vi "main.vi"() -> ()   [LabVIEW 2024]
doc: "Use this template to build a producer/consumer design pattern with events to produce queue items. Use this design pattern instead of the User Interface Event Handler pattern for user interfaces when you want to execute code asynchronously in response to an event without slowing the user interface responsiveness."
uses:
  controls/type.eng.settings.ctl
  controls/UiStepBuilder.ctl
  controls/type.step-builder.ctl
  controls/UiProcHeader.ctl
  controls/Ui.nrt.flow-panel.ctl
  controls/UiNutritionFlowElement.ctl
  controls/UiScheduleTimestamp.ctl
  controls/typeEnv.ctl
  controls/type.StepFunction.ctl
  controls/typeXyPoint.ctl
  controls/type.address.ctl
  controls/enum.io.type.ctl
  controls/enum.io.mode.ctl
  controls/IONode.ctl
  controls/type-io-map-do.ctl
  controls/type-io-map-di.ctl
  controls/type-io-map-ai.ctl
  controls/type-snapshot.ctl
  controls/enum-io-sort-type.ctl
  controls/wind-dir-view.ctl
  controls/windows-panel.ctl
  controls/irr-panel.ctl
  controls/pbr-func-def.ctl
  controls/eng-serial-log.ctl
  controls/cluster-com-log.ctl
  controls/state-engine.ctl
  controls/state-logger.ctl
  controls/enum.io-interface.ctl
  controls/enum-com-log.ctl
  controls/enum-q-sched.ctl
  controls/enum.report-filter.ctl
  controls/typePathSelector.ctl
  controls/ini-key.ctl
  controls/typeProcVarientName.ctl
  controls/UiNutritionPanel.ctl
  controls/enumVarCtrlIO.ctl
  controls/type.eng-call.proc-insert.ctl
  controls/type.eng.proc.isrunning.ctl
  controls/eng-call-do-by-name.ctl
  controls/cluster-q-sched.ctl
  <vilib>/Utility/error.llb/DialogType.ctl
  <vilib>/Utility/miscctls.llb/LVPointTypeDef.ctl
  <vilib>/Utility/miscctls.llb/LVDateTimeRec.ctl
  controls/rio-rx-enum.ctl
  controls/type.eng.log-cluster.ctl
  controls/typeCmdPostStepFunc.ctl
  controls/typeEngineLogCluster.ctl
  VIs/Polymorphics/variantCtrlString.vi
  VIs/proc.util.validateParamExist.vi
  <vilib>/Utility/error.llb/Trim Whitespace.vi
  <vilib>/Utility/error.llb/Trim Whitespace One-Sided.vi
  globals/globals-engine.vi
  <vilib>/Utility/libraryn.llb/Create Directory Recursive.vi
  <vilib>/Utility/config.llb/Read Key (String).vi
  VIs/util.error.create.vi
  <vilib>/Utility/config.llb/Read Key (Double).vi
  <vilib>/Utility/config.llb/Read Key (I32).vi
  VIs/util-address-builder.vi
  VIs/util.DO.ToString.vi
  VIs/Polymorphics/io.command-builder.vi
  VIs/Polymorphics/io.command-builder.DO.vi
  VIs/Polymorphics/io.command-builder.AI.vi
  VIs/Polymorphics/io.command-builder.DI.vi
  <vilib>/Utility/config.llb/Write Key (String).vi
  <vilib>/Utility/config.llb/Write Key (Double).vi
  <vilib>/Utility/config.llb/Write Key (I32).vi
  controls/typeIniFileSection.ctl
  <vilib>/Utility/file.llb/Read Delimited Spreadsheet (DBL).vi
  <vilib>/Utility/config.llb/NI_LVConfig.lvlib
  <vilib>/Instr/_visa.llb/VISA Find Search Mode.ctl
  <vilib>/Utility/file.llb/Write Delimited Spreadsheet (DBL).vi
panel:
  out "clock 3":string="12:34:56"
  out "COM Size":i64 format="IOs: %d"
  out "COM FIFO":i32 format="QCom: %d"
  out "LOG FIFO 2":i32 format="QLog: %d"
  out "ENG FIFO 2":i32 format="QEng: %d"
  in  "Cluster":cluster{"MAIN":bool, "I/O":bool, "ADMIN":bool}
  out "DayNight":bool
  in  "ENG ms ctrl 28":i32=300 caption="Runtime Interval" format="Runtime:  %d [ms]"
  in  "ENG ms ctrl 15":i32=300 caption="Runtime Interval" format="Runtime:  %d [ms]"
  in  "ENG ms ctrl 14":i32=300 caption="Runtime Interval" format="Runtime:  %d [ms]"
  in  "ENG ms ctrl 13":i32=300 caption="Runtime Interval" format="Runtime:  %d [ms]"
  in  "ENG ms ctrl 12":i32=300 caption="Runtime Interval" format="Runtime:  %d [ms]"
  in  "ENG ms ctrl 11":i32=300 caption="Runtime Interval" format="Runtime:  %d [ms]"
  in  "ENG ms ctrl 10":i32=300 caption="Runtime Interval" format="Runtime:  %d [ms]"
  in  "ENG ms ctrl 9":i32=300 caption="Runtime Interval" format="Runtime:  %d [ms]"
  in  "ENG ms ctrl 8":i32=300 caption="Runtime Interval" format="Runtime:  %d [ms]"
  in  "Admin Panel":bool
  out "Waveform Chart":dbl(graph)
  out "User messages":string
  out "error out":errorcluster
  in  "Timer Reset?":bool
  out "userName":string="USER"
  out "projectName":string="NAME"
  in  "ENV":T1=enum."ENV.TEST.SINGLE-02"
  out "clock":string="12:34:56"
  in  "Enable Report":bool
  in  "Tab Control 2":T2(tab)
  in  "EngLogClear":bool
  out "Collected Reports":string
  out "Collected Reports 2":string
  in  "VISA REPORT":T4={"visa report"=[["Range", "High", "Low", "25", "FULL"], ["", "", "", "", ""], ["", "", "", "", ""], ["", "", "", "", ""], ["", "", "", "", ""], ["", "", "", "", ""], ["", "", "", "", ""], ["", "", "", "", ""], ["", "", "", "", ""]], "RIO Address"=0, "IOtype"=enum."AI", "VISA Report En"=FALSE, "Clear"=FALSE, "Only Errors?"=FALSE} {"RIO Address" min=-1 max=31 step=1 format="RIO: %02d"}
  out "SelectedPath":path
  out "case":T5
  in  "Clk Simulator":timestamp format="%<%x %.1X>T"
  in  "Simulate Clock Reset":bool
  out "Clock Simulation":bool
  in  "Time Addition":dbl
  out "AI":dbl[][](array[numeric]) format="%#.1f"
  in  "Calib?":bool
  out "SCHED":i32 format="%.3p"
  out "Waveform Chart 3":dbl(graph)
  out "GuiLog":i32 format="%#.3p"
  out "Eng":i32 format="%#.3p"
  out "Event":i32 format="%#.3p"
  out "ComLog":i32 format="%.3p"
  out "Schedulers":cluster{"Proc Name":string, "Time":timestamp}[](array[cluster]) {"Time" format="%<%H:%M:%S>T"}
  out "Report General":T7(array[cluster]) {"clk" format="%#.1f"}
  in  "Log Clear":bool
  in  "Proc Name":string(combo)
  in  "DO Set by Addr":T9 {"ADDR" format="%04d"}
  in  "DO Set by Name":T10={"State"=FALSE, "Name"="Name...", "Timeout [s]"=8, "Send"=FALSE}
  in  "SerialPort":refnum<visa-resource-name>="COM12"
  in  "MenuRuntime":T11={"Run"=FALSE, "Step"=FALSE, "Load"=FALSE, "Status"=FALSE, "Unload"=FALSE, "Reload"=FALSE, "Stop"=FALSE, "ProcedureReload"=FALSE, "ProcedureStep"=FALSE, "ProcedureSelect"="set-dout", "ProcedureRun"=FALSE}
  out "Simulated":string[](array[string])
  in  "ProjectSettings":T12={"Project Name"="Yogiland", "Latitude"=0.0, "Longitude"=0.0, "TimeZone"=0, "userName"="Yogiland"} {"Longitude" format="%#.6g"; "Latitude" format="%#.6g"}
  out "RIO Snapshots":T13[](array[typedef]) {"Dports" format="%08x"}
  in  "Tab Main":enum32{"MAIN", "I/O", "ADMIN"}(tab)
  in  "Button":bool
  in  "Section":string(combo)
  in  "Tab NTR":T14(tab)
  in  "NTR Flowchart":T15={"WASH_IN"={"boolean"=FALSE, "Message"="25/150"}, "EC"={"boolean"=TRUE, "Message"="L Alarm"}, "PH"={"boolean"=TRUE, "Message"="Low"}, "ORP"={"boolean"=TRUE, "Message"="Range"}, "W_TEMP"={"boolean"=TRUE, "Message"="25"}, "W_LEVEL"={"boolean"=TRUE, "Message"="FULL"}, "ALFA1"={"boolean"=TRUE, "Message"="60/60"}, "BETA1"={"boolean"=TRUE, "Message"="25/60"}, "ALFA2"={"boolean"=FALSE, "Message"="0/0"}, "BETA2"={"boolean"=FALSE, "Message"="0/0"}, "ACID"={"boolean"=FALSE, "Message"="0/60"}, "BASE"={"boolean"=FALSE, "Message"="0/50"}, "WATER"={"boolean"=FALSE, "Message"="0/150"}, "WASH_OUT"={"boolean"=FALSE, "Message"="ss"}, "UNIT"={"boolean"=FALSE, "Message"="0"}, "ORPMIX"={"boolean"=FALSE, "Message"="0/150"}}
  out "ntr.status-table":string[][](table)=[["Range", "High", "Low", "25", "FULL"], ["", "", "", "", ""], ["", "", "", "", ""], ["", "", "", "", ""], ["", "", "", "", ""], ["", "", "", "", ""], ["", "", "", "", ""], ["", "", "", "", ""], ["", "", "", "", ""]]
  out "NTR Status":string="Nutrition Status: Processing Unit "
  in  "ntrGraphPeriod":T18 {"lastDays" format="Last %d Days"; "Time range"."Start" format="From: %<%d/%m/%y>T"; "Time range"."End" format="To: %<%d/%m/%y>T"}
  out "Nutrition Sensor Graph":cluster{"X":dbl[], "Y":dbl[]}(graph)
  out "EC 3":cluster{"X":dbl[], "Y":dbl[]}(graph)
  in  "ntrDosepumpSelect":string(combo)
  in  "ntrInputSelect":string(combo)
  in  "Irrigation status":string="Irrigation Status"
  out "Solar Elevation Graph":waveform(dbl)(graph)
  in  "UiProjectSettings":T19 {"Longitude" format="%#.6g"; "Latitude" format="%#.6g"}
  in  "GoToCam 2":bool
  in  "GoToCam":bool
  in  "Cluster 2":T20
  in  "camera":u16(ring) items=["Camera 1", "Camera 2"]
  in  "start":T17 caption="Open" format="%<%H:%M>T"
  out "last":T17 caption="Open" format="Last Harvest %<%H:%M:%S %d/%m/%y>T"
  in  "PRBmenu":cluster{"Harvest":bool, "SANI":bool}
  in  "PbrView 2":T21 {"Unit Storage"."col" scale=0.0..1.0; "Unit Storage"."?" scale=0.0..1.0; "Unit Storage"."?" scale=0.0..1.0; "Unit Column"."col" scale=0.0..1.0; "Unit Column"."?" scale=0.0..1.0; "Unit Column"."?" scale=0.0..1.0; "Digester"."Digester 2" scale=0.0..10.0; "Digester"."Digester 1" scale=0.0..10.0; "BIO Mass Tank" scale=0.0..100.0; "Harvest\n Tank" scale=0.0..100.0}
  in  "pbr-proc-mode":enum16{"MANUAL", "AUTO"}(ring)
  in  "PBR Builder":T23(array[cluster])
  out "source":string
  in  "PBR_PLAY":cluster{"PLAY":bool, "PAUSE":bool, "STOP":bool}
  in  "PBR PROC":string(combo)
  in  "PBR":T24
  in  "Graph Panel":T25={"Time range"={"Start"=timestamp(0 s since 1904-01-01), "End"=timestamp(0 s since 1904-01-01)}, "lastDays"=3, "refresh"=FALSE} {"lastDays" min=1 max=99 step=1 format="%d Days"; "Time range"."Start" format="From: %<%d/%m/%y>T"; "Time range"."End" format="To: %<%d/%m/%y>T"}
  out "OutdoorStatus":T26
  out "indoorStatus":T27
  in  "Tab Control 3":T28(tab)
  out "Outdoor Tdry Graph":cluster{"X":dbl[], "Y":dbl[]}[](graph)
  out "RH":cluster{"X":dbl[], "Y":dbl[]}[](graph)
  out "UV Graph":cluster{"X":dbl[], "Y":dbl[]}(graph)
  in  "UVAccHistoryDays":i8=3
  out "UV_ACC":cluster{"X":dbl[], "Y":dbl[]}(graph)
  out "Waveform Chart 2":cluster{dbl, "UV Limit":dbl}(graph)
  in  "UvAccRefresh":bool
  out "WindSpeed":cluster{"X":dbl[], "Y":dbl[]}(graph)
  out "Wind Dir Panel":T29
  out "UV Acc.":dbl format="%#_3p"
  in  "Tab Auxi":T30(tab)
  in  "IRR Params":T31={"Day Time"={"Sunset"=timestamp(0 s since 1904-01-01), "Sunrise"=timestamp(0 s since 1904-01-01)}, "timeLimits"={"Irrigation"=0.0, "Nut./Water"=0.0}, "Calculated Timing"={"Irrigation Timeout"=timestamp(0 s since 1904-01-01), "Nutrients Timeout"=timestamp(0 s since 1904-01-01)}, "Irr Dosing Time"={"Nutrients"=0, "Water"=0, "Wash"=0}, "UV Limit "=0.0, "Dose Table"=[{"Enable"=FALSE, "output"="IRR_SEC1"}, {"Enable"=FALSE, "output"="IRR_SEC2"}, {"Enable"=FALSE, "output"="IRR_SEC3"}, {"Enable"=FALSE, "output"="IRR_SEC4"}, {"Enable"=FALSE, "output"="IRR_SEC5"}, {"Enable"=FALSE, "output"="IRR_SEC6"}], "Last Iteration"=timestamp(0 s since 1904-01-01), "UV Reduction Status"=FALSE, "UV Reduction"=0} {"UV Reduction" max=99 step=1 format="%d [%%]"; "timeLimits"."Nut./Water" format="%02.2f [hr]"; "timeLimits"."Irrigation" format="%02.2f [hr]"; "Day Time"."Sunrise" format="%<%H:%M:%S>T"; "Day Time"."Sunset" format="%<%H:%M:%S>T"; "Calculated Timing"."Nutrients Timeout" format="%<%H:%M:%S>T"; "Calculated Timing"."Irrigation Timeout" format="%<%H:%M:%S>T"; "UV Limit" format="%#.1p [J/m2]"; "Irr Dosing Time"."Wash" format="%d [s]"; "Irr Dosing Time"."Water" format="%d [s]"; "Irr Dosing Time"."Nutrients" format="%d [s]"; "Last Iteration" format="%<%X %x>T"}
  in  "WinView":T32 {"EastSideView" scale=0.0..100.0; "WestSideView" scale=0.0..8.0; "EastPosition" max=12; "WestPosition" max=12}
  in  "AuxiliaryList":T33(array[cluster]) {"Period" format="Period [s]: %d"; "Pulse" format="Pulse [s]: %d"}
  in  "NTR Panel":cluster{"CloseAll":bool}
  in  "RFS Enable Table":bool
  in  "RFS Enable Table":T34
  in  "RFS Cycles Set":bool
  in  "RFS Cycles":u16
  out "RFS Cycles":u16
  in  "RFS Cycles Get":bool
  out "RFS Status":string
  in  "RFS SetX1":bool
  in  "TableIndex":u8 max=7 step=1 format="Table: %d"
  in  "RFS SetX8":bool
  in  "RFS Delays":T35
  in  "RFS Address":u8 format="Address: %d"
  out "RFS Cycles Table":T36
  out "elements":cluster{"case":T5, "data":variant}[](array[cluster])
  in  "Tab IO":enum32{"Map", "Editor", "Calibration"}(tab)
  in  "Clear Virtuals":bool
  in  "IO Map Take Snapshot":bool caption="Take Snapshop"
  out "RIO List":cluster{"Address":u8, "Connected":bool}[](array[cluster]) {"Address" format="%02d"}
  in  "Show Undefined":bool
  out "IO Map AI Count":i32
  out "IO Map DI Count":i32
  out "IO Map DO Count":i32
  in  "IO Map DO":T37[](array[typedef]) caption="Digital Outputs" {"ADDR" format="%04d"}
  in  "IO Map AI":T39[](array[typedef]) caption="Analog Inputs" {"ADDR" format="%04d"}
  in  "IO Map DI":T40[](array[typedef]) caption="Digital Inputs" {"ADDR" format="%04d"}
  in  "IO Map Snapshot Enable":bool caption="Auto Snapshop Enable"
  in  "IO Search Map":T41={"By Name"="", "By Tag"="Tags...", "By Address"=0} caption="Search by Name | Tag | Address" {"By Address" min=-1 max=31 step=1 format="RIO: %02d"}
  in  "IO Search Map Refresh":bool
  in  "TimerSec":dbl=5.0 format="%#.1f"
  out "downcount[sec]":dbl format="%#.1g"
  in  "Simulators":cluster{"Input ":string, "Value":string}[](array[cluster])
  in  "IO Map VL":T42[](array[typedef]) caption="Virtual Channels" {"calibration"."Y" format="%#.3f"; "calibration"."X" format="%#.3f"; "ADDR" format="%04d"}
  out "IO Map VL Count":i32
  in  "IO Conf view":enum16{"Show All", "Search"}(ring)
  in  "IOconf Sort":T44
  in  "IO Search Conf":T45={"ADDR"=-1, "Label"="", "Type"=enum."Type", "Mode"=enum."Mode", "Tags"=""} {"ADDR" min=-1 max=99 format="RIO: %02d"}
  in  "IO Conf":T46(array[cluster]) {"calibration"."Y" format="%#.3f"; "calibration"."X" format="%#.3f"; "ADDR" format="%04d"}
  in  "IO List":cluster{"save":bool, "loadCsv":bool}
  in  "New Element":T42={"ADDR"=0, "Label"="Name", "Type"=enum."DI", "Mode"=enum."RIO", "Value"="Value", "Tags"="Tags", "calibration"=[]} {"calibration"."Y" format="%#.3f"; "calibration"."X" format="%#.3f"; "ADDR" format="%04d"}
  in  "IO Add New":bool
  out "size":i32 format="Count: %d"
  out "Value (Y)":dbl
  out "Raw (X)":dbl
  in  "IO calib save":bool
  in  "IO calib select":string(combo)
  in  "XyPairs":T43[](array[typedef]) {"Y" format="%#.3f"}
  out "error":errorcluster
  out "Chart":cluster{"unCalibrated":u16, "Value out":dbl}(graph)
  in  "Tab Control":enum32{"Builder", "Snapshot", "Settings"}(tab)
  in  "BuilderMenu":T47
  in  "UiBuildProcHead":T48={"Procedure Name"="MyProcExample", "Running"=TRUE, "tags"="MyProcExample"}
  in  "Loaded Proc Path":string[](array[string])
  in  "UiBuildSteps":T49[](array[typedef])
  in  "File path":path
  out "UiBuildSteps 2":T49[](array[typedef])
  in  "Proc Select 2":string(combo)
  out "Serial Log Size":i32
  out "COM Snapshot":T51[](array[typedef])
  in  "Snapshot Size":i64=1000
  in  "COM":bool
  in  "filter":T52={"Status"=0, "Date"="", "Caller"="", "Type"="", "IOname"="", "Calib"="", "Uncalib"="", "Vsdt"="Vsdt", "StatusMsg"=""}
  out "Serial Record(s)":T53[](array[typedef]) {"IOnode"."calibration"."Y" format="%#.3f"; "IOnode"."calibration"."X" format="%#.3f"; "IOnode"."ADDR" format="%04d"}
  out "App Started at":timestamp format="%<%x %.3X>T"
  out "Loaded":cluster{"Procedure":variant[]}[](array[cluster]) caption="Loaded Procedures"
  in  "ENG ms":i32=-1 caption="Interval"
  in  "Title Bar Visible":bool
  in  "ENG ms ctrl":i32=300 caption="Runtime Interval" format="Runtime:  %d [ms]"
  in  "EVENT ms":i32=100 format="%d [ms]"
  out "Type":u8 format="%.0x"
  out "Address":u8 format="%.0x"
  in  "read buffer":string
  out "Command Payload":string
  out "AI uncalib out":u16
  out "AI out":dbl
  out "Data Size":u8
  out "GUI Engine Errors":errorcluster[](array[cluster])
  out "Record Engine Errors":errorcluster[](array[cluster])
  out "VM Engine Errors":errorcluster[](array[cluster])
  out "Scheduler Engine Errors":errorcluster[](array[cluster])
  # "Outoor"
  # "Indoor"
  # "UV Accumulator"
  # "Nutrition"
  # "Nutrition History"
  # "Nursery"
  # "Camera Robot"
  # "PBR"
  # "- Fully Open"
  # "- Fully Close"
  # "W"
  # "E"
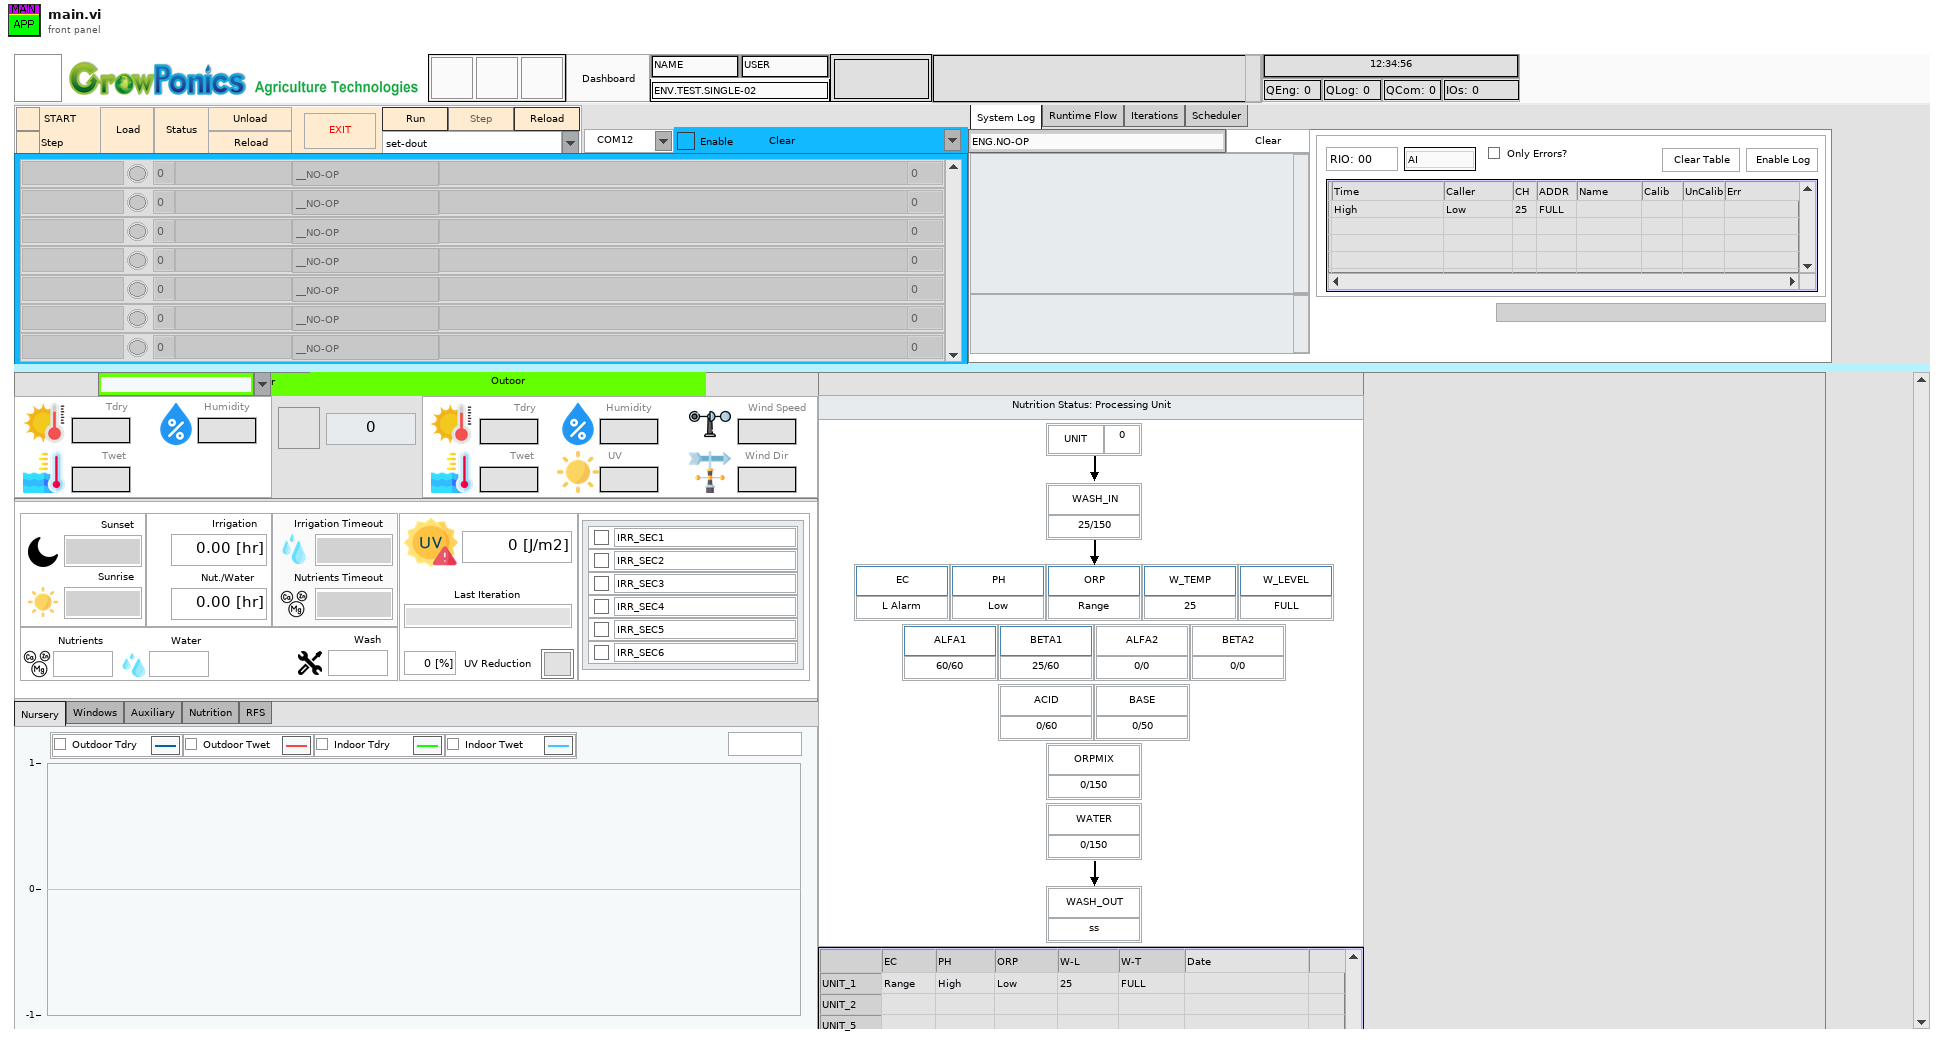
[diagram p1: front panel]
types:
  T1 = typedef "typeEnv.ctl" = enum16{"ENV.PRODUCTION", "ENV.TEST.NO-HW", "ENV.TEST.SINGLE-01", "ENV.TEST.SINGLE-02", "ENV.TEST.SINGLE-02 AI 0", "ENV.TEST.SINGLE-03"}
  T2 = enum32{"System Log", "Runtime Flow", "Iterations", "Scheduler"}
  T3 = typedef "enum.io.type.ctl" = enum16{"Type", "DI", "DO", "AI", "AO", "VL", "BUF"}
  T4 = cluster{"visa report":string[][], "RIO Address":i32, "IOtype":T3, "VISA Report En":bool, "Clear":bool, "Only Errors?":bool}
  T5 = typedef "state-engine.ctl" = enum16{"ENG.NO-OP", "ENG.START", "ENG.STOP", "ENG.EXECUTE", "ENG.STATUS", "ENG.EXTERNAL-CALL", "ENG.INIT", "ENG.INIT.VARS", "ENG.INIT.SERIAL", "ENG.LOAD", "ENG.LOAD.SINGLE", "ENG.LOAD.MODULE", "ENG.LOAD.RELOAD", "ENG.LOAD.UNLOAD", "ENG.IO.LOAD", "ENG.IO.SAVE", "ENG.PROC.RELOAD-BY-NAME", "ENG.PROC.START", "ENG.PROC.STOP", "ENG.PROC.INSERT-STEPS", "ENG.PROC.ISRUNNING", "ENG.PROC.PRESET", "ENG.PROC.STATUS", "ENG.PRINT-USER-MSG", "ENG.RIO.SNAPSHOT", "ENG.RIO.AIN-SNAPSHOT-CALIB", "ENG.RIO.DOUT-BY-ADDR", "ENG.RIO.DOUT-BY-NAME", "ENG.RIO.RFS-DELAY-SET-X1", "ENG.RIO.RFS-DELAY-SET-X8", "ENG.RIO.RFS-CYCLES-SET", "ENG.RIO.RFS-CYCLES-GET", "ENG.RIO.RFS-ENABLE", "ENG.EXIT"}
  T6 = typedef "type.StepFunction.ctl" = enum16{"__NO-OP", "_DELAY_LOAD", "_DELAY_COMPARE", "_JUMP", "_COMPLETE", "_COMPARE", "_LOG_MESSAGE", "_LOG_LAST_REPORT", "_SCHEDULE", "_SCHEDULE_DAILY", "CLK_COMPARE", "PROC_START", "PROC_STOP", "PROC_LOAD", "PROC_COMPLETION_CHECK", "PROC_COMPLETION_LOAD", "_IO_READ", "_IO_READ_MANY", "_IO_WRITE", "_IO_WRITE_BY_REG", "_IO_GET_OUTPUT", "_OCS_CHECK", "_OCS_RECORD", "_GET_RH", "_GET_ACC_UV", "_GET_WD", "_GET_WS", "_REC_DELETE", "_REC_MOVE", "_REC_COPY", "_IRR_CHECK", "UNIT_CHECK", "UNIT_SAMPLE", "UNIT_DOSE"}
  T7 = cluster{"ErrorFlag":bool, "idx":i32, "Step Name":string, "Step Function":T6, "Report":string, "clk":dbl, "Step Name 2":string}[]
  T8 = typedef "type.address.ctl" = u16
  T9 = cluster{"State":bool, "ADDR":T8, "Timeout [s]":u8, "Send":bool}
  T10 = cluster{"State":bool, "Name":string, "Timeout [s]":u8, "Send":bool}
  T11 = cluster{"Run":bool, "Step":bool, "Load":bool, "Status":bool, "Unload":bool, "Reload":bool, "Stop":bool, "ProcedureReload":bool, "ProcedureStep":bool, "ProcedureSelect":string, "ProcedureRun":bool}
  T12 = typedef "type.eng.settings.ctl" = cluster{"Project Name":string, "Latitude":dbl, "Longitude":dbl, "TimeZone":i32, "userName":string}
  T13 = typedef "type-snapshot.ctl" = cluster{"Address":u8, "DI":bool[], "status":errorcluster, "AI":dbl[], "Dports":u32, "AI RAW":dbl[]}
  T14 = enum32{"Nutrition Flow", "Nutrition", "Nursery Status", "Camera", "PBR", "PBR Programming"}
  T15 = typedef "Ui.nrt.flow-panel.ctl" = cluster{"WASH_IN":T16, "EC":T16, "PH":T16, "ORP":T16, "W_TEMP":T16, "W_LEVEL":T16, "ALFA1":T16, "BETA1":T16, "ALFA2":T16, "BETA2":T16, "ACID":T16, "BASE":T16, "WATER":T16, "WASH_OUT":T16, "UNIT":cluster{"boolean":bool, "Message":string}, "ORPMIX":T16}
  T16 = typedef "UiNutritionFlowElement.ctl" = cluster{"boolean":bool, "Message":string}
  T17 = typedef "UiScheduleTimestamp.ctl" = timestamp
  T18 = cluster{"Time range":cluster{"Start":T17, "End":T17}, "lastDays":dbl, "refresh":bool}
  T19 = cluster{"Latitude":dbl, "Longitude":dbl, "TimeZone":i32}
  T20 = cluster{"Next Button":bool, "Previous Button":bool, "Up Button":bool, "Down Button":bool, "Home":bool}
  T21 = cluster{"Unit Storage":cluster{dbl, dbl, "col":dbl}, "Unit Column":cluster{dbl, dbl, "col":dbl}, "Ui_TANKOUT":bool, "Column":dbl, "Ui MAIN\nUi_COLOUT\nUi_PUMP":bool, "Digester":cluster{"Digester 1":dbl, "Digester 2":dbl}, "DO 4":bool, "Flow Out DI":bool, "BIO Mass Tank":dbl, "DO Membrane":bool, "MEDIUM":bool, "WATER":bool, "Ui_TANKIN":bool, "Harvest\n Tank":dbl, "HARVEST":bool}
  T22 = typedef "pbr-func-def.ctl" = enum16{"DELAY SEC", "SCHEDULE DAILY", "SENSE", "PROC START", "SET OUTPUT", "FINISH", "JUMP"}
  T23 = cluster{"Operation":T22, "Param":string, "uid":string}[]
  T24 = cluster{"LOAD":bool, "SAVE":bool, "COMPILE":bool, "SAVEAS":bool}
  T25 = cluster{"Time range":cluster{"Start":T17, "End":T17}, "lastDays":i8, "refresh":bool}
  T26 = cluster{"Tdry":string, "Twet":string, "UV":string, "Humidity":string, "Wind Speed":string, "Wind Direction":string}
  T27 = cluster{"Tdry":string, "Twet":string, "Humidity":string}
  T28 = enum32{"Temperature", "Humidity", "UV", "UV Acc", "Wind"}
  T29 = typedef "wind-dir-view.ctl" = cluster{"SE":bool, "SW":bool, "NE":bool, "NW":bool, "W":bool, "E":bool, "S":bool, "N":bool}
  T30 = enum32{"Nursery", "Windows", "Auxiliary", "Nutrition", "RFS"}
  T31 = typedef "irr-panel.ctl" = cluster{"Day Time":cluster{"Sunset":timestamp, "Sunrise":timestamp}, "timeLimits":cluster{"Irrigation":dbl, "Nut./Water":dbl}, "Calculated Timing":cluster{"Irrigation Timeout":timestamp, "Nutrients Timeout":timestamp}, "Irr Dosing Time":cluster{"Nutrients":u16, "Water":u16, "Wash":u16}, "UV Limit ":dbl, "Dose Table":cluster{"Enable":bool, "output":string}[], "Last Iteration":timestamp, "UV Reduction Status":bool, "UV Reduction":u8}
  T32 = typedef "windows-panel.ctl" = cluster{"EastPosition":u16, "WestPosition":u16, "Wind Direction":string, "CloseAll":bool, "WestSideView":u16, "EastSideView":u16, "Wind Speed":string, "confs":cluster{"Full Open [sec]":u16, "Full Close [sec]":u16, "Stages":u16}}
  T33 = cluster{"Source":string, "SourceStatus":bool, "Dest":string, "DestStatus":bool, "Pulse":u16, "Period":u16, "Proc Name":string}[]
  T34 = cluster{"[0]":bool, "[1]":bool, "[2]":bool, "[3]":bool, "[4]":bool, "[5]":bool, "[6]":bool, "[7]":bool}
  T35 = cluster{"Delay Y":u8, "Delay X1":u8, "Delay X2":u8, "Delay CT":u8}
  T36 = cluster{"[0]":u16, "[1]":u16, "[2]":u16, "[3]":u16, "[4]":u16, "[5]":u16, "[6]":u16, "[7]":u16}
  T37 = typedef "type-io-map-do.ctl" = cluster{"ADDR":T8, "Label":string, "Mode":T38, "Value":string, "State":bool}
  T38 = typedef "enum.io.mode.ctl" = enum16{"Mode", "RIO", "SIM"}
  T39 = typedef "type-io-map-ai.ctl" = cluster{"ADDR":T8, "Label":string, "Mode":T38, "Value":string}
  T40 = typedef "type-io-map-di.ctl" = cluster{"ADDR":T8, "Label":string, "Mode":T38, "State":bool, "Value":string}
  T41 = cluster{"By Name":string, "By Tag":string, "By Address":i32}
  T42 = typedef "IONode.ctl" = cluster{"ADDR":T8, "Label":string, "Type":T3, "Mode":T38, "Value":string, "Tags":string, "calibration":T43[]}
  T43 = typedef "typeXyPoint.ctl" = cluster{"X":dbl, "Y":dbl}
  T44 = typedef "enum-io-sort-type.ctl" = enum16{"Sort By Address", "Sort By Name"}
  T45 = cluster{"ADDR":i8, "Label":string, "Type":T3, "Mode":T38, "Tags":string}
  T46 = cluster{"ADDR":T8, "Label":string, "Type":T3, "Mode":T38, "Value":string, "Tags":string, "calibration":T43[]}[]
  T47 = cluster{"templateSave":bool, "templateLoad":bool, "procedureLoad":bool, "procedureSaveAs":bool, "procedureSave":bool, "procedureReload":bool}
  T48 = typedef "UiProcHeader.ctl" = cluster{"Procedure Name":string, "Running":bool, "tags":string}
  T49 = typedef "UiStepBuilder.ctl" = cluster{"Step Function":T50, "ParamString":string, "Step Label":string}
  T50 = typedef "type.step-builder.ctl" = enum16{"NO_OPERATION", "DELAY-JUMP", "DELAY", "JUMP", "COMPLETE", "SCHEDULER", "SCHEDULER_DAILY", "IRR-CHECK", "UNIT-CHECK", "UNIT-SAMPLE", "UNIT-DOSE", "LOG-REPORT", "LOG-MESSAGE", "IO-READ", "IO-READ-MANY", "IO-WRITE", "IO-COMPARE-OUT", "IO-COMPARE-IN", "PROC-START", "PROC-STOP", "PROC-LOAD", "PROC-IS-COMPLETED", "RECORD-MOVE", "GET-RH", "GET-UV", "GET-WD", "GET-WS", "OCS-CHECK", "OCS-RECORD"}
  T51 = typedef "eng-serial-log.ctl" = cluster{"Status":u32, "Date":string, "Caller":string, "Type":string, "IOname":string, "Calib":string, "Uncalib":string, "Vsdt":string, "StatusMsg":string}
  T52 = cluster{"Status":u32, "Date":string, "Caller":string, "Type":string, "IOname":string, "Calib":string, "Uncalib":string, "Vsdt":string, "StatusMsg":string}
  T53 = typedef "cluster-com-log.ctl" = cluster{"Caller":string, "IOnode":T42, "error":errorcluster, "dports":bool[], "AIN (calib)":dbl, "AIN (raw)":u16, "Times Stamp":timestamp, "Record File Path":path, "Visa Data":string}
  T54 = typedef "enum-q-sched.ctl" = enum16{"SCHED.INIT", "SCHED.REGISTER", "SCHED.EXIT"}
  T55 = typedef "enum-com-log.ctl" = enum16{"REC.NO_OP", "REC.INIT", "REC.EXIT", "REC.SERIAL", "REC.IO", "REC.FETCH", "REC.OPEN-FILE", "REC.REOPEN-FILE"}
  T56 = typedef "enum.io-interface.ctl" = enum16{"IO_VISA_WR-RD", "IO_VISA_OPEN", "IO_VISA_CLOSE", "IO_VISA_CLEAR"}
  T57 = typedef "state-logger.ctl" = enum16{"LOG.NO_OP", "LOG.INIT", "LOG.INIT.NTR-FLOW", "LOG.EXIT", "LOG.CATCH", "LOG.PARSE.OCS", "LOG.UPDATE.SELECTORS", "LOG.UPDATE.IRR", "LOG.SNAPSHOT.PROC", "LOG.SNAPSHOT"}
  T58 = enum32{"Invalid", "Standard", "Closed", "Hidden", "Minimized", "Maximized"}
  T59 = typedef "ini-key.ctl" = enum16{"INI.PROJECT_NAME", "INI.ENV", "INI.ENG.SERIAL", "INI.ENG.INTERVAL_MS", "INI.LOCAL.LONGITUDE", "INI.LOCAL.LATITUDE", "INI.LOCAL.TIMEZONE"}
  T60 = typedef "typePathSelector.ctl" = enum16{"DIR_PROCS", "DIR_CONFIG", "DIR_TEMPLATE", "DIR_IO_FILE", "DIR_RECORD", "DIR_LOG", "DIR_RUNTIME", "DIR_PRESET", "DIR_INI"}
  T61 = typedef "enum.report-filter.ctl" = enum16{"Read ALL", "Read Errors", "Collect", "ClearAll"}
  T62 = typedef "typeINIKey.ctl" = string
  T63 = typedef "typeIniFileSection.ctl" = string
  T64 = typedef "NI_LVConfig.lvlib/Config Data RefNum.ctl" = refnum<k1>
  T65 = typedef "UiNutritionPanel.ctl" = cluster{"Main":cluster{"Enable":bool, "WashTimes":cluster{"In":dbl, "Out":dbl}, "DailyActivityHours":cluster{"Begin Time":T17, "End Time":T17}[]}, "Water Dosing":cluster{"Water Dose":dbl, "Water Limit":dbl}, "EC Ranges":cluster{"H Alarm":dbl, "L Alarm":dbl, "Low":dbl}, "EC Dosing":cluster{"ALFA1 Dose":dbl, "ALFA1 Limit":dbl, "BETA1 Dose":dbl, "BETA1 Limit":dbl, "ALFA2 Dose":dbl, "ALFA2 Limit":dbl, "BETA2 Dose":dbl, "BETA2 Limit":dbl}, "PH Ranges":cluster{"H Alarm":dbl, "L Alarm":dbl, "High":dbl, "Low":dbl}, "PH Dosing":cluster{"ACID Dose":dbl, "ACID Limit":dbl, "BASE Dose":dbl, "BASE Limit":dbl}, "ORP Ranges":cluster{"H Alarm":dbl, "L Alarm":dbl, "Low":dbl}, "ORP Dosing":cluster{"MIX Dose":dbl, "MIX Limit":dbl}}
  T66 = enum16{"Always On", "Always Off", "Off While Running"}
  T67 = typedef "LVPointTypeDef.ctl" = cluster{"Horizontal":i16, "Vertical":i16}
  T68 = enum32{"Nutrition Flow", "Nutrition", "Nursery Status", "Camera", "PBR"}
  T69 = typedef "enumVarCtrlIO.ctl" = enum16{"IO Get By Key", "IO List Configs", "IO Add By Key", "IO Modify Value By Key", "IO Modify Calib By Key", "IO Modify ADDR By Key", "IO Modify Mode By Key", "IO Modify Type By Key", "IO Modify Name By Key", "IO Remove By Key", "IO Remove All"}
  T70 = cluster{"Device":i8, "Label":string, "Type":T3, "Mode":T38, "Tags":string}
  T71 = cluster{"State":bool, "Timeout":u16, "Name":string}
  T72 = enum8{"Enabled", "Disabled", "Disabled and Grayed Out"}
  T73 = cluster{"ADDR":u8, "Label":string, "Type":T3, "Mode":T38, "Tags":string}
  T74 = typedef "LVDateTimeRec.ctl" = cluster{"fractional second":dbl, "second":i32, "minute":i32, "hour":i32, "day of month":i32, "month":i32, "year":i32, "day of week":i32, "day of year":i32, "DST":i32}
  T75 = typedef "DialogType.ctl" = u16
  T76 = cluster{"ADDR":bool, "Label":bool, "Mode":bool, "Value":bool, "State":bool}[]
  T77 = cluster{"ADDR":bool, "Label":bool, "Mode":bool, "Value":bool, "State":bool}
  T78 = typedef "UiCompactReport.ctl" = cluster{"ErrorFlag":bool, "idx":i32, "Step Name":string, "Step Function":T6, "Report":string, "clk":dbl, "Proc":string}
  T79 = enum16{"Left Button", "Center Button", "Right Button", "Window Close"}
  T80 = typedef "rio-rx-enum.ctl" = u16
  T81 = enum32{"Bad", "Idle", "Run top level", "Running"}
  T82 = cluster{"Q-Log":refnum<queue>, "procQ":cluster{"data":variant, "Enum":T57}}
  T83 = typedef "cluster-q-sched.ctl" = cluster{"Proc Name":string, "Time":timestamp}
  T84 = typedef "type.eng.log-cluster.ctl" = cluster{"Procedure(post)":variant[], "Procedure(pre)":variant[], "Next State ":cluster{"CMD":T85, "data":variant}, "IsRunning":bool, "error in":errorcluster}
  T85 = typedef "typeCmdPostStepFunc.ctl" = enum16{"NEXT", "PREV", "JUMP", "STAY", "COMPLETE", "ENGCALL.PROC.START", "ENGCALL.PROC.STOP", "ENGCALL.PROC.COMPLETION-CHECK", "ENGCALL.PROC.INIT", "ERROR"}
  T86 = typedef "typeEngineLogCluster.ctl" = cluster{"Proc Name":string, "ProcPath":string, "Step Name":string, "Step Function":T6, "Step Index":i32, "Report":string, "clk":dbl, "error in":errorcluster, "Log Message":string, "Proc Module":string}
  T87 = typedef "typeProcVarientName.ctl" = enum16{"procNameID", "procModuleID", "procPath", "procIsRunning", "procIndex", "procModule", "procRegisterNumeric", "procRegisterString", "procReport", "procReportPrev", "procCLK", "procStepPointer", "procType"}
  T88 = typedef "wind-directions.ctl" = enum16{"N", "NE", "E", "SE", "S", "SW", "W", "NW"}
  T89 = cluster{"Irrigation Timeout":timestamp, "Fertiliztion Timeout":timestamp}
  T90 = enum16{"open", "replace", "create", "open or create", "replace or create", "replace or create with confirmation"}
  T91 = typedef "type.eng-call.proc-insert.ctl" = cluster{"ProcName":string, "instructions":variant[]}
  T92 = typedef "type.eng.proc.isrunning.ctl" = cluster{"callerProc":string, "procPointer":string}
  T93 = cluster{"operation":enum16{"START", "STOP"}, "procName":string}
  T94 = typedef "eng-call-do-by-name.ctl" = cluster{"State":bool, "Timeout":u16, "Name":string}
  T95 = cluster{"DataSize":u8, "Address":u8, "CMD":u8, "Table Index":u8, "Delay Y":u8, "Delay X1":u8, "Delay X2":u8, "Delay CT":u8}
  T96 = cluster{"DataSize":u8, "Address":u8, "CMD":u8, "Enable":u8}
  T97 = cluster{"DataSize":u8, "Address":u8, "CMD":u8, "Cycles":u16}
  T98 = cluster{cluster{"Procedure":variant[]}, "error":errorcluster}[]
  T99 = typedef "type.aux.ctl" = cluster{"Source":string, "SourceStatus":bool, "Dest":string, "DestStatus":bool, "Pulse":u16, "Period":u16, "Proc Name":string}
  T100 = typedef "VISA Find Search Mode.ctl" = u32
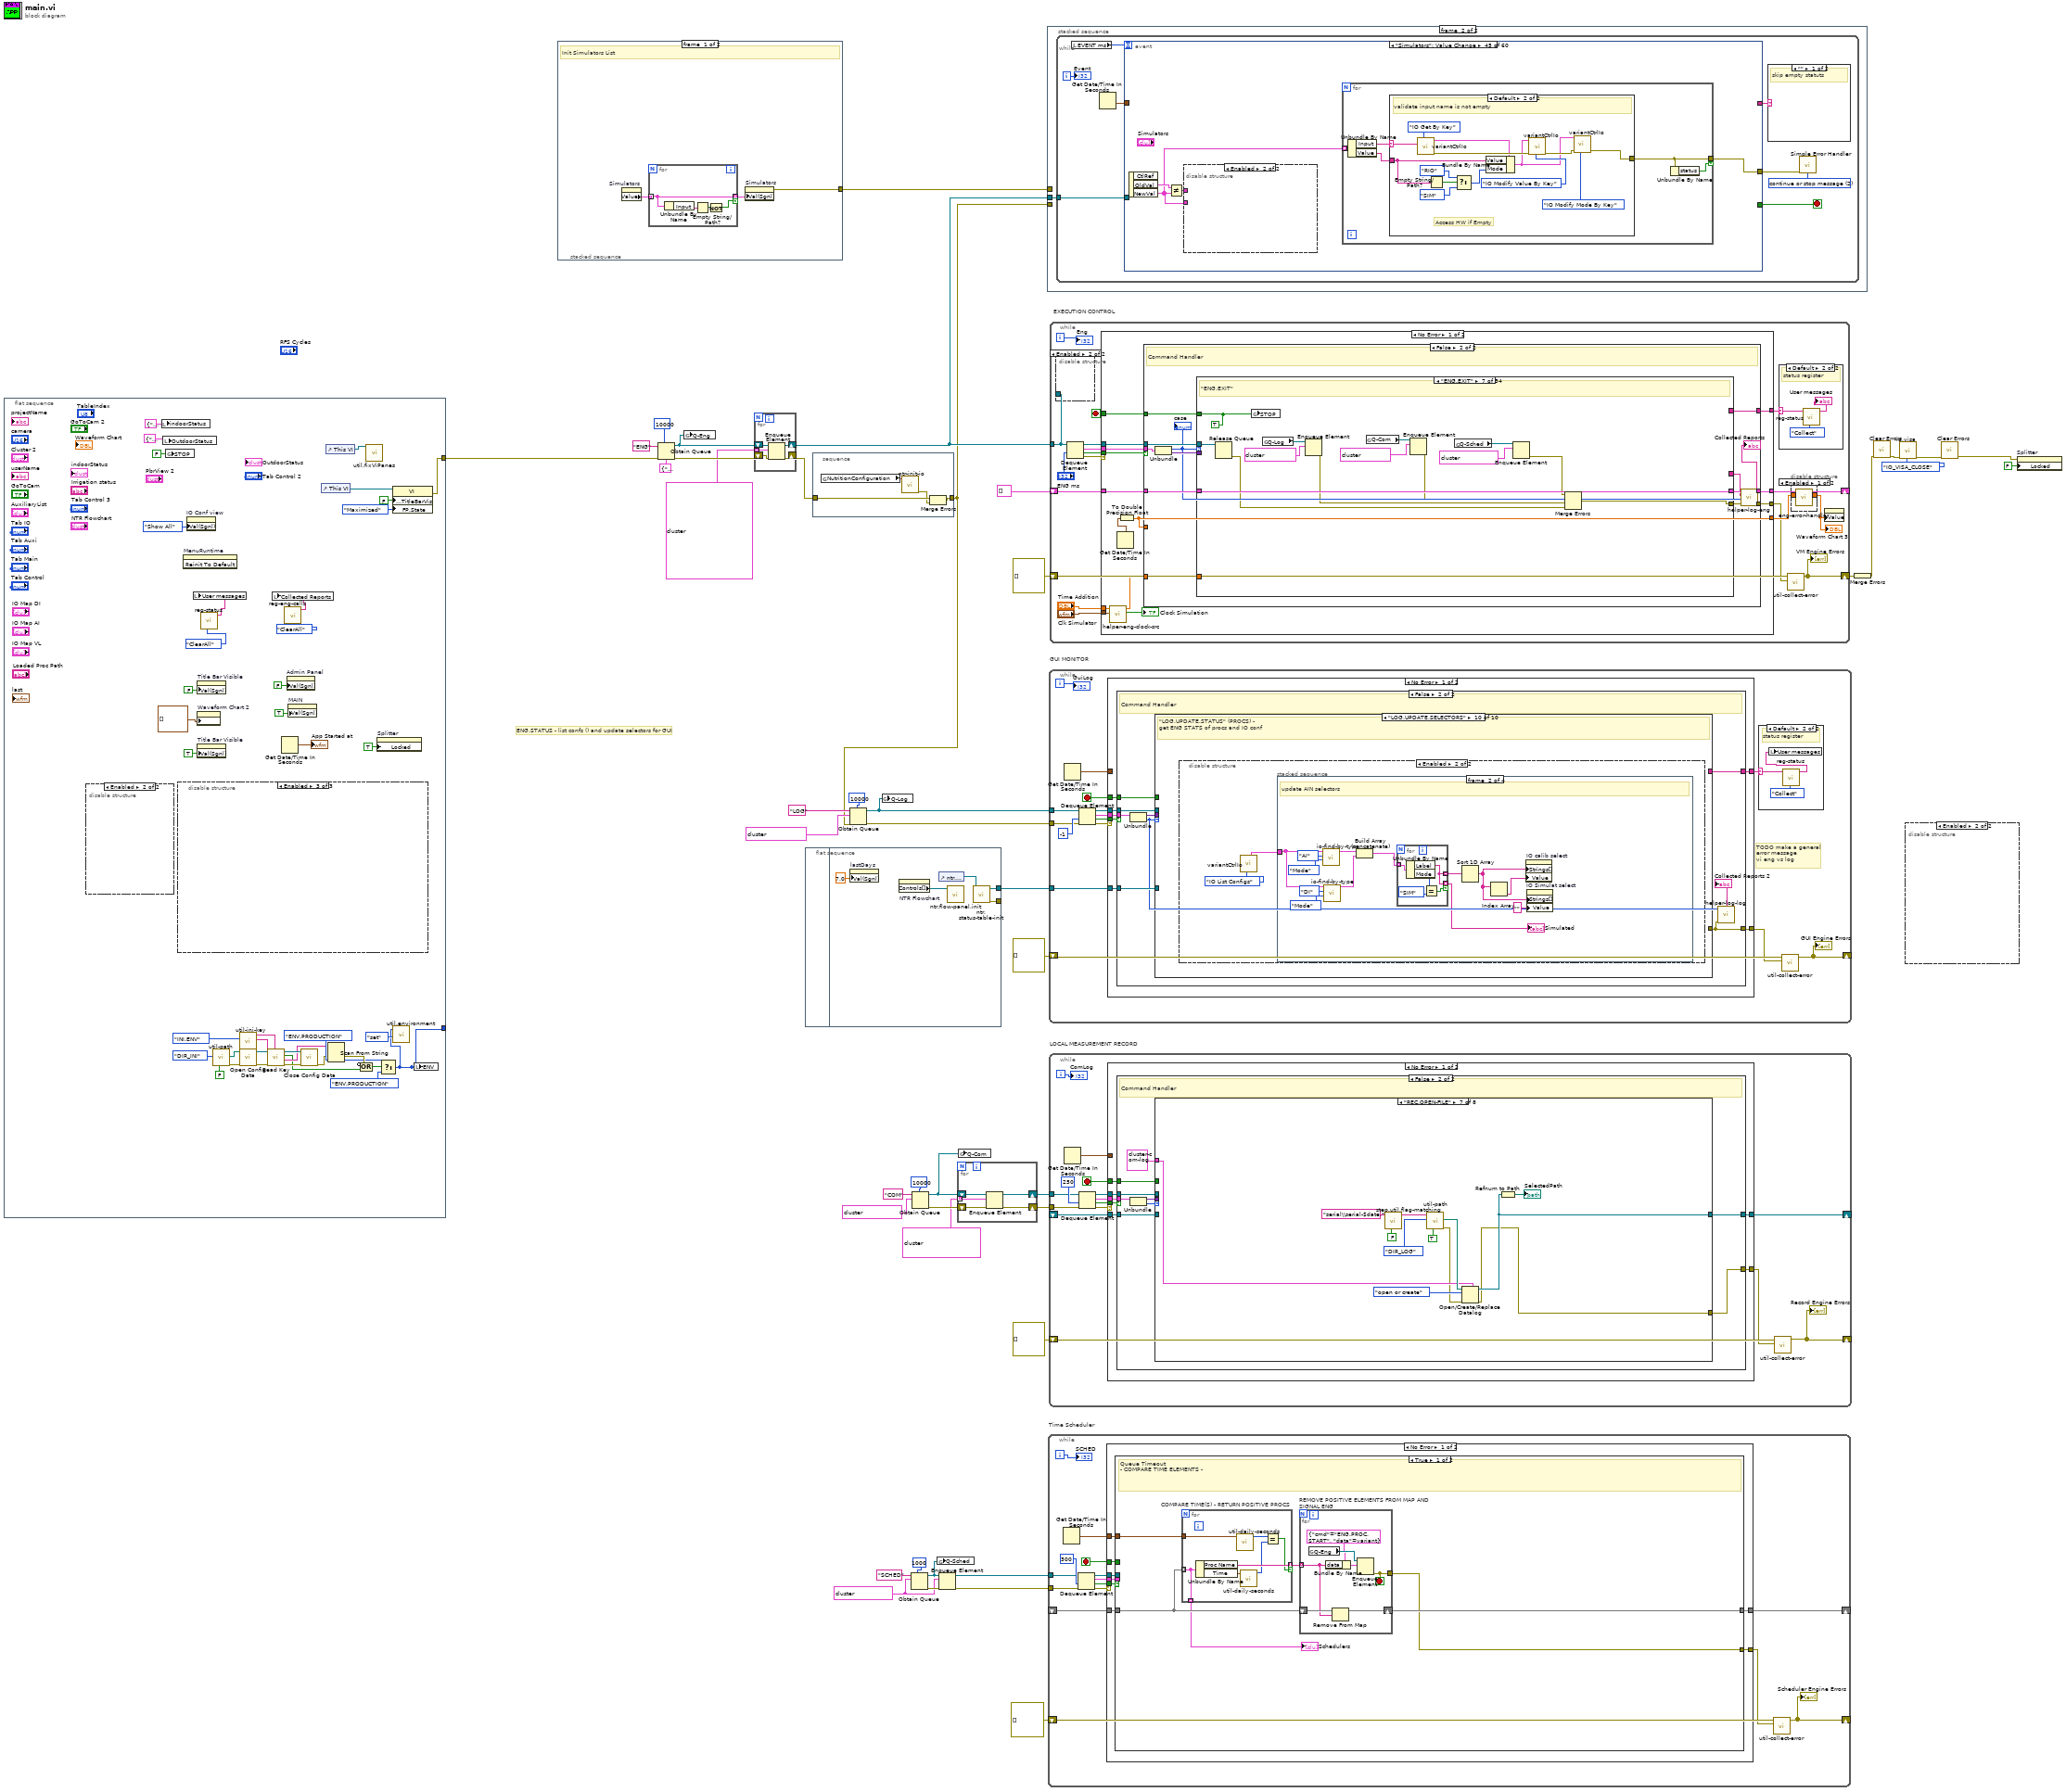
[diagram p0: block diagram]
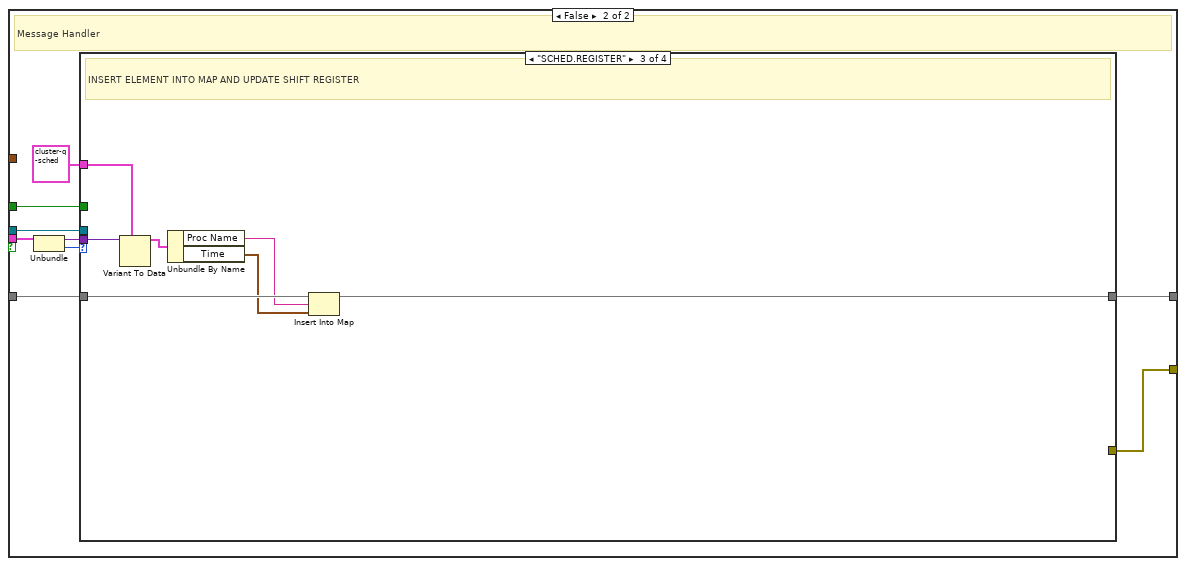
[diagram p2: hidden frame]
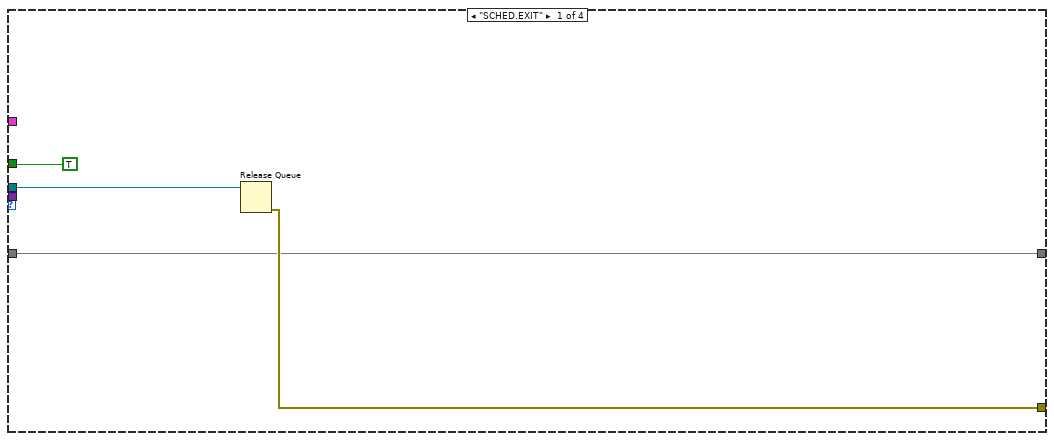
[diagram p3: hidden frame]
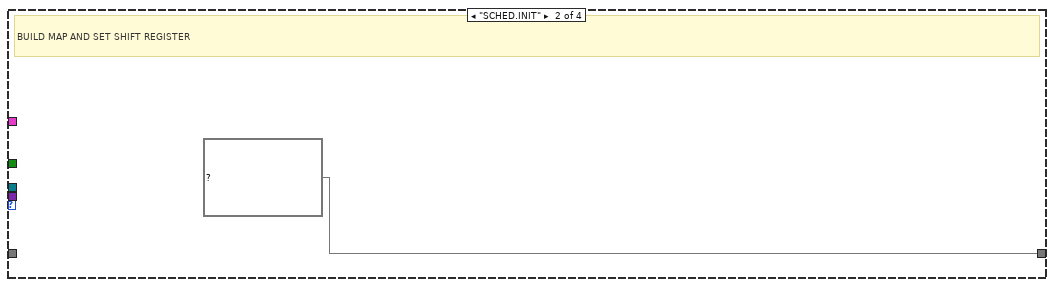
[diagram p4: hidden frame]
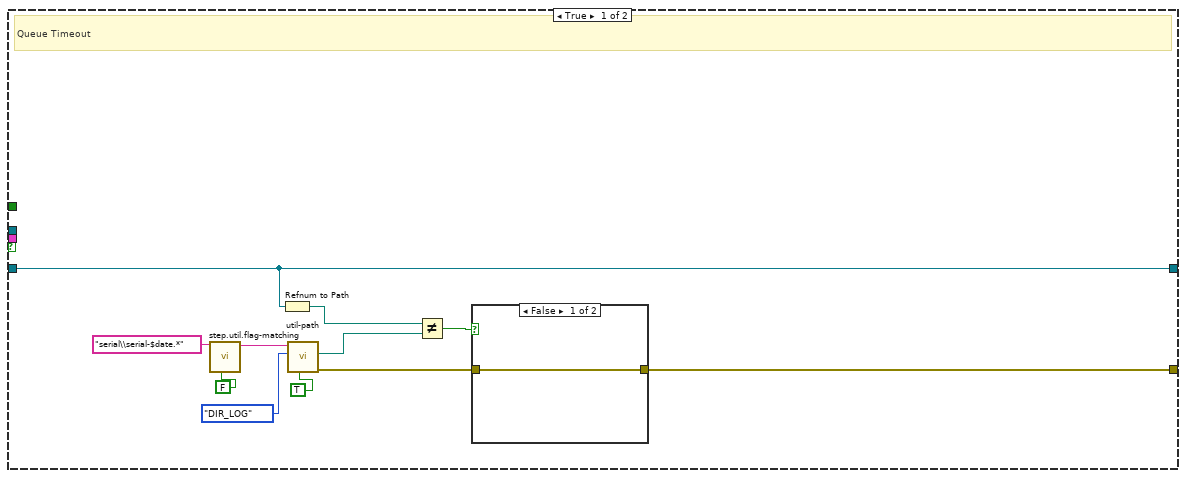
[diagram p8: hidden frame]
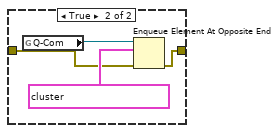
[diagram p9: hidden frame]
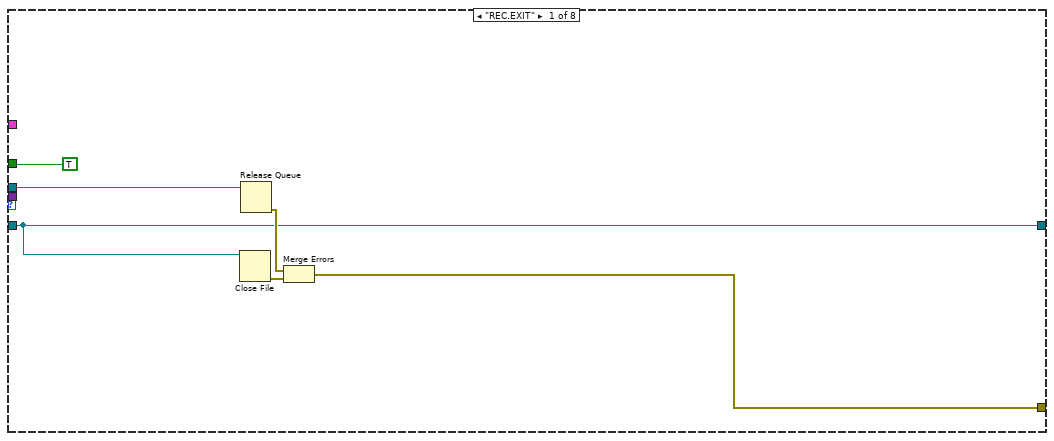
[diagram p10: hidden frame]
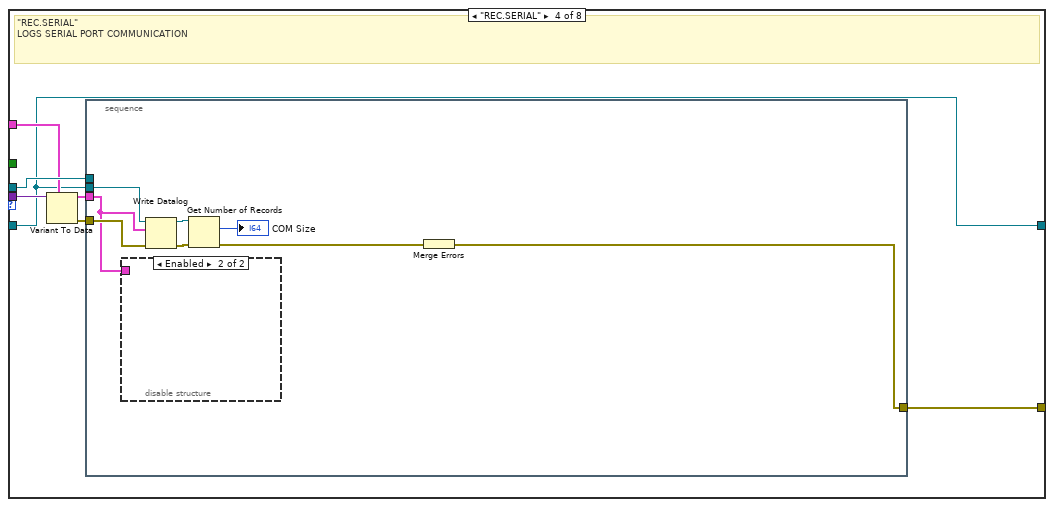
[diagram p13: hidden frame]
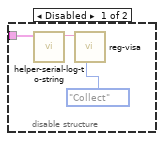
[diagram p14: hidden frame]
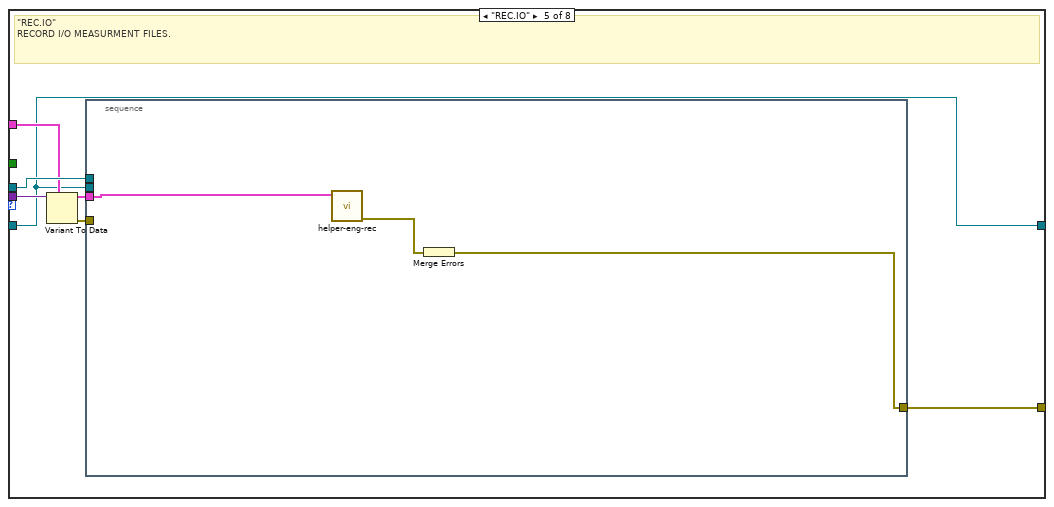
[diagram p15: hidden frame]
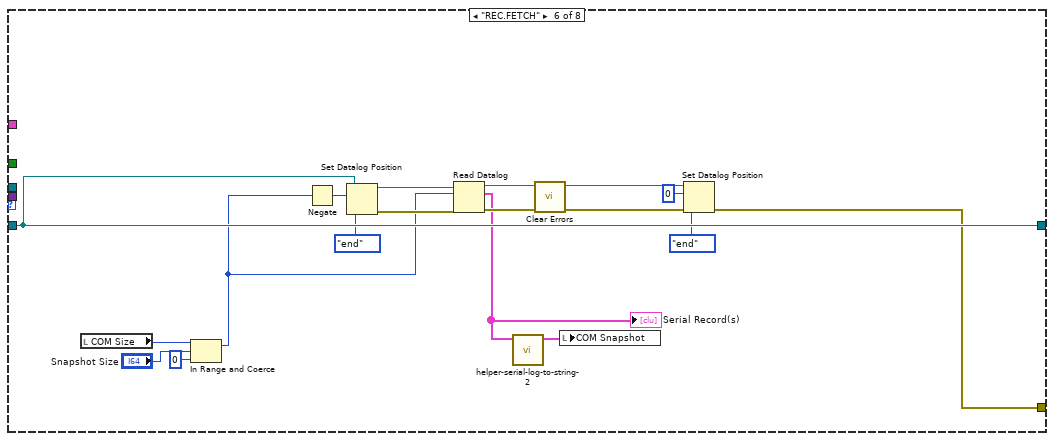
[diagram p16: hidden frame]
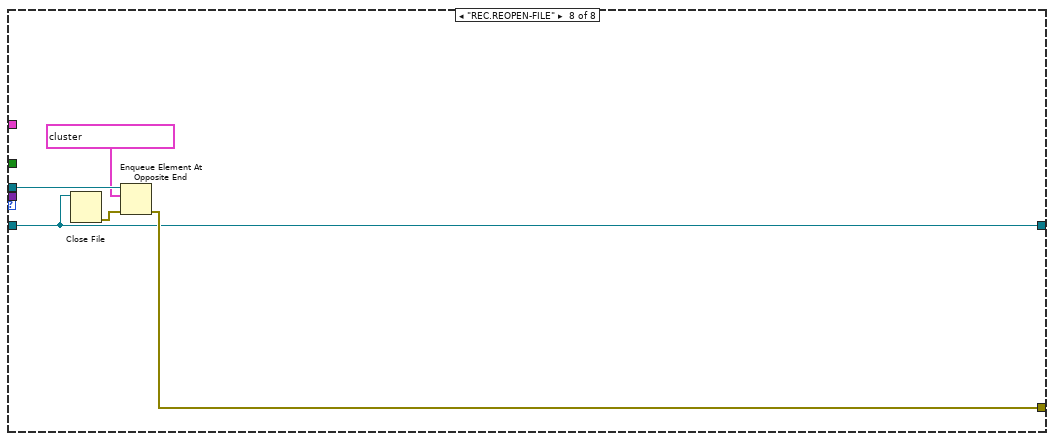
[diagram p17: hidden frame]
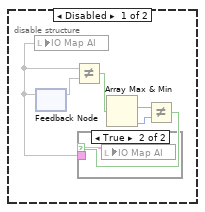
[diagram p19: hidden frame]
diagram:
  w1 = cluster{"data":variant, "Enum":T54} {"data"=variant, "Enum"=enum."SCHED.INIT"} ("procQ")
  # "ENG.STATUS - list confs () and update selectors for GUI"
  n1 = flat-sequence {
    tunnel: [w58] -> _
    tunnel: [w45] -> w15
    frame #0 {
      n2 = disable-structure shown="Enabled" {
        frame Disabled {
          # "Flows VIs"
          n3 = call "flow-IRR.vi"() -> ()  [unwired: 10 in, 2 out]
          n4 = call "flow-icc.vi"() -> ()  [unwired: 11 in, 1 out]
          n5 = call "flow-NTR.vi"() -> ()  [unwired: 11 in, 1 out]
        }
        frame Enabled {
        }
      }
      n6 = local write "indoorStatus"(T27 {"Tdry"="", "Twet"="", "Humidity"=""} ("indoorStatus")) -> ()
      n7 = local write "OutdoorStatus"(T26 {"Tdry"="", "Twet"="", "UV"="", "Humidity"="", "Wind Speed"="", "Wind Direction"=""} ("OutdoorStatus")) -> ()
      n8 = global write "globals-engine.vi" "STOP"(FALSE ("STOP")) -> ()
      n9 = disable-structure shown="Enabled" {
        frame Disabled {
          (unwired) cluster{"X":dbl[], "Y":dbl[]} {"X"=[], "Y"=[]} ("cluster")
          n10 = call-poly <vilib>:"Read Delimited Spreadsheet.vi"("file path (dialog if empty)"=path "C:/interface/file1.txt", "transpose? (F)"=TRUE) -> ("all rows"=w93:dbl[][])  [unwired: 8 in, 5 out]
          n11 = call-poly <vilib>:"Read Delimited Spreadsheet.vi"("file path (dialog if empty)"=path "C:/interface/file2.txt", "transpose? (F)"=TRUE) -> ("all rows"=w90:dbl[][])  [unwired: 8 in, 5 out]
          n12 = Index Array(array=w93) -> (element #1=w88:dbl[], element #2=w87:dbl[])  [unwired: 4 in]
          n13 = Index Array(array=w90) -> (element #1=w91:dbl[], element #2=w86:dbl[])  [unwired: 4 in]
          n14 = Bundle("all rows"=w88, "all rows"=w87) -> (w92:cluster{"all rows":dbl[], "all rows":dbl[]})  [unwired: 1 in]
          n15 = Bundle("all rows"=w91, "all rows"=w86) -> (w89:cluster{"all rows":dbl[], "all rows":dbl[]})  [unwired: 1 in]
          n16 = Build Array(w92, w89) -> ()  [unwired: 1 out]
        }
        frame Disabled {
          n17 = Build Array(T62 "VISA" ("section")) -> (w102:T62[])
          n18 = call "util.file.ini.vi"("Section"=T63 "SYSTEM" ("section"), "keys"=w102) -> ("values"=w101:string[])  [unwired: 7 in, 2 out]
          n19 = Index Array(array=w101) -> (element=w100:string)  [unwired: 1 in]
          n20 = property on="SerialPort" class="VISAName"("Val(Sgnl)"=w100) -> ()  [unwired: 2 in, 2 out]
        }
        frame Enabled {
        }
      }
      n21 = invoke on="MenuRuntime" class="Clust (strict)" method="Reinit To Default"() -> ()  [unwired: 3 in, 3 out]
      n22 = property on="IO Conf view" class="Enum (strict)"("Val(Sgnl)"=enum16{"Show All", "Search"}."Show All" ("Value (Signaling)")) -> ()  [unwired: 2 in, 2 out]
      n23 = property on="Title Bar Visible" class="Bool (strict)"("Val(Sgnl)"=FALSE ("Value (Signaling)")) -> ()  [unwired: 2 in, 2 out]
      n24 = property on="Waveform Chart 2" class="WFChart (strict)"("History Data"=cluster{"result string":dbl, "UV Limit":dbl}[] []) -> ()  [unwired: 2 in, 2 out]
      n25 = property on="Title Bar Visible" class="Bool (strict)"("Val(Sgnl)"=TRUE ("Value (Signaling)")) -> ()  [unwired: 2 in, 2 out]
      n26 = call "reg-status.vi"("Operation(Read)"=enum.report-filter."ClearAll") -> ("Collected Reports"=w81:string)  [unwired: 9 in, 1 out]
      n27 = local write "User messages"(w81) -> ()
      n28 = call "util-path.vi"("Create Folders?(F)"=FALSE, "Selected Folder (PROCS)"=typePathSelector."DIR_INI" ("Selected Folder (PROCEDURE_DIR)")) -> ("error out"=w67:errorcluster, "SelectedPath"=w69:path)  [unwired: 5 in, 3 out]
      n29 = call "util-ini-key.vi"("key"=ini-key."INI.ENV" ("input 1")) -> ("key"=w73:string, "section"=w74:string)  [unwired: 9 in]
      n30 = call <vilib>:"Open Config Data.vi"("error in (no error)"=w67, "configuration file path"=w69) -> ("error out"=w68:errorcluster, "refnum"=w70:T64)  [unwired: 7 in, 1 out]
      n31 = call-poly <vilib>:"Read Key.vi"("section"=w74, "error in (no error)"=w68, "key"=w73, "refnum"=w70) -> ("error out"=w71:errorcluster, "value"=w65:string, "found?"=w64:bool, "refnum out"=w72:T64)  [unwired: 4 in]
      n32 = Get Date/Time In Seconds() -> (seconds since 1Jan1904=→"App Started at":timestamp)
      n33 = call "reg-eng-calls.vi"("Operation(Read)"=enum.report-filter."ClearAll") -> ("Collected Reports"=w79:string)  [unwired: 9 in, 1 out]
      n34 = local write "Collected Reports"(w79) -> ()
      n35 = property on="Admin Panel" class="Bool (strict)"("Val(Sgnl)"=FALSE ("Value (Signaling)")) -> ()  [unwired: 2 in, 2 out]
      n36 = property on="MAIN" class="Bool (strict)"("Val(Sgnl)"=TRUE ("Value (Signaling)")) -> ()  [unwired: 2 in, 2 out]
      n37 = call <vilib>:"Close Config Data.vi"("error in (no error)"=w71, "refnum"=w72) -> ("error out"=w59:errorcluster)  [unwired: 8 in, 1 out]
      n38 = control-ref of="This VI"() -> (w54:refnum<vi>)
      n39 = control-ref of="This VI"() -> (w83:refnum<vi>)
      n40 = Scan From String(input string=w65, error in=w59, default 1=typeEnv."ENV.PRODUCTION" ("ENV in")) -> (error out=w63:errorcluster, output 1=w61:T1)  [unwired: 2 in, 2 out]
      n41 = Compound Arithmetic op=OR(invert w63, w64) -> (w62:bool)
      n42 = call "util.fixViPanes.vi"("VI in"=w83) -> ()  [unwired: 11 in]
      n43 = property on="Splitter" class="Splitter"("Locked"=TRUE ("Splitter Position Locked")) -> ()  [unwired: 2 in, 2 out]
      n44 = Select(t=w61, s=w62, f=typeEnv."ENV.PRODUCTION") -> (s? t:f=w58:T1)
      n45 = property class="VI"(reference=w54, "Front Panel.TitleBarVis"=FALSE ("Front Panel Window:Title Bar Visible"), "FP.State"=T58."Maximized" ("Front Panel Window:State")) -> (error out=w45:errorcluster)  [unwired: 1 in, 1 out]
      n46 = call "util.environment.vi"("Operation (Get)"=enum16{"get", "set"}."set", "ENV in"=w58) -> ()  [unwired: 8 in, 2 out]
      n47 = local write "ENV"(w58) -> ()
    }
  }
  n48 = stacked-sequence {
    tunnel: [w105 _] -> w26
    frame #0 {
      # "Init Simulators List"
      n49 = property on="Simulators" class="Arr (strict)"() -> ("Value"=w104:cluster{"Input ":string, "Value":string}[])  [unwired: 2 in, 2 out]
      n50 = for {
        tunnel: w104 -> [w109] mode=indexing
        tunnel: [w109] -> w103 mode=indexing if=w106
        n51 = Unbundle By Name(w109) -> ("Input"=w108:string)
        n52 = Empty String/Path?(string/path=w108) -> (empty?=w107:bool)
        n53 = Not(x=w107) -> (.not. x?=w106:bool)
      }
      n54 = property on="Simulators" class="Arr (strict)"("Val(Sgnl)"=w103) -> (error out=w105:errorcluster)  [unwired: 2 in, 1 out]
    }
    frame #1 {
    }
  }
  n55 = Obtain Queue(max queue size (-1, unlimited)=10000, name (unnamed)="ENG", element data type=cluster{"case":T5, "data":variant} {"case"=enum."ENG.NO-OP", "data"=variant} ("procQ"), error in (no error)=w15) -> (queue out=w40:refnum<queue>, error out=w44:errorcluster)  [unwired: 1 in, 1 out]
  n56 = global write "globals-engine.vi" "Q-Eng"(w40) -> ()
  n57 = for {
    tunnel: cluster{"cmd":T5, "data":variant}[] [{"cmd"=enum."ENG.STOP", "data"=variant}, {"cmd"=enum."ENG.INIT", "data"=variant}, {"cmd"=enum."ENG.IO.LOAD", "data"=variant}, {"cmd"=enum."ENG.LOAD", "data"=variant}, {"cmd"=enum."ENG.STATUS", "data"=variant}, {"cmd"=enum."ENG.START", "data"=variant}] ("typedefElement") -> [w110] mode=indexing
    shift-right: [w111] -> w10
    shift-left: w44 -> [w113]
    shift-right: [w112] -> w28
    shift-left: w40 -> [w114]
    n58 = Enqueue Element(queue=w114, element=w110, error in (no error)=w113) -> (queue out=w112:refnum<queue>, error out=w111:errorcluster)  [unwired: 1 in, 1 out]
  }
  n59 = flat-sequence {
    tunnel: [w118] -> _
    tunnel: [w117] -> w33
    frame #0 {
    }
    frame #1 {
      n60 = property on="lastDays" class="DigNum (strict)"("Val(Sgnl)"=7.0 ("Value (Signaling)")) -> ()  [unwired: 2 in, 2 out]
      n61 = property on="NTR Flowchart" class="Clust (strict)"() -> ("Controls[]"=w116:refnum<vi>[])  [unwired: 2 in, 2 out]
      n62 = control-ref of="ntr.status-table"() -> (w119:refnum<vi>)
      n63 = call "ntr.flow-panel.init.vi"("Controls in"=w116) -> ()  [unwired: 8 in, 3 out]
      n64 = call "ntr.status-table-init.vi"("Table in"=w119) -> ("error out"=w118:errorcluster, "Table out"=w117:refnum<vi>)  [unwired: 9 in]
    }
  }
  n65 = stacked-sequence {
    tunnel: [w121] -> w9
    tunnel: w10 -> [w122]
    frame #0 {
      n66 = global read "globals-engine.vi" "NutritionConfiguration"() -> (w123:T65[])
      n67 = call "ntr-init-io.vi"("NutritionConfiguration"=w123) -> ("error out"=w120:errorcluster)  [unwired: 10 in]
      n68 = Merge Errors(w122, w120) -> (w121:errorcluster)
    }
  }
  n69 = Obtain Queue(max queue size (-1, unlimited)=10000, name (unnamed)="LOG", element data type=cluster{"data":variant, "Enum":T57} {"data"=variant, "Enum"=enum."LOG.NO_OP"} ("procQ"), error in (no error)=w9) -> (queue out=w29:refnum<queue>, error out=w32:errorcluster)  [unwired: 1 in, 1 out]
  n70 = global write "globals-engine.vi" "Q-Log"(w29) -> ()
  n71 = Obtain Queue(max queue size (-1, unlimited)=1000, name (unnamed)="SCHED", element data type=w1) -> (queue out=w5:refnum<queue>, error out=w3:errorcluster)  [unwired: 2 in, 1 out]
  n72 = Obtain Queue(max queue size (-1, unlimited)=10000, name (unnamed)="COM", element data type=cluster{"data":variant, "Enum":T55} {"data"=variant, "Enum"=enum."REC.NO_OP"} ("procQ")) -> (queue out=w16:refnum<queue>, error out=w22:errorcluster)  [unwired: 2 in, 1 out]
  n73 = global write "globals-engine.vi" "Q-Sched"(w5) -> ()
  n74 = Enqueue Element(queue=w5, element=w1, error in (no error)=w3) -> (queue out=w4:refnum<queue>, error out=w2:errorcluster)  [unwired: 1 in, 1 out]
  n75 = for {
    tunnel: cluster{"data":variant, "Enum":T55}[] [{"data"=variant, "Enum"=enum."REC.OPEN-FILE"}] ("procQ") -> [w128] mode=indexing
    shift-right: [w126] -> w18
    shift-left: w16 -> [w127]
    shift-right: [w125] -> w17
    shift-left: w22 -> [w124]
    n76 = Enqueue Element(queue=w127, element=w128, error in (no error)=w124) -> (queue out=w126:refnum<queue>, error out=w125:errorcluster)  [unwired: 1 in, 1 out]
  }
  n77 = global write "globals-engine.vi" "Q-Com"(w16) -> ()
  n78 = stacked-sequence {
    tunnel: w28 -> [_ w131]
    tunnel: w9 -> [_ _]
    tunnel: w26 -> [_ _]
    frame #0 {
      n79 = To Time Stamp(1:0) -> (0:w129:timestamp)
      n80 = property on="start" class="AbsTime (strict)"("Value"=w129) -> ()  [unwired: 2 in, 2 out]
    }
    frame #1 {
      n81 = while {
        tunnel: w131 -> [w139]
        i -> [w136]
        stop <- w137 stop-if-true
        w135 = T75 2 items=["no dialog", "OK message", "continue or stop message", "OK message + warnings", "continue/stop + warnings"] ("type of dialog (OK msg:1)")
        n82 = local read "EVENT ms"() -> (w133:i32)
        n83 = Get Date/Time In Seconds() -> (seconds since 1Jan1904=w132:timestamp)
        n84 = event shown="[44] \"Simulators\": Value Change" {
          selector: _ -> [_ _ _ _ _ _ _ _ _ _ _ _ _ _ _ _ _ _ _ _ _ _ _ _ _ _ _ _ _ _ _ _ _ _ _ _ _ _ _ _ _ _ _ _ _ _ _ _ _ _ _ _ _ _ _ _ _ _ _ _]
          dyn-events: _ -> [_ _ _ _ _ _ _ _ _ _ _ _ _ _ _ _ _ _ _ _ _ _ _ _ _ _ _ _ _ _ _ _ _ _ _ _ _ _ _ _ _ _ _ _ _ _ _ _ _ _ _ _ _ _ _ _ _ _ _ _]
          timeout: w133 -> [_ _ _ _ _ _ _ _ _ _ _ _ _ _ _ _ _ _ _ _ _ _ _ _ _ _ _ _ _ _ _ _ _ _ _ _ _ _ _ _ _ _ _ _ _ _ _ _ _ _ _ _ _ _ _ _ _ _ _ _]
          tunnel: w139 -> [_ _ _ _ _ _ _ _ _ _ _ _ _ _ w294 _ _ w317 _ _ _ _ _ _ _ _ _ w544 _ _ _ _ _ _ _ _ _ _ _ _ _ _ _ _ _ _ _ _ _ _ _ w1187 _ _ _ _ _ _ _ _]
          tunnel: [_ _ w155 _ w181 w185 w214 _ _ _ _ _ w271 w281 w286 _ w302 w316 w336 _ _ _ _ _ _ _ w439 _ w548 _ w575 _ _ _ w585 w678 w723 w741 w749 _ _ w951 _ _ w962 _ w1007 w1057 _ _ w1164 w1186 w1336 w1421 w1428 w1431 w1434 w1437 w1440 w1443] -> w138
          tunnel: [_ _ _ _ _ _ _ _ _ _ _ _ _ _ _ _ _ _ _ _ _ _ _ _ _ _ _ w547 _ _ _ _ _ _ _ _ _ _ _ _ _ _ _ _ _ _ _ _ _ _ _ _ _ _ _ _ _ _ _ _] -> w137
          tunnel: [_ _ _ _ _ _ _ _ _ _ _ _ _ _ _ _ w305 _ _ _ _ _ _ _ _ _ _ _ _ _ _ _ _ _ _ _ _ _ _ _ _ _ _ _ _ _ _ _ _ _ _ _ _ _ _ _ _ _ _ _] -> w134
          tunnel: w132 -> [_ _ _ _ _ _ _ _ _ _ _ _ _ _ _ _ _ _ _ _ _ _ _ _ _ _ _ _ _ _ _ _ _ _ _ _ w721 _ _ _ _ _ _ _ _ _ _ _ _ _ _ _ w1335 _ _ _ _ _ _ _]
          event "Admin Panel": Value Change {
            n85 = event-data() -> ("NewVal"=w148:bool)  [unwired: 1 in]
            n86 = Select(t=310 ("Splitter Position"), s=w148, f=52 ("Splitter Position")) -> (s? t:f=w149:i32)
            n87 = property on="Splitter" class="Splitter"("Position"=w149) -> ()  [unwired: 2 in, 2 out]
            n88 = Select(t=T66."Always On" ("Vertical Scrollbar Visibility"), s="Admin Panel", f=T66."Always Off" ("Vertical Scrollbar Visibility")) -> (s? t:f=w143:T66)
            n89 = property on="VISA Report En" class="Bool (strict)"("Value"="Admin Panel") -> ()  [unwired: 2 in, 2 out]
            n90 = property on="Pane 2" class="Pane"("VertScrollbarVisibility"=w143) -> ()  [unwired: 2 in, 2 out]
            n91 = property on="Pane 2" class="Pane"("Origin"=T67 {"Horizontal"=0, "Vertical"=0}) -> ()  [unwired: 2 in, 2 out]
          }
          event "Button": Value Change {
            n92 = event-data() -> ()  [unwired: 1 in, 1 out]
            n93 = local write "Tab Control 3"(T28."UV" ("Tab Control 3")) -> ()
            n94 = local write "Tab Auxi"(enum32{"Nursery", "Windows", "Auxiliary"}."Nursery" ("Tab Auxi")) -> ()
            n95 = local write "Tab NTR"(T68."Nursery Status" ("Tab NTR")) -> ()
          }
          event "Clear Virtuals": Value Change {
            n96 = event-data() -> ()  [unwired: 1 in, 1 out]
            n97 = disable-structure shown="Enabled" {
              disable-tunnel: [w156 _] -> w155
              frame Enabled {
                n98 = call "variantCtrlIo.vi"("menu (Get Param)"=enumVarCtrlIO."IO List Configs") -> ("IO Configs List"=w158:T42[])  [unwired: 6 in, 4 out]
                n99 = call "util-io-filter.vi"("IO Search Conf"=T70 {"Device"=-1, "Label"="", "Type"=enum."VL", "Mode"=enum."Mode", "Tags"=""} ("IO Search Conf 2"), "IO Configs List"=w158) -> ("Search Results"=w157:T42[])  [unwired: 9 in]
                n100 = for {
                  tunnel: w157 -> [w164] mode=indexing
                  tunnel: [w161] -> w156
                  n101 = Bundle By Name(cluster=w164, "Value"="") -> (w163:T42)
                  n102 = call "variantCtrlIo.vi"("menu (Get Param)"=enumVarCtrlIO."IO Modify Value By Key", "IOnode in"=w163) -> ("error out"=w161:errorcluster)  [unwired: 5 in, 4 out]
                }
              }
              frame Disabled {
              }
            }
          }
          event "Cluster.MAIN", "Cluster.I/O", "Cluster.ADMIN": Value Change {
            n103 = event-data() -> ("CtlRef"=w168:refnum<vi>)  [unwired: 1 in]
            n104 = property class="Bool (strict)"(reference=w168) -> ("Label.Text"=w166:string)  [unwired: 1 in, 2 out]
            n105 = property on="Tab Main" class="TabCtl (strict)"() -> ("Pages"=w170:refnum<vi>[])  [unwired: 2 in, 2 out]
            n106 = property on="Cluster" class="Clust (strict)"() -> ("Controls[]"=w167:refnum<vi>[])  [unwired: 2 in, 2 out]
            n107 = for {
              tunnel: w170 -> [w180] mode=indexing
              tunnel: w166 -> [w178]
              tunnel: [w177] -> w169 if=w176
              i -> [w177]
              n108 = property class="Page"(reference=w180) -> ("PageLabel"=w179:string)  [unwired: 1 in, 2 out]
              n109 = Equal?(x=w179, y=w178) -> (x = y?=w176:bool)
            }
            n110 = for {
              tunnel: w167 -> [w175] mode=indexing
              tunnel: w166 -> [w173]
              n111 = property class="Ctl"(reference=w175) -> (reference out=w172:refnum<vi>, "Label.Text"=w174:string)  [unwired: 1 in, 1 out]
              n112 = Equal?(x=w174, y=w173) -> (x = y?=w171:bool)
              n113 = property class="Ctl"(reference=w172, "Value"=w171) -> ()  [unwired: 1 in, 2 out]
            }
            n114 = local write "Tab Main"(w169) -> ()
          }
          event "COM": Value Change {
            n115 = event-data() -> ()  [unwired: 1 in, 1 out]
            n116 = global read "globals-engine.vi" "Q-Com"() -> (w183:refnum<queue>)
            n117 = Enqueue Element At Opposite End(queue=w183, element=cluster{"data":variant, "Enum":T55} {"data"=variant, "Enum"=enum."REC.FETCH"}) -> (error out=w181:errorcluster)  [unwired: 2 in, 2 out]
          }
          event "DO Set by Addr.Send": Value Change {
            (unwired) TRUE ("Timer Enable")
            n118 = event-data() -> ()  [unwired: 1 in, 6 out]
            n119 = property on="Send" class="Bool (strict)"("Value"=FALSE ("State")) -> ()  [unwired: 2 in, 2 out]
            n120 = Unbundle By Name("DO Set by Addr") -> ("State"=w193:bool, "ADDR"=w188:T8, "Timeout [s]"=w192:u8)
            n121 = Bundle By Name(cluster=cluster{"State":bool, "ADDR":T8, "Timeout":u8} {"State"=FALSE, "ADDR"=8, "Timeout"=8} ("digitalPort"), "State"=w193, "ADDR"=w188, "Timeout"=w192) -> (w191:cluster{"State":bool, "ADDR":T8, "Timeout":u8})
            n122 = global read "globals-engine.vi" "Q-Eng"() -> (w184:refnum<queue>)
            n123 = Bundle By Name(cluster=cluster{"case":T5, "data":variant} {"case"=enum."ENG.RIO.DOUT-BY-ADDR", "data"=variant} ("element"), "data"=w191) -> (w195:cluster{"case":T5, "data":variant})
            n124 = Enqueue Element At Opposite End(queue=w184, element=w195) -> (queue out=w187:refnum<queue>, error out=w186:errorcluster)  [unwired: 2 in, 1 out]
            n125 = disable-structure shown="Enabled" {
              disable-tunnel: w188 -> [w202 w205 _]
              disable-tunnel: w187 -> [w199 _ _]
              disable-tunnel: w186 -> [w198 w208 w209]
              disable-tunnel: [w197 w208 w209] -> w185
              frame Disabled {
                n126 = call "util-address-parser.vi"("ADDR 2"=w202) -> ("Address"=w201:u8)  [unwired: 9 in, 1 out]
                n127 = Build Array(w201) -> (w200:u8[])
                n128 = Bundle By Name(cluster=cluster{"case":T5, "data":variant} {"case"=enum."ENG.RIO.SNAPSHOT", "data"=variant} ("element"), "data"=w200) -> (w204:cluster{"case":T5, "data":variant})
                n129 = Enqueue Element(queue=w199, element=w204, error in (no error)=w198) -> (error out=w197:errorcluster)  [unwired: 1 in, 2 out]
              }
              frame Disabled {
                n130 = call "util-address-parser.vi"("ADDR 2"=w205) -> ("Address"=w206:u8)  [unwired: 9 in, 1 out]
                n131 = Format Into String(format string="Event Set DO by address %02d", w206) -> ()  [unwired: 2 in, 2 out]
              }
              frame Enabled {
              }
            }
          }
          event "DO Set by Name.Send": Value Change {
            (unwired) TRUE ("Timer Enable")
            n132 = event-data() -> ()  [unwired: 1 in, 2 out]
            n133 = property on="Send" class="Bool (strict)"("Value"=FALSE ("State")) -> ()  [unwired: 2 in, 2 out]
            n134 = Unbundle By Name("DO Set by Name") -> ("State"=w221:bool, "Name"=w213:string, "Timeout [s]"=w220:u8)
            n135 = Bundle By Name(cluster=T71 {"State"=FALSE, "Timeout"=0, "Name"=""} ("Cluster"), "State"=w221, "Name"=w213, "Timeout"=w220) -> (w219:T71)
            n136 = call "variantCtrlIo.vi"("menu (Get Param)"=enumVarCtrlIO."IO Get By Key", "Key (use IOnode Label if empty )"=w213) -> ("IOnode out"=w212:T42)  [unwired: 5 in, 4 out]
            n137 = Unbundle By Name(w212) -> ("ADDR"=w210:T8)
            n138 = global read "globals-engine.vi" "Q-Eng"() -> (w217:refnum<queue>)
            n139 = Bundle By Name(cluster=cluster{"case":T5, "data":variant} {"case"=enum."ENG.RIO.DOUT-BY-NAME", "data"=variant} ("element"), "data"=w219) -> (w224:cluster{"case":T5, "data":variant})
            n140 = Enqueue Element At Opposite End(queue=w217, element=w224) -> (queue out=w216:refnum<queue>, error out=w215:errorcluster)  [unwired: 2 in, 1 out]
            n141 = disable-structure shown="Enabled" {
              disable-tunnel: w216 -> [w230 _]
              disable-tunnel: w215 -> [w229 w235]
              disable-tunnel: [w228 w235] -> w214
              disable-tunnel: _ -> [w227 _]
              disable-tunnel: w210 -> [w226 _]
              frame Disabled {
                n142 = call "util-address-parser.vi"("ADDR 2"=w226) -> ("Address"=w232:u8)  [unwired: 9 in, 1 out]
                n143 = Build Array(w232) -> (w231:u8[])
                n144 = Bundle By Name(cluster=cluster{"case":T5, "data":variant} {"case"=enum."ENG.RIO.SNAPSHOT", "data"=variant} ("element"), "data"=w231) -> (w234:cluster{"case":T5, "data":variant})
                n145 = Enqueue Element(queue=w230, element=w234, error in (no error)=w229) -> (error out=w228:errorcluster)  [unwired: 1 in, 2 out]
              }
              frame Enabled {
              }
            }
          }
          event "ENG ms ctrl": Value Change {
            n146 = event-data() -> ()  [unwired: 1 in, 1 out]
          }
          event Value Change {
            n147 = event-data() -> ("NewVal"=w236:T1)  [unwired: 1 in]
            n148 = call "util.environment.vi"("Operation (Get)"=enum16{"get", "set"}."set" ("Operation"), "ENV in"=w236) -> ("error out"=w240:errorcluster)  [unwired: 8 in, 1 out]
            n149 = disable-structure shown="Disabled" {
              disable-tunnel: w236 -> [w255 _]
              frame Disabled {
                # "display tab pages if debugging"
                n150 = Not Equal?(x=typeEnv."ENV.PRODUCTION", y=w255) -> (x != y?=w253:bool)
                n151 = property on="Tab Main" class="TabCtl (strict)"("Tabs Visible?"=w253) -> ()  [unwired: 2 in, 2 out]
              }
              frame Enabled {
              }
            }
            n152 = Format Into String(w236) -> (resulting string=w241:string)  [unwired: 3 in, 1 out]
            n153 = call "util-ini-key.vi"("key"=ini-key."INI.ENV" ("input 1")) -> ("key"=w237:string, "section"=w238:string)  [unwired: 9 in]
            n154 = call "util-path.vi"("Create Folders?(F)"=FALSE, "error in"=w240, "Selected Folder (PROCS)"=typePathSelector."DIR_INI" ("Selected Folder (PROCEDURE_DIR)")) -> ("error out"=w250:errorcluster, "SelectedPath"=w248:path)  [unwired: 4 in, 3 out]
            n155 = call <vilib>:"Open Config Data.vi"("error in (no error)"=w250, "configuration file path"=w248) -> ("error out"=w249:errorcluster, "refnum"=w247:T64)  [unwired: 7 in, 1 out]
            n156 = call-poly <vilib>:"Write Key.vi"("write raw string? (F)"=TRUE, "section"=w238, "error in (no error)"=w249, "value"=w241, "key"=w237, "refnum"=w247) -> ("error out"=w246:errorcluster, "refnum out"=w245:T64)  [unwired: 3 in, 1 out]
            n157 = call <vilib>:"Close Config Data.vi"("error in (no error)"=w246, "refnum"=w245) -> ("error out"=→"error out":errorcluster)  [unwired: 8 in, 1 out]
          }
          event "EVENT ms": Value Change {
            n158 = event-data() -> ()  [unwired: 1 in, 1 out]
          }
          event "File path": Value Change {
            n159 = event-data() -> ("NewVal"=w256:path)  [unwired: 1 in]
            n160 = call "util.file.vars.file-operations.vi"("selected path"=w256) -> ("error out"=w260:errorcluster, "Procedure"=w259:variant[])  [unwired: 8 in, 1 out]
            n161 = call "build.proc.parse.vi"("error"=w260, "Array in"=w259) -> ("Flow Steps"=w257:T49[], "Proc Head"=w258:T48)  [unwired: 7 in, 1 out]
            n162 = local write "UiBuildSteps"(w257) -> ()
            n163 = local write "UiBuildProcHead"(w258) -> ()
          }
          event "filter": Value Change {
            n164 = event-data() -> ()  [unwired: 1 in, 1 out]
            n165 = local read "Serial Record(s)"() -> (w264:T53[])
            n166 = call "helper-serial-log-to-string-2.vi"("filter"="filter", "Array in"=w264) -> ("Array out"=w261:T51[])  [unwired: 9 in]
            "COM Snapshot" <- w261
            n167 = Array Size(array=w261) -> (size(s)=→"Serial Log Size":i32)
            n168 = local write "COM Snapshot"(w261) -> ()
          }
          event "IO Add New": Value Change {
            n169 = event-data() -> ()  [unwired: 1 in, 1 out]
            n170 = Bundle By Name(cluster="New Element", "Mode"=enum.io.mode."RIO") -> (w267:T42)
            n171 = call "variantCtrlIo.vi"("menu (Get Param)"=enumVarCtrlIO."IO Add By Key", "IOnode in"=w267) -> ("error out"=w266:errorcluster)  [unwired: 5 in, 4 out]
            n172 = local write "New Element"(T42 {"ADDR"=0, "Label"="", "Type"=enum."Type", "Mode"=enum."RIO", "Value"="", "Tags"="", "calibration"=[]} ("New Element")) -> ()
            n173 = global read "globals-engine.vi" "Q-Log"() -> (w272:refnum<queue>)
            n174 = Enqueue Element(queue=w272, element=cluster{"data":variant, "Enum":T57} {"data"=variant, "Enum"=enum."LOG.UPDATE.SELECTORS"}, error in (no error)=w266) -> (error out=w271:errorcluster)  [unwired: 1 in, 2 out]
          }
          event "IO calib save": Value Change {
            n175 = event-data() -> ()  [unwired: 1 in, 1 out]
            n176 = local read "IO calib select"() -> (w283:string)
            n177 = call "variantCtrlIo.vi"("menu (Get Param)"=enumVarCtrlIO."IO Get By Key", "Key (use IOnode Label if empty )"=w283) -> ("error out"=w275:errorcluster, "IOnode out"=w282:T42)  [unwired: 5 in, 3 out]
            n178 = local write "IO calib save"(FALSE ("calib save")) -> ()
            n179 = in-place {
              n180 = in-place-cluster #1(w282) -> ()  [unwired: 1 out]
              n181 = in-place-cluster #1("calibration"="XyPairs") -> (w278:T42)
            }
            n182 = global read "globals-engine.vi" "Q-Eng"() -> (w274:refnum<queue>)
            n183 = call "variantCtrlIo.vi"("menu (Get Param)"=enumVarCtrlIO."IO Modify Calib By Key", "error in"=w275, "IOnode in"=w278) -> ("error out"=w276:errorcluster)  [unwired: 4 in, 4 out]
            n184 = Enqueue Element(queue=w274, element=cluster{"cmd":T5, "data":variant} {"cmd"=enum."ENG.IO.SAVE", "data"=variant} ("typedefElement"), error in (no error)=w276) -> (error out=w281:errorcluster)  [unwired: 1 in, 2 out]
          }
          event "IO calib select": Value Change {
            n185 = event-data() -> ("NewVal"=w290:string)  [unwired: 1 in]
            n186 = call "variantCtrlIo.vi"("menu (Get Param)"=enumVarCtrlIO."IO Get By Key", "Key (use IOnode Label if empty )"=w290) -> ("error out"=w287:errorcluster, "IOnode out"=w289:T42)  [unwired: 5 in, 3 out]
            n187 = property on="Chart" class="WFChart (strict)"("History Data"=cluster{"X":dbl, "Y":dbl}[] []) -> ()  [unwired: 2 in, 2 out]
            n188 = Unbundle By Name(w289) -> ("calibration"=w288:T43[])
            n189 = local write "XyPairs"(w288) -> ()
            n190 = Enqueue Element(queue=w294, element=cluster{"cmd":T5, "data":variant} {"cmd"=enum."ENG.RIO.AIN-SNAPSHOT-CALIB", "data"=variant} ("typedefElement"), error in (no error)=w287) -> (error out=w293:errorcluster)  [unwired: 1 in, 2 out]
            n191 = call <vilib>:"Clear Errors.vi"("error in (no error)"=w293) -> ("error out"=w286:errorcluster)  [unwired: 5 in, 1 out]
          }
          event "IO Conf view": Value Change {
            n192 = event-data() -> ("NewVal"=w298:enum16{"Show All", "Search"})  [unwired: 1 in]
            n193 = case shown="\"Show All\"" w298 {
              tunnel: [T72."Disabled and Grayed Out" ("Disabled") T72."Enabled" ("Disabled")] -> w297
              frame "Show All" {
              }
              frame "Search" {
              }
            }
            n194 = property on="IO Search Conf" class="Clust (strict)"("DisabledEnum"=w297, "Value"=T45 {"ADDR"=-1, "Label"="", "Type"=enum."Type", "Mode"=enum."Mode", "Tags"=""} ("IO Search Conf")) -> ()  [unwired: 2 in, 2 out]
          }
          event "IO Conf": Value Change {
            # "IO Conf not allows adding (or removing) elements using right-click menu. new elements added by seperate ui object and the IO conf only allow to edit elements and delete by renaming to empty name"
            n195 = event-data() -> ("OldVal"=w309:T46, "NewVal"=w308:T46)  [unwired: 1 in]
            n196 = call "helper-io-edit.vi"("NewVal"=w308, "OldVal"=w309) -> ("error out"=w303:errorcluster, "IO changed?"=w304:bool)  [unwired: 7 in, 1 out]
            n197 = Select(t="Edit I/O Configuration" ("string"), s=w304, f="") -> (s? t:f=w305:string)
            n198 = case shown="True" w304 {
              tunnel: w303 -> [w310 w312]
              tunnel: [w310 w311] -> w302
              frame False {
              }
              frame True {
                n199 = global read "globals-engine.vi" "Q-Eng"() -> (w314:refnum<queue>)
                n200 = Enqueue Element(queue=w314, element=cluster{"cmd":T5, "data":variant} {"cmd"=enum."ENG.STATUS", "data"=variant} ("typedefElement"), error in (no error)=w312) -> (error out=w311:errorcluster)  [unwired: 1 in, 2 out]
              }
            }
            n201 = local read "IO Search Conf"() -> (w301:T45)
            n202 = property on="IO Search Conf" class="Clust (strict)"("Val(Sgnl)"=w301) -> ()  [unwired: 2 in, 2 out]
          }
          event "IO List.save", "IO List.loadCsv": Value Change {
            n203 = event-data() -> ("CtlRef"=w319:refnum<vi>)  [unwired: 1 in]
            n204 = property class="Bool (strict)"(reference=w319) -> ("Label.Text"=w318:string)  [unwired: 1 in, 2 out]
            n205 = local write "IO List"(cluster{"save":bool, "loadCsv":bool} {"save"=FALSE, "loadCsv"=FALSE} ("StorageMenu")) -> ()
            n206 = case shown="\"save\"" w318 {
              tunnel: [w321 w327 errorcluster {"status"=TRUE, "code"=-564498, "source"="Case Error for UiMenuIoBuilder"} ("error out")] -> w316
              tunnel: w317 -> [w322 w324 _]
              frame "save" {
                # "save to IO directory"
                n207 = Enqueue Element At Opposite End(queue=w322, element=cluster{"cmd":T5, "data":variant} {"cmd"=enum."ENG.IO.SAVE", "data"=variant} ("typedefElement")) -> (error out=w321:errorcluster)  [unwired: 2 in, 2 out]
              }
              frame "loadCsv" {
                n208 = call "util-io-csv-load.vi"("file path (dialog if empty)"=path "") -> ("error out"=w325:errorcluster, "Array"=w326:T42[])  [unwired: 9 in]
                n209 = case shown="No Error" w325 {
                  selector: w325 -> [_ w334]
                  tunnel: [w333 w334] -> w327
                  tunnel: w326 -> [w328 _]
                  tunnel: w324 -> [w332 _]
                  frame No Error {
                    n210 = Bundle By Name(cluster=cluster{"cmd":T5, "data":variant} {"cmd"=enum."ENG.IO.LOAD", "data"=variant} ("typedefElement"), "data"=w328, "cmd"=state-engine."ENG.IO.LOAD") -> (w330:cluster{"cmd":T5, "data":variant})
                    n211 = Enqueue Element(queue=w332, element=w330) -> (error out=w333:errorcluster)  [unwired: 2 in, 2 out]
                  }
                  frame Error {
                  }
                }
              }
              frame Default {
              }
            }
          }
          event "IO Map DO": Value Change {
            n212 = event-data() -> ("OldVal"=w338:T37[], "NewVal"=w344:T37[])  [unwired: 1 in]
            n213 = Not Equal?(x=w338, y=w344) -> (x != y?=w346:T76)
            n214 = Array Max & Min(array=w346) -> (max index (indices)=w339:i32)  [unwired: 3 out]
            n215 = Index Array(array=w346, index=w339) -> (element=w345:T77)
            n216 = Index Array(array=w344, index=w339) -> (element=w343:T37)
            n217 = Unbundle By Name(w343) -> ("ADDR"=w337:T8, "Label"=w342:string, "State"=w341:bool)
            n218 = Unbundle By Name(w345) -> ("State"=w340:bool)
            n219 = case shown="True" w340 {
              tunnel: w342 -> [_ w348]
              tunnel: w341 -> [_ w352]
              tunnel: w337 -> [_ w351]
              tunnel: [_ w347] -> w336
              frame False {
              }
              frame True {
                n220 = property on="Timeout [s]" class="DigNum (strict)"() -> ("Value"=w349:u8)  [unwired: 2 in, 2 out]
                n221 = call "helper-do-active-verif.vi"("name"=w348, "Value"=w349, "State"=w352, "ADDR"=w351) -> ("digitalPort"=w353:cluster{"State":bool, "ADDR":T8, "Timeout":u8}, "T button?"=w350:bool)  [unwired: 6 in]
                n222 = case shown="True" w350 {
                  tunnel: w353 -> [w357 _]
                  tunnel: [w354 _] -> w347
                  frame True {
                    w356 = cluster{"cmd":T5, "data":variant} {"cmd"=enum."ENG.RIO.SNAPSHOT", "data"=variant}  # snapshot all
                    n223 = global read "globals-engine.vi" "Q-Eng"() -> (w359:refnum<queue>)
                    n224 = Bundle By Name(cluster=cluster{"case":T5, "data":variant} {"case"=enum."ENG.RIO.DOUT-BY-ADDR", "data"=variant} ("element"), "data"=w357) -> (w360:cluster{"case":T5, "data":variant})
                    n225 = Enqueue Element At Opposite End(queue=w359, element=w360) -> (queue out=w355:refnum<queue>)  [unwired: 2 in, 2 out]
                    n226 = Enqueue Element(queue=w355, element=w356) -> (error out=w354:errorcluster)  [unwired: 2 in, 2 out]
                  }
                  frame False {
                    w362 = cluster{"cmd":T5, "data":variant} {"cmd"=enum."ENG.RIO.SNAPSHOT", "data"=variant}  # snapshot all
                    n227 = global read "globals-engine.vi" "Q-Eng"() -> (w361:refnum<queue>)
                    n228 = Enqueue Element(queue=w361, element=w362) -> ()  [unwired: 2 in, 3 out]
                  }
                }
              }
            }
          }
          event "IO Map Take Snapshot": Value Change {
            w363 = cluster{"cmd":T5, "data":variant} {"cmd"=enum."ENG.RIO.SNAPSHOT", "data"=variant}  # snapshot all
            n229 = event-data() -> ()  [unwired: 1 in, 1 out]
            n230 = local write "IO Map Take Snapshot"(FALSE ("IO Map Take Snapshot")) -> ()
            n231 = global read "globals-engine.vi" "Q-Eng"() -> (w365:refnum<queue>)
            n232 = property on="State" class="Bool (strict)"("DisabledEnum"=T72."Disabled" ("Disabled")) -> ()  [unwired: 2 in, 2 out]
            n233 = Enqueue Element(queue=w365, element=w363) -> ()  [unwired: 2 in, 3 out]
          }
          event "IO Search Conf": Value Change {
            n234 = event-data() -> ()  [unwired: 1 in, 6 out]
            n235 = call "variantCtrlIo.vi"("menu (Get Param)"=enumVarCtrlIO."IO List Configs") -> ("IO Configs List"=w373:T42[])  [unwired: 6 in, 4 out]
            n236 = call "util-io-filter.vi"("IO Search Conf"="IO Search Conf", "IO Configs List"=w373) -> ("Search Results"=w370:T42[])  [unwired: 9 in]
            n237 = local read "IOconf Sort"() -> (w368:T44)
            n238 = call "util-io-sort.vi"(10:w368, "IO Configs List"=w370) -> ("Result"=w369:T42[])  [unwired: 9 in]
            n239 = Array Size(array=w369) -> (size(s)=→"size":i32)
            n240 = local write "IO Conf"(w369) -> ()
          }
          event "IO Search Map Refresh": Value Change {
            n241 = event-data() -> ()  [unwired: 1 in, 1 out]
            n242 = local write "IO Search Map Refresh"(FALSE ("IO Search Refresh")) -> ()
            n243 = property on="IO Search Map" class="Clust (strict)"("Val(Sgnl)"=T41 {"By Name"="", "By Tag"="", "By Address"=-1} ("Value (Signaling)")) -> ()  [unwired: 2 in, 2 out]
          }
          event "IO Search Map": Value Change {
            n244 = event-data() -> ()  [unwired: 1 in, 1 out]
            n245 = Unbundle By Name("IO Search Map") -> ("By Address"=w383:i32, "By Name"=w393:string, "By Tag"=w392:string)
            n246 = call "variantCtrlIo.vi"("menu (Get Param)"=enumVarCtrlIO."IO List Configs") -> ("IO Configs List"=w385:T42[])  [unwired: 6 in, 4 out]
            n247 = call "util-address-range.vi"("ADDR"=w383) -> ("x .and. y?"=w378:bool)  [unwired: 10 in]
            n248 = Select(t=T72."Enabled" ("Disabled"), s=w378, f=T72."Disabled and Grayed Out" ("Disabled")) -> (s? t:f=w379:T72)
            n249 = case shown="False" w378 {
              selector: w378 -> [w416 _]
              tunnel: [w416 w417] -> w377
              frame False {
              }
              frame True {
                n250 = local read "Show Undefined"() -> (w417:bool)
              }
            }
            n251 = And(x=w378, y=w377) -> (x .and. y?=w382:bool)
            n252 = case shown="False" w382 {
              tunnel: w385 -> [w418 w421]
              tunnel: [w418 w420] -> w384
              tunnel: w383 -> [_ w419]
              frame False {
              }
              frame True {
                n253 = call "helper-snapshot-list.vi"("ADDR"=w419, "IOnodes in"=w421) -> ("IOcon snapshot list out"=w420:T42[])  [unwired: 9 in]
              }
            }
            n254 = property on="Show Undefined" class="Bool (strict)"("DisabledEnum"=w379) -> ()  [unwired: 2 in, 2 out]
            n255 = Bundle By Name(cluster=T73 {"ADDR"=0, "Label"="", "Type"=enum."Type", "Mode"=enum."Mode", "Tags"=""} ("IO Search Conf"), "ADDR"=w383, "Label"=w393, "Tags"=w392) -> (w391:T73)
            n256 = call "util-io-filter.vi"("IO Search Conf"=w391, "IO Configs List"=w384) -> ("Search Results"=w376:T42[])  [unwired: 9 in]
            n257 = call "helper-io-set-tables.vi"("IOnodes"=w376) -> ("VL"=w387:T42[], "IO Map AI"=w388:T39[], "IO Map DO"=w389:T37[], "IO Map DI"=w390:T40[])  [unwired: 7 in]
            n258 = disable-structure shown="Enabled" {
              disable-tunnel: w390 -> [w411 w415]
              disable-tunnel: w389 -> [w410 w414]
              disable-tunnel: w388 -> [w409 w413]
              disable-tunnel: w387 -> [w408 w412]
              disable-tunnel: u32[] [0] ("Index Values") -> [w407 _]
              frame Disabled {
                n259 = property on="IO Map DI" class="Arr (strict)"("Value"=w411, "Index Values"=w407) -> ()  [unwired: 2 in, 2 out]
                n260 = property on="IO Map DO" class="Arr (strict)"("Value"=w410, "Index Values"=w407) -> ()  [unwired: 2 in, 2 out]
                n261 = property on="IO Map AI" class="Arr (strict)"("Value"=w409, "Index Values"=w407) -> ()  [unwired: 2 in, 2 out]
                n262 = property on="IO Map VL" class="Arr (strict)"("Value"=w408, "Index Values"=w407) -> ()  [unwired: 2 in, 2 out]
              }
              frame Enabled {
                n263 = property on="IO Map DI" class="Arr (strict)"("Value"=w415) -> ()  [unwired: 2 in, 2 out]
                n264 = property on="IO Map DO" class="Arr (strict)"("Value"=w414) -> ()  [unwired: 2 in, 2 out]
                n265 = property on="IO Map AI" class="Arr (strict)"("Value"=w413) -> ()  [unwired: 2 in, 2 out]
                n266 = property on="IO Map VL" class="Arr (strict)"("Value"=w412) -> ()  [unwired: 2 in, 2 out]
              }
            }
            n267 = flat-sequence {
              tunnel: w390 -> [w406]
              tunnel: w389 -> [w404]
              tunnel: w388 -> [w400]
              tunnel: w387 -> [w399]
              frame #0 {
                w397 = cluster{"cmd":T5, "data":variant} {"cmd"=enum."ENG.RIO.SNAPSHOT", "data"=variant}  # snapshot all
                n268 = Array Size(array=w404) -> (size(s)=→"IO Map DO Count":i32)
                n269 = Array Size(array=w399) -> (size(s)=→"IO Map VL Count":i32)
                n270 = Array Size(array=w400) -> (size(s)=→"IO Map AI Count":i32)
                n271 = Array Size(array=w406) -> (size(s)=→"IO Map DI Count":i32)
                n272 = global read "globals-engine.vi" "Q-Eng"() -> (w398:refnum<queue>)
                n273 = Enqueue Element(queue=w398, element=w397) -> ()  [unwired: 2 in, 3 out]
              }
            }
          }
          event Value Change {
            n274 = event-data() -> ()  [unwired: 1 in, 1 out]
            n275 = local read "IO Search Conf"() -> (w422:T45)
            n276 = property on="IO Search Conf" class="Clust (strict)"("Val(Sgnl)"=w422) -> ()  [unwired: 2 in, 2 out]
          }
          event Value Change {
            n277 = event-data() -> ()  [unwired: 1 in, 1 out]
            n278 = disable-structure shown="Enabled" {
              disable-tunnel: "IRR Params" -> [w424]
              frame Enabled {
                n279 = global write "globals-engine.vi" "IRR Params"(w424) -> ()
                n280 = To Variant(anything=w424) -> (Variant=w432:variant)
                n281 = Build Array(w432) -> (w431:variant[])
                n282 = call "util.file.vars.vi"("Operation(Read)"=enum16{"Read File", "Write File"}."Write File", "Directory (DIR_PROC)"=typePathSelector."DIR_CONFIG" ("Directory (PROCEDURE_DIR)"), "Proc Name(open dialog if empty)"="IRR_CONF" ("Proc Name"), "Vars[] in"=w431) -> ("error out"=w430:errorcluster)  [unwired: 3 in, 4 out]
                n283 = case shown="No Error" w430 {
                  selector: w430 -> [_ w434]
                  tunnel: [_ w434] -> w429
                  frame No Error {
                  }
                  frame Error {
                  }
                }
                n284 = global read "globals-engine.vi" "Q-Log"() -> (w433:refnum<queue>)
                n285 = Enqueue Element(queue=w433, element=cluster{"data":variant, "Enum":T57} {"data"=variant, "Enum"=enum."LOG.UPDATE.IRR"} ("procQ"), error in (no error)=w429) -> ()  [unwired: 1 in, 3 out]
              }
            }
          }
          event "Log Clear": Value Change {
            n286 = event-data() -> ()  [unwired: 1 in, 1 out]
            n287 = call "reg-log-general.vi"("Operation(Read)"=enum.report-filter."ClearAll") -> ("compact report"=w437:T78[])  [unwired: 8 in, 2 out]
            n288 = local write "Report General"(w437) -> ()
            n289 = local write "Proc Name"("" ("Proc Name")) -> ()
          }
          event "MenuRuntime.Run", "MenuRuntime.Step", "MenuRuntime.Load", "MenuRuntime.Status", "MenuRuntime.ProcedureRun", "MenuRuntime.ProcedureStep", "MenuRuntime.ProcedureReload", "MenuRuntime.Unload", "MenuRuntime.Reload": Value Change {
            n290 = event-data() -> ("CtlRef"=w444:refnum<vi>)  [unwired: 1 in]
            n291 = property class="Bool (strict)"(reference=w444) -> (reference out=w443:refnum<vi>, "Value"=w442:bool, "Label.Text"=w440:string)  [unwired: 1 in, 1 out]
            n292 = global read "globals-engine.vi" "Q-Eng"() -> (w438:refnum<queue>)
            n293 = case shown="\"Unload\"" w440 {
              tunnel: w438 -> [w447 w449 w452 w493 w504 w513 w518 _ w525 w528 w533 _]
              tunnel: w442 -> [_ _ _ _ _ w514 _ w523 _ w529 _ _]
              tunnel: [_ _ _ _ _ w514 _ w523 _ w529 _ FALSE] -> w441
              tunnel: [w446 w448 w451 w494 w505 w512 w517 w522 w524 w527 w532 errorcluster {"status"=TRUE, "code"=-1, "source"="Missing menu in UiRuntimeMenu"} ("error out")] -> w439
              frame "Init" {
                n294 = Enqueue Element(queue=w447, element=cluster{"cmd":T5, "data":variant} {"cmd"=enum."ENG.INIT", "data"=variant} ("typedefElement")) -> (error out=w446:errorcluster)  [unwired: 2 in, 2 out]
              }
              frame "InitGlobals" {
                n295 = Enqueue Element(queue=w449, element=cluster{"cmd":T5, "data":variant} {"cmd"=enum."ENG.INIT.VARS", "data"=variant} ("typedefElement")) -> (error out=w448:errorcluster)  [unwired: 2 in, 2 out]
              }
              frame "Load" {
                # "LOAD FOR PRODUCTION"
                n296 = call <vilib>:"Three Button Dialog.vi"("Right Button Text (\"Cancel\")"="All" ("Left Button Text (\"Yes\")"), "Center Button Text (\"No\")"="Folder" ("Left Button Text (\"Yes\")"), "Left Button Text (\"Yes\")"="File" ("Left Button Text (\"Yes\")"), "message"="Load ...") -> ("Which Button?"=w457:T79)  [unwired: 7 in]
                n297 = case shown="\"Left Button\"" w457 {
                  tunnel: w452 -> [_ w461 w474 w487]
                  tunnel: [_ w460 w473 w486] -> w451
                  frame "Window Close", Default {
                  }
                  frame "Left Button" {
                    w458 = 43  # canceled?
                    # "Load Single"
                    n298 = call "util.file.vars.path-parser.vi"("allowDialogs?(False)"=TRUE) -> ("error out"=w463:errorcluster, "cancelled"=w464:bool, "selected path"=w465:path)  [unwired: 8 in]
                    n299 = call <vilib>:"Clear Errors.vi"("error in (no error)"=w463, "specific error code to clear (0: all)"=w458) -> ("error out"=w459:errorcluster)  [unwired: 4 in, 1 out]
                    n300 = case shown="False" w464 {
                      tunnel: w465 -> [w471 _]
                      tunnel: w461 -> [w470 _]
                      tunnel: [w467 w472] -> w460
                      tunnel: w459 -> [w466 w472]
                      frame False {
                        n301 = Bundle By Name(cluster=cluster{"cmd":T5, "data":variant} {"cmd"=enum."ENG.LOAD.SINGLE", "data"=variant} ("typedefElement"), "data"=w471) -> (w469:cluster{"cmd":T5, "data":variant})
                        n302 = Enqueue Element(queue=w470, element=w469, error in (no error)=w466) -> (error out=w467:errorcluster)  [unwired: 1 in, 2 out]
                      }
                      frame True {
                      }
                    }
                  }
                  frame "Center Button" {
                    # "Load Module"
                    n303 = call "util.file.vars.path-parser.vi"("allowDialogs?(False)"=TRUE) -> ("error out"=w476:errorcluster, "cancelled"=w477:bool, "selected path"=w478:path)  [unwired: 8 in]
                    n304 = case shown="False" w477 {
                      tunnel: w478 -> [w484 _]
                      tunnel: w474 -> [w483 _]
                      tunnel: [w480 w485] -> w473
                      tunnel: w476 -> [w479 w485]
                      frame False {
                        n305 = Bundle By Name(cluster=cluster{"cmd":T5, "data":variant} {"cmd"=enum."ENG.LOAD.MODULE", "data"=variant} ("typedefElement"), "data"=w484) -> (w482:cluster{"cmd":T5, "data":variant})
                        n306 = Enqueue Element(queue=w483, element=w482, error in (no error)=w479) -> (error out=w480:errorcluster)  [unwired: 1 in, 2 out]
                      }
                      frame True {
                      }
                    }
                  }
                  frame "Right Button" {
                    # "Load All"
                    n307 = Enqueue Element(queue=w487, element=cluster{"cmd":T5, "data":variant} {"cmd"=enum."ENG.LOAD", "data"=variant} ("typedefElement")) -> (error out=w486:errorcluster)  [unwired: 2 in, 2 out]
                  }
                }
              }
              frame "ProcedureRun" {
                # "\"ProcedureRun\", \"Run\" \nset timeout interval to call eng execution periodically"
                n308 = property on="ProcedureSelect" class="CmbBox"() -> ("Value"=w491:string)  [unwired: 2 in, 2 out]
                n309 = Format Into String(format string="Run %s?", w491) -> (resulting string=w490:string)  [unwired: 2 in, 1 out]
                n310 = Two Button Dialog(message=w490) -> (T button?=w489:bool)  [unwired: 2 in]
                n311 = case shown="True" w489 {
                  tunnel: [_ w497] -> w494
                  tunnel: w493 -> [_ w496]
                  tunnel: w491 -> [_ w495]
                  frame False {
                  }
                  frame True {
                    n312 = Bundle By Name(cluster=cluster{"cmd":T5, "data":variant} {"cmd"=enum."ENG.PROC.START", "data"=variant} ("typedefElement"), "data"=w495) -> (w499:cluster{"cmd":T5, "data":variant})
                    n313 = Enqueue Element(queue=w496, element=w499) -> (error out=w497:errorcluster)  [unwired: 2 in, 2 out]
                  }
                }
              }
              frame "ProcedureLoad" {
                # "\"ProcedureRun\", \"Run\" \nset timeout interval to call eng execution periodically"
                n314 = property on="ProcedureSelect" class="CmbBox"() -> ("Value"=w502:string)  [unwired: 2 in, 2 out]
                n315 = Format Into String(format string="Reload %s?", w502) -> (resulting string=w501:string)  [unwired: 2 in, 1 out]
                n316 = Two Button Dialog(message=w501) -> (T button?=w500:bool)  [unwired: 2 in]
                n317 = case shown="True" w500 {
                  tunnel: [_ w508] -> w505
                  tunnel: w504 -> [_ w507]
                  tunnel: w502 -> [_ w506]
                  frame False {
                  }
                  frame True {
                    n318 = Bundle By Name(cluster=cluster{"cmd":T5, "data":variant} {"cmd"=enum."ENG.PROC.RELOAD-BY-NAME", "data"=variant} ("typedefElement"), "data"=w506) -> (w510:cluster{"cmd":T5, "data":variant})
                    n319 = Enqueue Element(queue=w507, element=w510) -> (error out=w508:errorcluster)  [unwired: 2 in, 2 out]
                  }
                }
              }
              frame "ProcedureStep" {
                n320 = property on="ProcedureSelect" class="CmbBox"() -> ("Value"=w511:string)  [unwired: 2 in, 2 out]
                n321 = call "eng-call-execute.vi"("Proc Name to Execute (empty: Execute All)"=w511, "Queue in"=w513) -> ("error out"=w512:errorcluster)  [unwired: 9 in]
              }
              frame "Reload" {
                n322 = Two Button Dialog(message="Reload All Procedures?") -> (T button?=w515:bool)  [unwired: 2 in]
                n323 = case shown="True" w515 {
                  tunnel: w518 -> [_ w521]
                  tunnel: [_ w520] -> w517
                  frame False {
                  }
                  frame True {
                    n324 = Enqueue Element(queue=w521, element=cluster{"cmd":T5, "data":variant} {"cmd"=enum."ENG.LOAD.RELOAD", "data"=variant} ("typedefElement")) -> (error out=w520:errorcluster)  [unwired: 2 in, 2 out]
                  }
                }
              }
              frame "Run" {
                # "\"ProcedureRun\", \"Run\" \nset timeout interval to call eng execution periodically"
                n325 = call "eng-call-start.vi"("Start(T)/Stop(F)"=w523) -> ("error out"=w522:errorcluster)  [unwired: 10 in]
              }
              frame "Status" {
                n326 = Enqueue Element(queue=w525, element=cluster{"cmd":T5, "data":variant} {"cmd"=enum."ENG.STATUS", "data"=variant} ("typedefElement")) -> (error out=w524:errorcluster)  [unwired: 2 in, 2 out]
              }
              frame "Step" {
                # "\"Step\" \ncall eng execution (once)"
                n327 = call "eng-call-execute.vi"("Queue in"=w528) -> ("error out"=w527:errorcluster)  [unwired: 10 in]
              }
              frame "Unload" {
                n328 = Two Button Dialog(message="Unload All Procedures?") -> (T button?=w530:bool)  [unwired: 2 in]
                n329 = case shown="True" w530 {
                  tunnel: w533 -> [_ w536]
                  tunnel: [_ w535] -> w532
                  frame False {
                  }
                  frame True {
                    n330 = for {
                      tunnel: w536 -> [w539]
                      tunnel: [w538] -> w535
                      tunnel: cluster{"cmd":T5, "data":variant}[] [{"cmd"=enum."ENG.LOAD.UNLOAD", "data"=variant}, {"cmd"=enum."ENG.STATUS", "data"=variant}] ("typedefElement") -> [w537] mode=indexing
                      n331 = Enqueue Element(queue=w539, element=w537) -> (error out=w538:errorcluster)  [unwired: 2 in, 2 out]
                    }
                  }
                }
              }
              frame Default {
              }
            }
            n332 = property class="Bool (strict)"(reference=w443, "Value"=w441) -> ()  [unwired: 1 in, 2 out]
          }
          event "MenuRuntime.Stop": Value Change {
            n333 = event-data() -> ("NewVal"=w547:bool)  [unwired: 1 in]
            n334 = Bundle By Name(cluster=cluster{"cmd":T5, "data":variant} {"cmd"=enum."ENG.EXIT", "data"=variant} ("typedefElement"), "data"=variant) -> (w545:cluster{"cmd":T5, "data":variant})
            n335 = global write "globals-engine.vi" "STOP"(TRUE ("STOP")) -> ()
            n336 = Enqueue Element At Opposite End(queue=w544, element=w545) -> ()  [unwired: 2 in, 3 out]
          }
          event "NTR Panel.CloseAll": Value Change {
            n337 = event-data() -> ("CtlRef"=w551:refnum<vi>)  [unwired: 1 in]
            n338 = property class="Bool (strict)"(reference=w551) -> ("Label.Text"=w550:string, "BoolText.Text"=w549:string)  [unwired: 1 in, 2 out]
            n339 = case shown="\"CloseAll\"" w550 {
              tunnel: w549 -> [_ w556]
              tunnel: [_ w552] -> w548
              frame "False", Default {
              }
              frame "CloseAll" {
                n340 = Concatenate Strings(w556, "?" ("string")) -> (w555:string)
                n341 = Two Button Dialog(message=w555) -> (T button?=w553:bool)  [unwired: 2 in]
                n342 = case shown="True" w553 {
                  tunnel: [_ w557] -> w552
                  frame False {
                  }
                  frame True {
                    n343 = global read "globals-engine.vi" "NutritionConfiguration"() -> (w558:T65[])
                    n344 = call "ntr-init-io.vi"("NutritionConfiguration"=w558) -> ("error out"=w557:errorcluster)  [unwired: 10 in]
                  }
                }
              }
            }
          }
          event "ntrGraphPeriod.lastDays": Value Change {
            n345 = event-data() -> ("NewVal"=w561:dbl)  [unwired: 1 in]
            n346 = Get Date/Time In Seconds() -> (seconds since 1Jan1904=w569:timestamp)
            n347 = invoke on="End" class="AbsTime (strict)" method="Reinit To Default"() -> (error out=w570:errorcluster)  [unwired: 3 in, 2 out]
            n348 = expression code="x*24*60*60"(w561) -> (w560:dbl)
            n349 = Subtract(x=w569, y=w560) -> (x-y=w562:timestamp)
            n350 = Seconds To Date/Time(time stamp (now)=w562) -> (date time rec=w566:T74)  [unwired: 1 in]
            n351 = Unbundle By Name(w566) -> ("year"=w565:i32, "month"=w564:i32, "day of month"=w563:i32)
            n352 = Bundle By Name(cluster=T74 {"fractional second"=0.0, "second"=0, "minute"=0, "hour"=0, "day of month"=0, "month"=0, "year"=0, "day of week"=0, "day of year"=0, "DST"=0} ("date time rec"), "year"=w565, "month"=w564, "day of month"=w563) -> (w567:T74)
            n353 = Date/Time To Seconds(2:w567) -> (0:w559:timestamp)  [unwired: 1 in]
            n354 = property on="Start" class="AbsTime (strict)"(error in=w570, "Val(Sgnl)"=w559) -> ()  [unwired: 1 in, 2 out]
          }
          event "ntrGraphPeriod.refresh": Value Change {
            n355 = event-data() -> ()  [unwired: 1 in, 3 out]
            n356 = property on="refresh" class="Bool (strict)"("Value"=FALSE) -> ()  [unwired: 2 in, 2 out]
            n357 = property on="ntrDosepumpSelect" class="CmbBox"() -> ("Value"=w573:string)  [unwired: 2 in, 2 out]
            n358 = property on="ntrInputSelect" class="CmbBox"() -> ("Value"=w571:string)  [unwired: 2 in, 2 out]
            n359 = call "util.ntr.dose-path.vi"("ntrGraphPeriod"="ntrGraphPeriod", "Dosepump"=w571) -> ("error out"=w575:errorcluster, "Graph"=→"Nutrition Sensor Graph":cluster{"X":dbl[], "Y":dbl[]})  [unwired: 7 in, 1 out]
            n360 = call "util.ntr.dose-path.vi"("ntrGraphPeriod"="ntrGraphPeriod", "Dosepump"=w573) -> ("Graph"=→"EC 3":cluster{"X":dbl[], "Y":dbl[]})  [unwired: 7 in, 2 out]
          }
          event "ntrInputSelect", "ntrGraphPeriod.Time range", "ntrDosepumpSelect": Value Change {
            n361 = event-data() -> ()  [unwired: 1 in, 1 out]
            n362 = property on="refresh" class="Bool (strict)"("Val(Sgnl)"=TRUE ("Value (Signaling)")) -> ()  [unwired: 2 in, 2 out]
          }
          event "pbr-proc-mode", "PBR Builder": Value Change {
            n363 = event-data() -> ()  [unwired: 1 in, 1 out]
            n364 = property on="COMPILE" class="Bool (strict)"("Val(Sgnl)"=TRUE ("Value (Signaling)")) -> ()  [unwired: 2 in, 2 out]
          }
          event "PBR PROC": Value Change {
            n365 = event-data() -> ()  [unwired: 1 in, 1 out]
            n366 = property on="LOAD" class="Bool (strict)"("Val(Sgnl)"=TRUE ("Value (Signaling)")) -> ()  [unwired: 2 in, 2 out]
          }
          event "PBR.COMPILE", "PBR.SAVE", "PBR.LOAD", "PBR.SAVEAS": Value Change {
            # "templateSave (save as text file)\ntemplateLoad (load from text file)\nprocedureSave(build flow and save as varient file)\nprocedureLoad(load from varient file and parse to flow)"
            n367 = event-data() -> ("CtlRef"=w586:refnum<vi>)  [unwired: 1 in]
            n368 = property class="Bool (strict)"(reference=w586, "Value"=FALSE) -> ("Label.Text"=w588:string)  [unwired: 1 in, 2 out]
            n369 = local read "PBR PROC"() -> (w581:string)
            n370 = feedback #2() -> (w582:variant[])  [unwired: 1 in]
            n371 = case shown="\"COMPILE\", Default" w588 {
              tunnel: [_ w611 w633 w652] -> w587
              tunnel: [w598 w605 w627 w647] -> w583
              tunnel: w582 -> [_ w605 w627 w646]
              tunnel: w581 -> [_ w609 _ w648]
              frame "COMPILE", Default {
                # "(2)"
                # "(1)"
                # "(1)  Build PBR_BUILDER to FLOW  \n(2)  Build FLOW to procedure (2.1) Save procedure (DIR_PROC)"
                n372 = local read "pbr-proc-mode"() -> (w589:enum16{"MANUAL", "AUTO"})
                n373 = local read "PBR Builder"() -> (w591:T23)
                n374 = case shown="\"MANUAL\", Default" w589 {
                  tunnel: [T48 {"Procedure Name"="", "Running"=FALSE, "tags"=""} ("Proc Head") T48 {"Procedure Name"="", "Running"=TRUE, "tags"=""} ("Proc Head")] -> w599
                  frame "MANUAL", Default {
                  }
                  frame "AUTO" {
                  }
                }
                n375 = call "pbr-builder.vi"("PBR FLOW in"=w591) -> ("Status"=w594:errorcluster, "FLOW out"=w590:T49[])  [unwired: 8 in, 1 out]
                n376 = call "build.proc.vi"("error in"=w594, "Flow"=w590, "Proc Head"=w599) -> ("error out"=w597:errorcluster, "Instructions"=w598:variant[])  [unwired: 7 in]
                n377 = Select(t=u32 16711680 ("Text.Text Colors:Text Color"), s=w597, f=u32 0 ("Text.Text Colors:Text Color")) -> (s? t:f=w600:u32)
                n378 = Select(t=w597, s=w597, f=errorcluster {"status"=FALSE, "code"=0, "source"="Compiled Successfully"} ("error constant")) -> (s? t:f=w595:errorcluster)
                n379 = property on="source" class="Str"("Text.TextColor"=w600) -> ()  [unwired: 2 in, 2 out]
                n380 = Unbundle By Name(w595) -> ("source"=w593:string)
                n381 = Concatenate Strings(w593) -> (→"source":string)
              }
              frame "SAVE" {
                # "(3)  Save PBR_BUILDER as CONFIG"
                n382 = Format Into String(format string="Save %s?", w609) -> (resulting string=w607:string)  [unwired: 2 in, 1 out]
                n383 = global read "globals-engine.vi" "Q-Eng"() -> (w606:refnum<queue>)
                n384 = Two Button Dialog(message=w607) -> (T button?=w610:bool)  [unwired: 2 in]
                n385 = case shown="True" w610 {
                  tunnel: [_ w617] -> w611
                  tunnel: w609 -> [_ w614]
                  tunnel: w605 -> [_ w621]
                  tunnel: w606 -> [_ w616]
                  frame False {
                  }
                  frame True {
                    n386 = call "util.file.vars.vi"("Operation(Read)"=enum16{"Read File", "Write File"}."Write File", "Proc Name(open dialog if empty)"=w614, "Vars[] in"=w621) -> ("error out"=w620:errorcluster)  [unwired: 4 in, 4 out]
                    n387 = Bundle By Name(cluster=cluster{"cmd":T5, "data":variant} {"cmd"=enum."ENG.PROC.STOP", "data"=variant} ("typedefElement"), "data"=w614) -> (w612:cluster{"cmd":T5, "data":variant})
                    n388 = Bundle By Name(cluster=cluster{"cmd":T5, "data":variant} {"cmd"=enum."ENG.PROC.RELOAD-BY-NAME", "data"=variant} ("typedefElement"), "data"=w614) -> (w619:cluster{"cmd":T5, "data":variant})
                    n389 = Build Array(w612, w619) -> (w613:cluster{"cmd":T5, "data":variant}[])
                    n390 = for {
                      tunnel: w616 -> [w624]
                      tunnel: w613 -> [w623] mode=indexing
                      shift-right: [w625] -> w617
                      shift-left: w620 -> [w626]
                      n391 = Enqueue Element(queue=w624, element=w623, error in (no error)=w626) -> (error out=w625:errorcluster)  [unwired: 1 in, 2 out]
                    }
                    n392 = invoke on="PBR_PLAY" class="Clust (strict)" method="Reinit To Default"() -> ()  [unwired: 3 in, 3 out]
                  }
                }
              }
              frame "SAVEAS" {
                n393 = call "ui-form-text-line.vi"("User Prompt in"="Insert Procedure Name (ie. HARVEST1)") -> ("Cancelled?"=w631:bool, "text out"=w630:string)  [unwired: 9 in]
                n394 = Concatenate Strings("PBR\\" ("string"), w630) -> (w628:string)
                n395 = case shown="False" w631 {
                  tunnel: [w634 _] -> w633
                  tunnel: w628 -> [w641 _]
                  tunnel: w627 -> [w644 _]
                  frame False {
                    n396 = call "util.file.vars.vi"("Operation(Read)"=enum16{"Read File", "Write File"}."Write File", "Proc Name(open dialog if empty)"=w641, "Vars[] in"=w644) -> ("error out"=w640:errorcluster, "File path"=w636:path)  [unwired: 4 in, 3 out]
                    n397 = call "pbr-get-procs-names.vi"("error in"=w640) -> ("error out"=w642:errorcluster, "Array"=w643:string[])  [unwired: 9 in]
                    n398 = global read "globals-engine.vi" "Q-Eng"() -> (w637:refnum<queue>)
                    n399 = property on="PBR PROC" class="CmbBox"(error in=w642, "Strings[]"=w643, "Value"=w641) -> (error out=w635:errorcluster)  [unwired: 1 in, 1 out]
                    n400 = Bundle By Name(cluster=cluster{"cmd":T5, "data":variant} {"cmd"=enum."ENG.LOAD.SINGLE", "data"=variant} ("typedefElement"), "data"=w636) -> (w639:cluster{"cmd":T5, "data":variant})
                    n401 = Enqueue Element(queue=w637, element=w639, error in (no error)=w635) -> (error out=w634:errorcluster)  [unwired: 1 in, 2 out]
                  }
                  frame True {
                  }
                }
              }
              frame "LOAD" {
                n402 = local read "PBR Builder"() -> (w650:T23)
                n403 = Empty Array?(array=w650) -> (empty?=w649:bool)
                n404 = case shown="False" w649 {
                  selector: w649 -> [_ w657]
                  tunnel: [w656 w657] -> w651
                  tunnel: w648 -> [w653 _]
                  frame False {
                    n405 = Format Into String(format string="Load %s?", w653) -> (resulting string=w654:string)  [unwired: 2 in, 1 out]
                    n406 = Two Button Dialog(message=w654) -> (T button?=w656:bool)  [unwired: 2 in]
                  }
                  frame True {
                  }
                }
                n407 = case shown="True" w651 {
                  tunnel: [_ w666] -> w652
                  tunnel: w648 -> [_ w665]
                  tunnel: [w658 w664] -> w647
                  tunnel: w646 -> [w658 _]
                  frame False {
                    # "Cancelled"
                  }
                  frame True {
                    # "Continue"
                    n408 = call "util.file.vars.vi"("Operation(Read)"=enum16{"Read File", "Write File"}."Read File", "Directory (DIR_PROC)"=typePathSelector."DIR_PROCS", "Proc Name(open dialog if empty)"=w665) -> ("error out"=w669:errorcluster, "Vars[] out"=w664:variant[])  [unwired: 4 in, 3 out]
                    n409 = call "build.proc.parse.vi"("error"=w669, "Array in"=w664) -> ("error out"=w667:errorcluster, "Flow Steps"=w671:T49[], "Proc Head"=w663:T48)  [unwired: 7 in]
                    n410 = Unbundle By Name(w663) -> ("Running"=w662:bool)
                    n411 = call "pbr-builder.vi"("FLOW in"=w671) -> ("PBR FLOW OUT"=w670:T23)  [unwired: 8 in, 2 out]
                    n412 = local write "PBR Builder"(w670) -> ()
                    n413 = Select(t=enum16{"MANUAL", "AUTO"}."AUTO" ("pbr-proc-mode"), s=w662, f=enum16{"MANUAL", "AUTO"}."MANUAL" ("pbr-proc-mode")) -> (s? t:f=w659:enum16{"MANUAL", "AUTO"})
                    n414 = local write "pbr-proc-mode"(w659) -> ()
                    n415 = invoke on="PBR_PLAY" class="Clust (strict)" method="Reinit To Default"() -> ()  [unwired: 3 in, 3 out]
                    n416 = property on="COMPILE" class="Bool (strict)"(error in=w667, "Val(Sgnl)"=TRUE ("Value (Signaling)")) -> (error out=w666:errorcluster)  [unwired: 1 in, 1 out]
                  }
                }
              }
            }
            n417 = feedback-in #2(w583) -> ()
            n418 = call <vilib>:"Clear Errors.vi"("error in (no error)"=w587) -> ("error out"=w585:errorcluster)  [unwired: 5 in, 1 out]
          }
          event "PBR_PLAY.PLAY", "PBR_PLAY.PAUSE", "PBR_PLAY.STOP": Value Change {
            n419 = event-data() -> ("CtlRef"=w680:refnum<vi>)  [unwired: 1 in]
            n420 = property class="Bool (strict)"(reference=w680) -> (reference out=w677:refnum<vi>, "Label.Text"=w679:string, "Value"=w675:bool)  [unwired: 1 in, 1 out]
            n421 = case shown="True" w675 {
              tunnel: w679 -> [_ w686]
              tunnel: [_ w685] -> w678
              tunnel: [TRUE ("T button?") w683] -> w676
              frame False {
              }
              frame True {
                n422 = global read "globals-engine.vi" "Q-Eng"() -> (w684:refnum<queue>)
                n423 = local read "PBR PROC"() -> (w682:string)
                n424 = case shown="\"STOP\"" w686 {
                  tunnel: [_ w692 w703 w714] -> w685
                  tunnel: w682 -> [_ w688 w699 w710]
                  tunnel: w684 -> [_ w691 w702 w713]
                  tunnel: [_ w690 w701 w712] -> w683
                  frame "False", Default {
                  }
                  frame "PLAY" {
                    n425 = Format Into String(format string="Start %s?", w688) -> (resulting string=w687:string)  [unwired: 2 in, 1 out]
                    n426 = Two Button Dialog(message=w687) -> (T button?=w690:bool)  [unwired: 2 in]
                    n427 = case shown="True" w690 {
                      tunnel: [_ w696] -> w692
                      tunnel: w688 -> [_ w693]
                      tunnel: w691 -> [_ w694]
                      frame False {
                      }
                      frame True {
                        n428 = Bundle By Name(cluster=cluster{"cmd":T5, "data":variant} {"cmd"=enum."ENG.PROC.START", "data"=variant} ("typedefElement"), "data"=w693) -> (w697:cluster{"cmd":T5, "data":variant})
                        n429 = Enqueue Element(queue=w694, element=w697) -> (error out=w696:errorcluster)  [unwired: 2 in, 2 out]
                      }
                    }
                  }
                  frame "PAUSE" {
                    n430 = Format Into String(format string="Pause %s?", w699) -> (resulting string=w698:string)  [unwired: 2 in, 1 out]
                    n431 = Two Button Dialog(message=w698) -> (T button?=w701:bool)  [unwired: 2 in]
                    n432 = case shown="True" w701 {
                      tunnel: [_ w707] -> w703
                      tunnel: w699 -> [_ w705]
                      tunnel: w702 -> [_ w704]
                      frame False {
                      }
                      frame True {
                        n433 = Bundle By Name(cluster=cluster{"cmd":T5, "data":variant} {"cmd"=enum."ENG.PROC.STOP", "data"=variant} ("typedefElement"), "data"=w705) -> (w708:cluster{"cmd":T5, "data":variant})
                        n434 = Enqueue Element(queue=w704, element=w708) -> (error out=w707:errorcluster)  [unwired: 2 in, 2 out]
                      }
                    }
                  }
                  frame "STOP" {
                    n435 = Format Into String(format string="Stop %s?", w710) -> (resulting string=w709:string)  [unwired: 2 in, 1 out]
                    n436 = Two Button Dialog(message=w709) -> (T button?=w712:bool)  [unwired: 2 in]
                    n437 = case shown="True" w712 {
                      tunnel: [_ w718] -> w714
                      tunnel: w710 -> [_ w716]
                      tunnel: w713 -> [_ w715]
                      frame False {
                      }
                      frame True {
                        n438 = Bundle By Name(cluster=cluster{"cmd":T5, "data":variant} {"cmd"=enum."ENG.PROC.RELOAD-BY-NAME", "data"=variant} ("typedefElement"), "data"=w716) -> (w719:cluster{"cmd":T5, "data":variant})
                        n439 = Enqueue Element(queue=w715, element=w719) -> (error out=w718:errorcluster)  [unwired: 2 in, 2 out]
                      }
                    }
                  }
                }
              }
            }
            n440 = case shown="True" w676 {
              selector: w676 -> [_ w720]
              tunnel: [_ w720] -> w674
              frame False {
              }
              frame True {
                n441 = invoke on="PBR_PLAY" class="Clust (strict)" method="Reinit To Default"() -> ()  [unwired: 3 in, 3 out]
              }
            }
            n442 = property class="Bool (strict)"(reference=w677, "Value"=w674) -> ()  [unwired: 1 in, 2 out]
          }
          event "PRBmenu.Harvest", "PRBmenu.SANI": Value Change {
            n443 = event-data() -> ("CtlRef"=w725:refnum<vi>)  [unwired: 1 in]
            n444 = property class="Bool (strict)"(reference=w725, "Value"=FALSE) -> ("Label.Text"=w724:string)  [unwired: 1 in, 2 out]
            n445 = case shown="\"False\", Default" w724 {
              tunnel: [_ w729 w735] -> w723
              tunnel: w721 -> [_ w726 _]
              frame "False", Default {
              }
              frame "Harvest" {
                n446 = local write "last"(w726) -> ()
                n447 = global read "globals-engine.vi" "Q-Eng"() -> (w732:refnum<queue>)
                n448 = Bundle By Name(cluster=cluster{"case":T5, "data":variant} {"case"=enum."ENG.PROC.START", "data"=variant} ("element"), "case"=state-engine."ENG.PROC.START", "data"="PBR\\HARVEST1") -> (w730:cluster{"case":T5, "data":variant})
                n449 = Enqueue Element(queue=w732, element=w730) -> (error out=w729:errorcluster)  [unwired: 2 in, 2 out]
              }
              frame "SANI" {
                n450 = global read "globals-engine.vi" "Q-Eng"() -> (w738:refnum<queue>)
                n451 = Bundle By Name(cluster=cluster{"case":T5, "data":variant} {"case"=enum."ENG.PROC.START", "data"=variant} ("element"), "case"=state-engine."ENG.PROC.START", "data"="PBR\\SANI") -> (w736:cluster{"case":T5, "data":variant})
                n452 = Enqueue Element(queue=w738, element=w736) -> (error out=w735:errorcluster)  [unwired: 2 in, 2 out]
              }
            }
          }
          event "Proc Select 2": Value Change {
            n453 = event-data() -> ()  [unwired: 1 in, 1 out]
            n454 = global read "globals-engine.vi" "Q-Eng"() -> (w740:refnum<queue>)
            n455 = Enqueue Element(queue=w740, element=cluster{"case":T5, "data":variant} {"case"=enum."ENG.PROC.STATUS", "data"=variant}) -> (error out=w741:errorcluster)  [unwired: 2 in, 2 out]
          }
          event "UiProjectSettings", "projectName": Value Change {
            n456 = event-data() -> ()  [unwired: 1 in, 6 out]
            n457 = local read "projectName"() -> (w742:string)
            n458 = Unbundle By Name("UiProjectSettings") -> ("Latitude"=w745:dbl, "Longitude"=w744:dbl, "TimeZone"=w743:i32)
            n459 = Bundle By Name(cluster="ProjectSettings", "Latitude"=w745, "Longitude"=w744, "TimeZone"=w743, "Project Name"=w742) -> (w746:T12)
            n460 = call "util-path.vi"("Create Folders?(F)"=FALSE, "Selected Folder (PROCS)"=typePathSelector."DIR_INI" ("Selected Folder (PROCEDURE_DIR)")) -> ("error out"=w762:errorcluster, "SelectedPath"=w763:path)  [unwired: 5 in, 3 out]
            n461 = Unbundle By Name(w746) -> ("Longitude"=w756:dbl, "Latitude"=w755:dbl, "TimeZone"=w754:i32, "Project Name"=w753:string)
            n462 = call <vilib>:"Open Config Data.vi"("error in (no error)"=w762, "configuration file path"=w763) -> ("error out"=w752:errorcluster, "refnum"=w759:T64)  [unwired: 7 in, 1 out]
            n463 = case shown="No Error" w752 {
              selector: w752 -> [_ w922]
              tunnel: w759 -> [w775 w921]
              tunnel: [_ w922] -> w758
              tunnel: [w774 w921] -> w757
              tunnel: w756 -> [w770 _]
              tunnel: w755 -> [w769 _]
              tunnel: w754 -> [w768 _]
              tunnel: w753 -> [w767 _]
              tunnel: [w765 _] -> w751
              frame No Error {
                n464 = stacked-sequence {
                  tunnel: [_ w815 _ _] -> w772
                  tunnel: w775 -> [w779 w814 w851 w887]
                  tunnel: [w778 _ _ _] -> w773
                  tunnel: [w777 _ _ _] -> w774
                  tunnel: [_ _ w850 _] -> w771
                  tunnel: w770 -> [w776 _ _ _]
                  tunnel: w769 -> [_ w813 _ _]
                  tunnel: w768 -> [_ _ w849 _]
                  tunnel: w767 -> [_ _ _ w886]
                  tunnel: [_ _ _ w885] -> w766
                  frame #0 {
                    w787 = 500  # timeout ms default
                    w802 = 500  # timeout ms default
                    n465 = call "util-path.vi"("Create Folders?(F)"=FALSE, "Selected Folder (PROCS)"=typePathSelector."DIR_INI" ("Selected Folder (PROCEDURE_DIR)")) -> ("error out"=w812:errorcluster, "SelectedPath"=w810:path)  [unwired: 5 in, 3 out]
                    n466 = call <vilib>:"Open Config Data.vi"("error in (no error)"=w812, "configuration file path"=w810) -> ("error out"=w811:errorcluster, "refnum"=w809:T64)  [unwired: 7 in, 1 out]
                    n467 = call "util-ini-key.vi"("key"=ini-key."INI.ENG.INTERVAL_MS" ("input 1")) -> ("key"=w806:string, "section"=w798:string)  [unwired: 9 in]
                    n468 = call-poly <vilib>:"Read Key.vi"("section"=w798, "error in (no error)"=w811, "key"=w806, "refnum"=w809) -> ("error out"=w808:errorcluster, "value"=w799:i32, "found?"=w801:bool, "refnum out"=w807:T64)  [unwired: 4 in]
                    n469 = call <vilib>:"Close Config Data.vi"("error in (no error)"=w808, "refnum"=w807) -> ()  [unwired: 8 in, 2 out]
                    n470 = call "util-path.vi"("Create Folders?(F)"=FALSE, "Selected Folder (PROCS)"=typePathSelector."DIR_INI" ("Selected Folder (PROCEDURE_DIR)")) -> ("error out"=w797:errorcluster, "SelectedPath"=w795:path)  [unwired: 5 in, 3 out]
                    n471 = Select(t=w799, s=w801, f=w802) -> (s? t:f=w800:i32)
                    n472 = call <vilib>:"Open Config Data.vi"("error in (no error)"=w797, "configuration file path"=w795) -> ("error out"=w796:errorcluster, "refnum"=w794:T64)  [unwired: 7 in, 1 out]
                    n473 = call "util-ini-key.vi"("key"=ini-key."INI.ENG.INTERVAL_MS" ("input 1")) -> ("key"=w791:string, "section"=w783:string)  [unwired: 9 in]
                    n474 = local write "ENG ms ctrl 9"(w800) -> ()
                    n475 = call "util-ini-key.vi"("key"=ini-key."INI.LOCAL.LONGITUDE" ("input 1")) -> ("key"=w782:string, "section"=w780:string)  [unwired: 9 in]
                    n476 = call-poly <vilib>:"Read Key.vi"("section"=w783, "error in (no error)"=w796, "key"=w791, "refnum"=w794) -> ("error out"=w793:errorcluster, "value"=w784:i32, "found?"=w786:bool, "refnum out"=w792:T64)  [unwired: 4 in]
                    n477 = call-poly <vilib>:"Write Key.vi"("section"=w780, "value"=w776, "key"=w782, "refnum"=w779) -> ("error out"=w778:errorcluster, "refnum out"=w777:T64)  [unwired: 5 in, 1 out]
                    n478 = call <vilib>:"Close Config Data.vi"("error in (no error)"=w793, "refnum"=w792) -> ()  [unwired: 8 in, 2 out]
                    n479 = Select(t=w784, s=w786, f=w787) -> (s? t:f=w785:i32)
                    n480 = local write "ENG ms ctrl 8"(w785) -> ()
                  }
                  frame #1 {
                    w823 = 500  # timeout ms default
                    w838 = 500  # timeout ms default
                    n481 = call "util-path.vi"("Create Folders?(F)"=FALSE, "Selected Folder (PROCS)"=typePathSelector."DIR_INI" ("Selected Folder (PROCEDURE_DIR)")) -> ("error out"=w848:errorcluster, "SelectedPath"=w846:path)  [unwired: 5 in, 3 out]
                    n482 = call <vilib>:"Open Config Data.vi"("error in (no error)"=w848, "configuration file path"=w846) -> ("error out"=w847:errorcluster, "refnum"=w845:T64)  [unwired: 7 in, 1 out]
                    n483 = call "util-ini-key.vi"("key"=ini-key."INI.ENG.INTERVAL_MS" ("input 1")) -> ("key"=w842:string, "section"=w834:string)  [unwired: 9 in]
                    n484 = call-poly <vilib>:"Read Key.vi"("section"=w834, "error in (no error)"=w847, "key"=w842, "refnum"=w845) -> ("error out"=w844:errorcluster, "value"=w835:i32, "found?"=w837:bool, "refnum out"=w843:T64)  [unwired: 4 in]
                    n485 = call <vilib>:"Close Config Data.vi"("error in (no error)"=w844, "refnum"=w843) -> ()  [unwired: 8 in, 2 out]
                    n486 = call "util-path.vi"("Create Folders?(F)"=FALSE, "Selected Folder (PROCS)"=typePathSelector."DIR_INI" ("Selected Folder (PROCEDURE_DIR)")) -> ("error out"=w833:errorcluster, "SelectedPath"=w831:path)  [unwired: 5 in, 3 out]
                    n487 = Select(t=w835, s=w837, f=w838) -> (s? t:f=w836:i32)
                    n488 = call <vilib>:"Open Config Data.vi"("error in (no error)"=w833, "configuration file path"=w831) -> ("error out"=w832:errorcluster, "refnum"=w830:T64)  [unwired: 7 in, 1 out]
                    n489 = call "util-ini-key.vi"("key"=ini-key."INI.ENG.INTERVAL_MS" ("input 1")) -> ("key"=w827:string, "section"=w819:string)  [unwired: 9 in]
                    n490 = call "util-ini-key.vi"("key"=ini-key."INI.LOCAL.LATITUDE" ("input 1")) -> ("key"=w818:string, "section"=w816:string)  [unwired: 9 in]
                    n491 = local write "ENG ms ctrl 11"(w836) -> ()
                    n492 = call-poly <vilib>:"Read Key.vi"("section"=w819, "error in (no error)"=w832, "key"=w827, "refnum"=w830) -> ("error out"=w829:errorcluster, "value"=w820:i32, "found?"=w822:bool, "refnum out"=w828:T64)  [unwired: 4 in]
                    n493 = call-poly <vilib>:"Write Key.vi"("section"=w816, "value"=w813, "key"=w818, "refnum"=w814) -> ("error out"=w815:errorcluster)  [unwired: 5 in, 2 out]
                    n494 = call <vilib>:"Close Config Data.vi"("error in (no error)"=w829, "refnum"=w828) -> ()  [unwired: 8 in, 2 out]
                    n495 = Select(t=w820, s=w822, f=w823) -> (s? t:f=w821:i32)
                    n496 = local write "ENG ms ctrl 10"(w821) -> ()
                  }
                  frame #2 {
                    w859 = 500  # timeout ms default
                    w874 = 500  # timeout ms default
                    n497 = call "util-path.vi"("Create Folders?(F)"=FALSE, "Selected Folder (PROCS)"=typePathSelector."DIR_INI" ("Selected Folder (PROCEDURE_DIR)")) -> ("error out"=w884:errorcluster, "SelectedPath"=w882:path)  [unwired: 5 in, 3 out]
                    n498 = call <vilib>:"Open Config Data.vi"("error in (no error)"=w884, "configuration file path"=w882) -> ("error out"=w883:errorcluster, "refnum"=w881:T64)  [unwired: 7 in, 1 out]
                    n499 = call "util-ini-key.vi"("key"=ini-key."INI.ENG.INTERVAL_MS" ("input 1")) -> ("key"=w878:string, "section"=w870:string)  [unwired: 9 in]
                    n500 = call-poly <vilib>:"Read Key.vi"("section"=w870, "error in (no error)"=w883, "key"=w878, "refnum"=w881) -> ("error out"=w880:errorcluster, "value"=w871:i32, "found?"=w873:bool, "refnum out"=w879:T64)  [unwired: 4 in]
                    n501 = call <vilib>:"Close Config Data.vi"("error in (no error)"=w880, "refnum"=w879) -> ()  [unwired: 8 in, 2 out]
                    n502 = call "util-path.vi"("Create Folders?(F)"=FALSE, "Selected Folder (PROCS)"=typePathSelector."DIR_INI" ("Selected Folder (PROCEDURE_DIR)")) -> ("error out"=w869:errorcluster, "SelectedPath"=w867:path)  [unwired: 5 in, 3 out]
                    n503 = Select(t=w871, s=w873, f=w874) -> (s? t:f=w872:i32)
                    n504 = call <vilib>:"Open Config Data.vi"("error in (no error)"=w869, "configuration file path"=w867) -> ("error out"=w868:errorcluster, "refnum"=w866:T64)  [unwired: 7 in, 1 out]
                    n505 = call "util-ini-key.vi"("key"=ini-key."INI.ENG.INTERVAL_MS" ("input 1")) -> ("key"=w863:string, "section"=w855:string)  [unwired: 9 in]
                    n506 = local write "ENG ms ctrl 13"(w872) -> ()
                    n507 = call "util-ini-key.vi"("key"=ini-key."INI.LOCAL.TIMEZONE" ("input 1")) -> ("key"=w854:string, "section"=w852:string)  [unwired: 9 in]
                    n508 = call-poly <vilib>:"Read Key.vi"("section"=w855, "error in (no error)"=w868, "key"=w863, "refnum"=w866) -> ("error out"=w865:errorcluster, "value"=w856:i32, "found?"=w858:bool, "refnum out"=w864:T64)  [unwired: 4 in]
                    n509 = call-poly <vilib>:"Write Key.vi"("section"=w852, "value"=w849, "key"=w854, "refnum"=w851) -> ("error out"=w850:errorcluster)  [unwired: 5 in, 2 out]
                    n510 = call <vilib>:"Close Config Data.vi"("error in (no error)"=w865, "refnum"=w864) -> ()  [unwired: 8 in, 2 out]
                    n511 = Select(t=w856, s=w858, f=w859) -> (s? t:f=w857:i32)
                    n512 = local write "ENG ms ctrl 12"(w857) -> ()
                  }
                  frame #3 {
                    w895 = 500  # timeout ms default
                    w910 = 500  # timeout ms default
                    n513 = call "util-path.vi"("Create Folders?(F)"=FALSE, "Selected Folder (PROCS)"=typePathSelector."DIR_INI" ("Selected Folder (PROCEDURE_DIR)")) -> ("error out"=w920:errorcluster, "SelectedPath"=w918:path)  [unwired: 5 in, 3 out]
                    n514 = call <vilib>:"Open Config Data.vi"("error in (no error)"=w920, "configuration file path"=w918) -> ("error out"=w919:errorcluster, "refnum"=w917:T64)  [unwired: 7 in, 1 out]
                    n515 = call "util-ini-key.vi"("key"=ini-key."INI.ENG.INTERVAL_MS" ("input 1")) -> ("key"=w914:string, "section"=w906:string)  [unwired: 9 in]
                    n516 = call-poly <vilib>:"Read Key.vi"("section"=w906, "error in (no error)"=w919, "key"=w914, "refnum"=w917) -> ("error out"=w916:errorcluster, "value"=w907:i32, "found?"=w909:bool, "refnum out"=w915:T64)  [unwired: 4 in]
                    n517 = call <vilib>:"Close Config Data.vi"("error in (no error)"=w916, "refnum"=w915) -> ()  [unwired: 8 in, 2 out]
                    n518 = call "util-path.vi"("Create Folders?(F)"=FALSE, "Selected Folder (PROCS)"=typePathSelector."DIR_INI" ("Selected Folder (PROCEDURE_DIR)")) -> ("error out"=w905:errorcluster, "SelectedPath"=w903:path)  [unwired: 5 in, 3 out]
                    n519 = Select(t=w907, s=w909, f=w910) -> (s? t:f=w908:i32)
                    n520 = call <vilib>:"Open Config Data.vi"("error in (no error)"=w905, "configuration file path"=w903) -> ("error out"=w904:errorcluster, "refnum"=w902:T64)  [unwired: 7 in, 1 out]
                    n521 = call "util-ini-key.vi"("key"=ini-key."INI.ENG.INTERVAL_MS" ("input 1")) -> ("key"=w899:string, "section"=w891:string)  [unwired: 9 in]
                    n522 = local write "ENG ms ctrl 15"(w908) -> ()
                    n523 = call "util-ini-key.vi"("key"=ini-key."INI.PROJECT_NAME" ("input 1")) -> ("key"=w890:string, "section"=w888:string)  [unwired: 9 in]
                    n524 = call-poly <vilib>:"Read Key.vi"("section"=w891, "error in (no error)"=w904, "key"=w899, "refnum"=w902) -> ("error out"=w901:errorcluster, "value"=w892:i32, "found?"=w894:bool, "refnum out"=w900:T64)  [unwired: 4 in]
                    n525 = call-poly <vilib>:"Write Key.vi"("section"=w888, "value"=w886, "key"=w890, "refnum"=w887) -> ("error out"=w885:errorcluster)  [unwired: 5 in, 2 out]
                    n526 = call <vilib>:"Close Config Data.vi"("error in (no error)"=w901, "refnum"=w900) -> ()  [unwired: 8 in, 2 out]
                    n527 = Select(t=w892, s=w894, f=w895) -> (s? t:f=w893:i32)
                    n528 = local write "ENG ms ctrl 14"(w893) -> ()
                  }
                }
                n529 = Merge Errors(w773, w772, w771, w766) -> (w765:errorcluster)
              }
              frame Error {
              }
            }
            n530 = call <vilib>:"Close Config Data.vi"("error in (no error)"=w758, "refnum"=w757) -> ("error out"=w750:errorcluster)  [unwired: 8 in, 1 out]
            n531 = Merge Errors(w750, w751) -> (w749:errorcluster)
            n532 = case shown="No Error" w749 {
              tunnel: w746 -> [w764 _]
              frame No Error {
                n533 = global write "globals-engine.vi" "ProjectSettings"(w764) -> ()
              }
              frame Error {
              }
            }
          }
          event "read buffer": Value Change {
            w926 = T80 4 items=["(0) RxStart", "(1) XOR", "(2) DataSize", "(3) Address", "(4) Type"] ("Enum")
            w927 = T80 3 items=["(0) RxStart", "(1) XOR", "(2) DataSize", "(3) Address", "(4) Type"] ("Enum")
            w928 = T80 2 items=["(0) RxStart", "(1) XOR", "(2) DataSize", "(3) Address", "(4) Type"] ("Enum")
            w923 = T42 {"ADDR"=0, "Label"="Name", "Type"=enum."DI", "Mode"=enum."RIO", "Value"="Value", "Tags"="Tags", "calibration"=[]} ("IoConf in")
            n534 = event-data() -> ()  [unwired: 1 in, 1 out]
            n535 = Unbundle By Name(w923) -> ("Type"=w936:T3)
            n536 = String To Byte Array(string="read buffer") -> (unsigned byte array=w930:u8[])
            n537 = call "io.responseValidator.vi"("ResponsToValidate in"="read buffer", "IoConf in 2"=w923) -> ("error out"=w934:errorcluster, "Data out"=w935:string)  [unwired: 8 in]
            "Command Payload" <- w935
            n538 = Index Array(array=w930, index #1=w928, index #2=w927, index #3=w926) -> (element #1=→"Data Size":u8, element #2=→"Address":u8, element #3=→"Type":u8)
            n539 = case "parse response" shown="\"DI\"" w936 {
              tunnel: w935 -> [_ w939 w949]
              tunnel: [w937 w943 w948] -> _
              tunnel: [_ w942 w947] -> w933
              tunnel: w923 -> [_ w938 w946]
              tunnel: [_ _ w945] -> w932
              tunnel: [_ w941 _] -> _
              tunnel: w934 -> [w937 w940 w944]
              frame Default {
              }
              frame "DI" {
                n540 = call "io.command-parser.DI.vi"("error in (no error)"=w940, "Reponse in"=w939, "IoConf out"=w938) -> ("error out"=w943:errorcluster, "dports"=w941:bool[], "DI out"=w942:dbl)  [unwired: 6 in]
              }
              frame "AI" {
                # "Parse Analog In responses,  (1) filter min/max and \n(2) average the rest"
                n541 = call "io.command-parser.AI.vi"("error in"=w944, "Reponse in"=w949, "IoConf in"=w946) -> ("error out"=w948:errorcluster, "AI uncalib out"=w945:u16, "AI out"=w947:dbl)  [unwired: 6 in]
              }
            }
            "AI out" <- w933
            "AI uncalib out" <- w932
          }
          event "Section": Value Change {
            n542 = event-data() -> ()  [unwired: 1 in, 1 out]
            n543 = local write "indoorStatus"(T27 {"Tdry"="", "Twet"="", "Humidity"=""} ("OutdoorStatus 3")) -> ()
          }
          event "SerialPort": Value Change {
            n544 = event-data() -> ("OldVal"=w953:refnum<visa-resource-name>, "NewVal"=w952:refnum<visa-resource-name>)  [unwired: 1 in]
            n545 = call "util-serial-init.vi"("NewVal"=w952, "Port"=w953) -> ("error out"=w951:errorcluster)  [unwired: 9 in]
          }
          event "Show Undefined": Value Change {
            w954 = "" ("By Tag")
            n546 = event-data() -> ()  [unwired: 1 in, 1 out]
            n547 = local read "IO Search Map"() -> (w956:T41)
            n548 = Bundle By Name(cluster=w956, "By Name"=w954, "By Tag"=w954) -> (w955:T41)
            n549 = property on="IO Search Map" class="Clust (strict)"("Val(Sgnl)"=w955) -> ()  [unwired: 2 in, 2 out]
            n550 = disable-structure shown="Disabled" {
              frame Disabled {
                n551 = local read "IO Search Conf"() -> (w957:T45)
                n552 = property on="IO Search Conf" class="Clust (strict)"("Val(Sgnl)"=w957) -> ()  [unwired: 2 in, 2 out]
              }
              frame Enabled {
              }
            }
          }
          event "Simulate Clock Reset": Value Change {
            n553 = event-data() -> ()  [unwired: 1 in, 1 out]
            n554 = local write "Clk Simulator"(timestamp(0 s since 1904-01-01) ("Time Stamp")) -> ()
          }
          event "Simulators": Value Change {
            n555 = event-data() -> ("OldVal"=w960:cluster{"Input ":string, "Value":string}[], "NewVal"=w959:cluster{"Input ":string, "Value":string}[])  [unwired: 1 in, 1 out]
            n556 = Not Equal?(x=w960, y=w959) -> (x != y?=w961:cluster{"Input ":bool, "Value":bool}[])
            n557 = disable-structure shown="Enabled" {
              disable-tunnel: w961 -> [w969 _]
              disable-tunnel: w959 -> [w964 _]
              frame Disabled {
                n558 = Array Max & Min(array=w969) -> (max index (indices)=w968:i32)  [unwired: 3 out]
                n559 = Index Array(array=w969, index=w968) -> ()  [unwired: 1 out]
                n560 = Index Array(array=w964, index=w968) -> (element=w966:cluster{"Input ":string, "Value":string})
                n561 = Unbundle By Name(w966) -> ("Input"=w965:string)  [unwired: 1 out]
                n562 = call "variantCtrlIo.vi"("isRequired (T)"=FALSE, "menu (Get Param)"=enumVarCtrlIO."IO Get By Key" ("menu (get)"), "Key (use IOnode Label if empty )"=w965) -> ()  [unwired: 4 in, 5 out]
              }
              frame Enabled {
              }
            }
            n563 = for {
              tunnel: [w971] -> w962 if=w970
              tunnel: w959 -> [w974] mode=indexing
              n564 = Unbundle By Name(w974) -> ("Input"=w972:string, "Value"=w973:string)
              n565 = case shown="Default" w972 {
                selector: w972 -> [_ w979]
                tunnel: [_ w977] -> w971
                tunnel: w973 -> [_ w981]
                frame "" {
                  # "empty input when input is cleared - ignore it"
                }
                frame Default {
                  # "Access HW if Empty"
                  # "validate input name is not empty"
                  n566 = call "variantCtrlIo.vi"("menu (Get Param)"=enumVarCtrlIO."IO Get By Key", "Key (use IOnode Label if empty )"=w979) -> ("error out"=w988:errorcluster, "IOnode out"=w985:T42)  [unwired: 5 in, 3 out]
                  n567 = Empty String/Path?(string/path=w981) -> (empty?=w986:bool)
                  n568 = Select(t=enum.io.mode."RIO", s=w986, f=enum.io.mode."SIM" ("Mode")) -> (s? t:f=w987:T38)
                  n569 = Bundle By Name(cluster=w985, "Value"=w981, "Mode"=w987) -> (w975:T42)
                  n570 = call "variantCtrlIo.vi"("menu (Get Param)"=enumVarCtrlIO."IO Modify Value By Key" ("menu (get)"), "error in"=w988, "IOnode in"=w975) -> ("error out"=w978:errorcluster)  [unwired: 4 in, 4 out]
                  n571 = call "variantCtrlIo.vi"("menu (Get Param)"=enumVarCtrlIO."IO Modify Mode By Key" ("menu (get)"), "error in"=w978, "IOnode in"=w975) -> ("error out"=w977:errorcluster)  [unwired: 4 in, 4 out]
                }
              }
              n572 = Unbundle By Name(w971) -> ("status"=w970:bool)
            }
          }
          event "Tab NTR": Value Change {
            n573 = event-data() -> ()  [unwired: 1 in, 1 out]
            n574 = case shown="\"Nutrition\"" "Tab NTR" {
              frame "Nutrition Flow", Default {
              }
              frame "Nutrition" {
                n575 = call "util.ntr.dose-aux.vi"() -> ("DO Dose pumps"=w994:string[])  [unwired: 7 in, 4 out]
                n576 = call "util-path.vi"("Selected Folder (PROCS)"=typePathSelector."DIR_RECORD", "append path (ie. folder\\filename.*)"="NTR\\NUTRITION" ("append path (ie. folder\\filename.*)")) -> ("SelectedPath"=w991:path)  [unwired: 5 in, 4 out]
                n577 = List Folder(path=w991) -> (folder names=w990:string[])  [unwired: 3 in, 3 out]
                n578 = Index Array(array=w990) -> (element=w995:string)  [unwired: 1 in]
                n579 = property on="ntrInputSelect" class="CmbBox"("Strings[]"=w990, "Value"=w995) -> ()  [unwired: 2 in, 2 out]
                n580 = Index Array(array=w994) -> (element=w996:string)  [unwired: 1 in]
                n581 = property on="ntrDosepumpSelect" class="CmbBox"("Strings[]"=w994, "Value"=w996) -> ()  [unwired: 2 in, 2 out]
              }
            }
          }
          event "Graph Panel": Value Change {
            n582 = event-data() -> ("NewVal"=w1011:T25)  [unwired: 1 in]
            n583 = local read "Section"() -> (w1005:string)
            n584 = property on="refresh" class="Bool (strict)"("Value"=FALSE) -> ()  [unwired: 2 in, 2 out]
            n585 = Unbundle By Name(w1011) -> ("lastDays"=w1000:i8)
            n586 = stacked-sequence {
              tunnel: w1011 -> [_ _ _ _ _]
              tunnel: [w1015 _ _ _ _] -> w1010
              tunnel: [w1013 _ _ _ _] -> w1009
              tunnel: [_ _ _ w1036 _] -> w1001
              tunnel: [_ _ w1022 _ _] -> w1008
              tunnel: [_ _ _ w1032 _] -> w1006
              tunnel: w1005 -> [_ _ _ w1031 w1048]
              tunnel: [_ _ _ _ w1047] -> w999
              tunnel: [_ _ _ _ w1046] -> w1004
              tunnel: w1000 -> [w1012 w1018 w1020 w1030 w1042]
              tunnel: [_ w1017 _ _ _] -> w998
              tunnel: [_ w1016 _ _ _] -> w997
              frame #0 {
                n587 = call "helper-build-graph.vi"("filename pattern"="_H0_UV_*.rec" ("filename.*"), "lastDays"=w1012) -> ("error out"=w1015:errorcluster, "Multiple Plots (X Array and Y Array)"=w1013:cluster{"X":dbl[], "Y":dbl[]})  [unwired: 7 in, 1 out]
              }
              frame #1 {
                n588 = call "helper-build-graph.vi"("filename pattern"="_H0_WSPD_*.rec" ("filename.*"), "lastDays"=w1018) -> ("error out"=w1016:errorcluster, "Multiple Plots (X Array and Y Array)"=w1017:cluster{"X":dbl[], "Y":dbl[]})  [unwired: 7 in, 1 out]
              }
              frame #2 {
                w1021 = "_H0" ("string")
                n589 = Concatenate Strings(w1021, "_TDRY_*.rec" ("filename.*")) -> (w1026:string)
                n590 = Concatenate Strings(w1021, "_TWET_*.rec" ("filename.*")) -> (w1025:string)
                n591 = call "helper-build-graph.vi"("filename pattern"=w1026, "lastDays"=w1020) -> ("Multiple Plots (X Array and Y Array)"=w1028:cluster{"X":dbl[], "Y":dbl[]})  [unwired: 7 in, 2 out]
                n592 = call "helper-build-graph.vi"("filename pattern"=w1025, "lastDays"=w1020) -> ("Multiple Plots (X Array and Y Array)"=w1023:cluster{"X":dbl[], "Y":dbl[]})  [unwired: 7 in, 2 out]
                n593 = Build Array(w1028, w1023) -> (w1022:cluster{"X":dbl[], "Y":dbl[]}[])
              }
              frame #3 {
                w1029 = "_" ("string")
                n594 = Concatenate Strings(w1029, w1031, "_TDRY_*.rec" ("filename.*")) -> (w1039:string)
                n595 = Concatenate Strings(w1029, w1031, "_TWET_*.rec" ("filename.*")) -> (w1038:string)
                n596 = call "helper-build-graph.vi"("filename pattern"=w1039, "lastDays"=w1030) -> ("error out"=w1034:errorcluster, "Multiple Plots (X Array and Y Array)"=w1041:cluster{"X":dbl[], "Y":dbl[]})  [unwired: 7 in, 1 out]
                n597 = call "helper-build-graph.vi"("filename pattern"=w1038, "lastDays"=w1030) -> ("error out"=w1033:errorcluster, "Multiple Plots (X Array and Y Array)"=w1035:cluster{"X":dbl[], "Y":dbl[]})  [unwired: 7 in, 1 out]
                n598 = Build Array(w1041, w1035) -> (w1036:cluster{"X":dbl[], "Y":dbl[]}[])
                n599 = Merge Errors(w1034, w1033) -> (w1032:errorcluster)
              }
              frame #4 {
                n600 = Concatenate Strings("_" ("string"), w1048, "_RH_*.rec" ("filename.*")) -> (w1050:string)
                n601 = call "helper-build-graph.vi"("filename pattern"="_H0_RH_*.rec" ("filename.*"), "lastDays"=w1042) -> ("error out"=w1052:errorcluster, "Multiple Plots (X Array and Y Array)"=w1053:cluster{"X":dbl[], "Y":dbl[]})  [unwired: 7 in, 1 out]
                n602 = call "helper-build-graph.vi"("filename pattern"=w1050, "lastDays"=w1042) -> ("error out"=w1044:errorcluster, "Multiple Plots (X Array and Y Array)"=w1043:cluster{"X":dbl[], "Y":dbl[]})  [unwired: 7 in, 1 out]
                n603 = Build Array(w1053, w1043) -> (w1046:cluster{"X":dbl[], "Y":dbl[]}[])
                n604 = Merge Errors(w1052, w1044) -> (w1047:errorcluster)
              }
            }
            "RH" <- w1004
            "UV Graph" <- w1009
            "WindSpeed" <- w998
            n605 = Build Array (concatenate)(w1008, w1001) -> (→"Outdoor Tdry Graph":cluster{"X":dbl[], "Y":dbl[]}[])
            n606 = Merge Errors(w1010, w1006, w999, w997) -> (w1007:errorcluster)
          }
          event "BuilderMenu.templateSave", "BuilderMenu.templateLoad", "BuilderMenu.procedureLoad", "BuilderMenu.procedureSaveAs", "BuilderMenu.procedureSave", "BuilderMenu.procedureReload": Value Change {
            w1060 = TRUE  # allowDialogs?(False)
            # "templateSave (save as text file)\ntemplateLoad (load from text file)\nprocedureSave(build flow and save as varient file)\nprocedureLoad(load from varient file and parse to flow)"
            n607 = event-data() -> ("CtlRef"=w1059:refnum<vi>)  [unwired: 1 in]
            n608 = property class="Bool (strict)"(reference=w1059, "Value"=FALSE) -> ("Label.Text"=w1065:string)  [unwired: 1 in, 2 out]
            n609 = Unbundle By Name("UiBuildProcHead") -> ("Procedure Name"=w1063:string)
            n610 = local read "File path"() -> (w1055:path)
            n611 = call "util-path-to-proc-name.vi"("File path"=w1055) -> ("String"=w1054:string)  [unwired: 10 in]
            n612 = case shown="\"procedureLoad\"" w1065 {
              tunnel: "UiBuildProcHead" -> [w1070 w1086 _ _ _ _ _]
              tunnel: "UiBuildSteps" -> [w1069 w1085 _ _ w1128 w1138 _]
              tunnel: [w1068 w1084 w1102 w1115 w1127 w1136 errorcluster {"status"=TRUE, "code"=-564498, "source"="Case Error in gui.builder.vi's event"} ("error out")] -> w1061
              tunnel: w1063 -> [_ _ _ _ _ w1137 _]
              tunnel: w1060 -> [w1067 w1083 w1100 w1114 _ _ _]
              tunnel: w1054 -> [_ w1079 _ w1110 _ _ _]
              frame "procedureSaveAs" {
                # "procedureSave: build flow and save as varient file"
                n613 = case shown="True" TRUE {
                  tunnel: w1070 -> [_ w1078]
                  tunnel: w1069 -> [_ w1077]
                  tunnel: [_ w1075] -> w1068
                  tunnel: w1067 -> [_ w1072]
                  frame False {
                    # "Cancelled"
                  }
                  frame True {
                    # "Continue"
                    n614 = call "build.proc.vi"("Flow"=w1077, "Proc Head"=w1078) -> ("error out"=w1074:errorcluster, "Instructions"=w1071:variant[])  [unwired: 8 in]
                    n615 = call "util.file.vars.vi"("Operation(Read)"=enum16{"Read File", "Write File"}."Write File", "allowDialogs?(False)"=w1072, "error in"=w1074, "Directory (DIR_PROC)"=typePathSelector."DIR_PROCS" ("location (PROCEDURE_DIR)"), "Vars[] in"=w1071) -> ("error out"=w1075:errorcluster)  [unwired: 2 in, 4 out]
                  }
                }
              }
              frame "procedureSave" {
                # "procedureSave: build flow and save as varient file"
                n616 = Format Into String(format string="Save Procedure as %s?", w1079) -> (resulting string=w1082:string)  [unwired: 2 in, 1 out]
                n617 = Two Button Dialog(message=w1082) -> (T button?=w1080:bool)  [unwired: 2 in]
                n618 = case shown="True" w1080 {
                  tunnel: w1086 -> [_ w1095]
                  tunnel: w1085 -> [_ w1094]
                  tunnel: [_ w1092] -> w1084
                  tunnel: w1083 -> [_ w1089]
                  tunnel: w1079 -> [_ w1088]
                  frame False {
                    # "Cancelled"
                  }
                  frame True {
                    # "Continue"
                    n619 = call "build.proc.vi"("Flow"=w1094, "Proc Head"=w1095) -> ("error out"=w1091:errorcluster, "Instructions"=w1087:variant[])  [unwired: 8 in]
                    n620 = call "util.file.vars.vi"("Operation(Read)"=enum16{"Read File", "Write File"}."Write File", "allowDialogs?(False)"=w1089, "error in"=w1091, "Directory (DIR_PROC)"=typePathSelector."DIR_PROCS" ("location (PROCEDURE_DIR)"), "Proc Name(open dialog if empty)"=w1088, "Vars[] in"=w1087) -> ("error out"=w1092:errorcluster)  [unwired: 1 in, 4 out]
                  }
                }
              }
              frame "procedureLoad" {
                n621 = call "util.file.vars.vi"("allowDialogs?(False)"=w1100, "Directory (DIR_PROC)"=typePathSelector."DIR_PROCS" ("location (PROCEDURE_DIR)")) -> ("error out"=w1101:errorcluster, "cancelled?"=w1099:bool, "Vars[] out"=w1096:variant[], "File path"=w1097:path)  [unwired: 5 in, 1 out]
                n622 = case shown="False" w1099 {
                  tunnel: w1096 -> [w1108 _]
                  tunnel: [w1106 w1109] -> w1102
                  tunnel: w1101 -> [w1105 w1109]
                  tunnel: w1097 -> [w1103 _]
                  frame False {
                    # "not cancelled"
                    n623 = call "build.proc.parse.vi"("error"=w1105, "Array in"=w1108) -> ("error out"=w1106:errorcluster, "Flow Steps"=w1104:T49[], "Proc Head"=w1107:T48)  [unwired: 7 in]
                    n624 = local write "File path"(w1103) -> ()
                    n625 = local write "UiBuildSteps"(w1104) -> ()
                    n626 = local write "UiBuildProcHead"(w1107) -> ()
                  }
                  frame True {
                    # "cancelled"
                  }
                }
              }
              frame "procedureReload" {
                # "procedureSave: build flow and save as varient file"
                n627 = Format Into String(format string="Reload %s?", w1110) -> (resulting string=w1113:string)  [unwired: 2 in, 1 out]
                n628 = Two Button Dialog(message=w1113) -> (T button?=w1111:bool)  [unwired: 2 in]
                n629 = case shown="True" w1111 {
                  tunnel: [_ w1117] -> w1115
                  tunnel: w1114 -> [_ _]
                  tunnel: w1110 -> [_ w1118]
                  frame False {
                    # "Cancelled"
                  }
                  frame True {
                    # "Continue"
                    n630 = Bundle By Name(cluster=cluster{"cmd":T5, "data":variant} {"cmd"=enum."ENG.PROC.RELOAD-BY-NAME", "data"=variant} ("typedefElement"), "data"=w1118) -> (w1116:cluster{"cmd":T5, "data":variant})
                    n631 = global read "globals-engine.vi" "Q-Eng"() -> (w1120:refnum<queue>)
                    n632 = Enqueue Element(queue=w1120, element=w1116) -> (error out=w1117:errorcluster)  [unwired: 2 in, 2 out]
                  }
                }
              }
              frame "templateLoad" {
                n633 = call "util.file.vars.path-parser.vi"("allowDialogs?(False)"=TRUE, "location (PROCEDURE_DIR)"=typePathSelector."DIR_TEMPLATE") -> ("error out"=w1123:errorcluster, "cancelled"=w1121:bool, "selected path"=w1125:path)  [unwired: 7 in]
                n634 = case shown="False" w1121 {
                  tunnel: w1128 -> [w1134 _]
                  tunnel: [w1133 w1135] -> w1127
                  tunnel: enum16{"Read", "Write"}."Read" ("Enum") -> [w1132 _]
                  tunnel: w1125 -> [w1131 _]
                  tunnel: w1123 -> [w1130 w1135]
                  frame False {
                    # "Not cancelled"
                    n635 = call "util.file.template.vi"("error in (no error)"=w1130, "Enum"=w1132, "sensor_flow"=w1134, "file path (dialog if empty)"=w1131) -> ("error out"=w1133:errorcluster, "Array"=w1129:T49[])  [unwired: 5 in, 1 out]
                    n636 = local write "UiBuildSteps"(w1129) -> ()
                  }
                  frame True {
                  }
                }
              }
              frame "templateSave" {
                n637 = stacked-sequence {
                  tunnel: w1138 -> [w1143]
                  tunnel: w1137 -> [_]
                  tunnel: [w1142] -> w1136
                  frame #0 {
                    n638 = call "ui-form-text-line.vi"("User Prompt in"="Enter template name.") -> ("Cancelled?"=w1139:bool, "text out"=w1140:string)  [unwired: 9 in]
                    n639 = case shown="False" w1139 {
                      tunnel: w1143 -> [w1154 _]
                      tunnel: [w1146 _] -> w1142
                      tunnel: w1140 -> [w1144 _]
                      frame False {
                        # "Not Cancelled"
                        n640 = call "util.file.vars.path-parser.vi"("allowDialogs?(False)"=TRUE, "location (PROCEDURE_DIR)"=typePathSelector."DIR_TEMPLATE", "Proc name"=w1144) -> ("selected path"=w1150:path)  [unwired: 6 in, 2 out]
                        n641 = call "util.file.template.vi"("Enum"=enum16{"Read", "Write"}."Write", "sensor_flow"=w1154, "file path (dialog if empty)"=w1150) -> ("error out"=w1147:errorcluster)  [unwired: 6 in, 2 out]
                        n642 = Format Into String(format string="%s saved as template.", initial string="", error in=w1147, w1144) -> (resulting string=w1148:string, error out=w1146:errorcluster)
                        n643 = One Button Dialog(message=w1148) -> ()  [unwired: 1 in, 1 out]
                      }
                      frame True {
                      }
                    }
                  }
                }
              }
              frame Default {
              }
            }
            n644 = call <vilib>:"Clear Errors.vi"("error in (no error)"=w1061, "specific error code to clear (0: all)"=43) -> ("error out"=w1057:errorcluster)  [unwired: 4 in, 1 out]
          }
          event "Title Bar Visible": Value Change {
            n645 = event-data() -> ()  [unwired: 1 in, 1 out]
            n646 = control-ref of="This VI"() -> (w1158:refnum<vi>)
            n647 = property class="VI"(reference=w1158, "Front Panel.TitleBarVis"="Title Bar Visible", "FP.State"=T58."Maximized" ("Front Panel Window:State")) -> ()  [unwired: 1 in, 2 out]
          }
          event "VISA REPORT.Clear": Value Change {
            n648 = event-data() -> ()  [unwired: 1 in, 1 out]
            n649 = call "reg-visa.vi"("Operation(Read)"=enum.report-filter."ClearAll") -> ()  [unwired: 9 in, 2 out]
          }
          event Value Change {
            n650 = event-data() -> ("CtlRef"=w1162:refnum<vi>, "NewVal"=w1165:variant, "OldVal"=w1166:variant)  [unwired: 1 in]
            n651 = property class="Ctl"(reference=w1162) -> (reference out=w1161:refnum<vi>, "Label.Text"=w1163:string)  [unwired: 1 in, 1 out]
            n652 = case shown="\"EastPosition\", \"WestPosition\"" w1163 {
              selector: w1163 -> [_ w1170 _]
              tunnel: w1166 -> [_ w1172 _]
              tunnel: w1165 -> [_ w1175 w1183]
              tunnel: [_ w1174 _] -> w1164
              tunnel: w1161 -> [_ w1173 _]
              tunnel: "WinView" -> [_ w1167 _]
              frame Default {
              }
              frame "EastPosition", "WestPosition" {
                n653 = call "helper-windows-control.vi"("Windows Panel"=w1167, "OldVal"=w1172, "NewVal"=w1175, "Label.Text"=w1170) -> ("error out"=w1174:errorcluster, "oldVal"=w1168:i32, "newVal"=w1169:i32, "canceled?"=w1171:bool)  [unwired: 4 in]
                n654 = case "Operation Canceled?" shown="False" w1171 {
                  tunnel: w1173 -> [_ w1181]
                  tunnel: w1168 -> [_ w1180]
                  tunnel: w1170 -> [w1177 _]
                  tunnel: w1169 -> [w1176 _]
                  frame False {
                    n655 = case "Update Views" shown="\"EastPosition\"" w1177 {
                      tunnel: w1176 -> [_ w1178 w1179]
                      frame Default {
                      }
                      frame "EastPosition" {
                        n656 = property on="EastSideView" class="Slide (strict)"("Value"=w1178) -> ()  [unwired: 2 in, 2 out]
                      }
                      frame "WestPosition" {
                        n657 = property on="WestSideView" class="Slide (strict)"("Value"=w1179) -> ()  [unwired: 2 in, 2 out]
                      }
                    }
                  }
                  frame True {
                    n658 = property class="Ctl"(reference=w1181, "Value"=w1180) -> ()  [unwired: 1 in, 2 out]
                  }
                }
              }
              frame "Stages" {
                (unwired) 0.0 ("Scale.Range:Minimum")
                n659 = Variant To Data(type=0, Variant=w1183) -> (data=w1182:i32)  [unwired: 1 in, 1 out]
                n660 = property on="EastSideView" class="Slide (strict)"("Scale.Maximum"=w1182) -> ()  [unwired: 2 in, 2 out]
                n661 = property on="WestSideView" class="Slide (strict)"("Scale.Maximum"=w1182) -> ()  [unwired: 2 in, 2 out]
                n662 = property on="WestPosition" class="DigNum (strict)"("Maximum"=w1182) -> ()  [unwired: 2 in, 2 out]
                n663 = property on="EastPosition" class="DigNum (strict)"("Maximum"=w1182) -> ()  [unwired: 2 in, 2 out]
              }
            }
          }
          event Menu Selection (User) {
            w1185 = "NTR\\NUTRITION"  # NTR Proce Name
            n664 = event-data() -> ("ItemTag"=w1188:string)  [unwired: 1 in]
            n665 = case shown="\"Exit\"" w1188 {
              selector: w1188 -> [_ _ _ _ _ _ _ w1319 _ _]
              tunnel: w1187 -> [_ _ _ _ w1272 w1278 w1283 _ w1334 _]
              tunnel: [w1189 w1216 w1247 _ w1269 w1275 w1281 _ w1333 _] -> w1186
              tunnel: w1185 -> [_ _ _ _ w1268 w1274 w1282 _ _ _]
              frame "ConfigAux" {
                n666 = vi-ref "config-AUXI.vi"() -> (w1192:refnum<vi>)
                n667 = property class="VI"(reference=w1192) -> (reference out=w1191:refnum<vi>, error out=w1194:errorcluster, "Name"=w1193:string, "Exec.State"=w1190:T81)  [unwired: 1 in]
                n668 = case shown="\"Idle\"" w1190 {
                  tunnel: w1194 -> [w1209 _]
                  tunnel: w1193 -> [w1208 _]
                  tunnel: w1191 -> [_ w1215]
                  tunnel: [w1201 w1212] -> w1189
                  frame "Idle" {
                    n669 = call "variantCtrlIo.vi"("menu (Get Param)"=enumVarCtrlIO."IO List Configs") -> ("IO Configs List"=w1196:T42[])  [unwired: 6 in, 4 out]
                    n670 = call "io-find-by-type.vi"("Mode(Any)"=enum.io.mode."Mode", "Type"=enum.io.type."DO" ("type"), "IOConfigs in"=w1196) -> ("Search Results"=w1200:T42[])  [unwired: 8 in]
                    n671 = for {
                      tunnel: w1200 -> [w1211] mode=indexing
                      tunnel: [w1210] -> w1198 mode=indexing
                      workers-P: _ -> [_]
                      n672 = Unbundle By Name(w1211) -> ("Label"=w1210:string)
                    }
                    n673 = Open VI Reference(type specifier VI Refnum (for type only)=refnum<vi> refnum, vi path=w1208, options=128 ("call and forget"), error in (no error)=w1209) -> (vi reference=w1204:refnum<vi>, error out=w1205:errorcluster)  [unwired: 2 in]
                    n674 = call-by-ref "Start Asynchronous Call"(reference=w1204, error in=w1205, "DO List"=w1198) -> (reference out=w1207:refnum<vi>, error out=w1206:errorcluster)  [unwired: 11 in]
                    n675 = Close Reference(reference=w1207, error in (no error)=w1206) -> (error out=w1201:errorcluster)
                  }
                  frame Default {
                    n676 = invoke class="VI" method="FP.Open"(reference=w1215, "Activate"=TRUE ("Activate?"), "State"=T58."Standard") -> (error out=w1212:errorcluster)  [unwired: 2 in, 4 out]
                  }
                }
              }
              frame "ConfigController" {
                n677 = vi-ref "config-ICC.vi"() -> (w1219:refnum<vi>)
                n678 = property class="VI"(reference=w1219) -> (reference out=w1218:refnum<vi>, error out=w1221:errorcluster, "Name"=w1220:string, "Exec.State"=w1217:T81)  [unwired: 1 in]
                n679 = case shown="\"Idle\"" w1217 {
                  tunnel: w1221 -> [w1239 w1243]
                  tunnel: w1220 -> [w1238 _]
                  tunnel: w1218 -> [_ w1246]
                  tunnel: [w1226 w1242] -> w1216
                  frame "Idle" {
                    w1224 = enum.io.mode."Mode" ("Mode(Any)")
                    n680 = call "variantCtrlIo.vi"("menu (Get Param)"=enumVarCtrlIO."IO List Configs") -> ("IO Configs List"=w1222:T42[])  [unwired: 6 in, 4 out]
                    n681 = call "io-find-by-type.vi"("Mode(Any)"=w1224, "Type"=enum.io.type."DI" ("type"), "IOConfigs in"=w1222) -> ("Search Results"=w1227:T42[])  [unwired: 8 in]
                    n682 = call "io-find-by-type.vi"("Mode(Any)"=w1224, "Type"=enum.io.type."AI" ("type"), "IOConfigs in"=w1222) -> ("Search Results"=w1231:T42[])  [unwired: 8 in]
                    n683 = Build Array (concatenate)(w1231, w1227) -> (w1228:T42[])
                    n684 = for {
                      tunnel: w1228 -> [w1241] mode=indexing
                      tunnel: [w1240] -> w1225 mode=indexing
                      workers-P: _ -> [_]
                      n685 = Unbundle By Name(w1241) -> ("Label"=w1240:string)
                    }
                    n686 = Open VI Reference(type specifier VI Refnum (for type only)=refnum<vi> refnum, vi path=w1238, options=128 ("call and forget"), error in (no error)=w1239) -> (vi reference=w1234:refnum<vi>, error out=w1235:errorcluster)  [unwired: 2 in]
                    n687 = Sort 1D Array(array=w1225) -> ()  [unwired: 1 out]
                    n688 = call-by-ref "Start Asynchronous Call"(reference=w1234, error in=w1235) -> (reference out=w1237:refnum<vi>, error out=w1236:errorcluster)  [unwired: 12 in]
                    n689 = Close Reference(reference=w1237, error in (no error)=w1236) -> (error out=w1226:errorcluster)
                  }
                  frame Default {
                    n690 = invoke class="VI" method="FP.Open"(reference=w1246, error in=w1243, "Activate"=TRUE ("Activate?"), "State"=T58."Standard") -> (error out=w1242:errorcluster)  [unwired: 1 in, 4 out]
                  }
                }
              }
              frame "ConfigNutrition" {
                n691 = disable-structure shown="Disabled" {
                  frame Disabled {
                    n692 = call "config-NTR.vi"() -> ()  [unwired: 12 in]
                  }
                  frame Enabled {
                  }
                }
                n693 = vi-ref "config-NTR.vi"() -> (w1250:refnum<vi>)
                n694 = property class="VI"(reference=w1250) -> (reference out=w1249:refnum<vi>, error out=w1252:errorcluster, "Name"=w1251:string, "Exec.State"=w1248:T81)  [unwired: 1 in]
                n695 = case shown="\"Idle\"" w1248 {
                  tunnel: w1252 -> [w1261 w1263]
                  tunnel: w1251 -> [w1260 _]
                  tunnel: w1249 -> [_ w1266]
                  tunnel: [w1253 w1262] -> w1247
                  frame "Idle" {
                    n696 = Open VI Reference(type specifier VI Refnum (for type only)=refnum<vi> refnum, vi path=w1260, options=128 ("call and forget"), error in (no error)=w1261) -> (vi reference=w1256:refnum<vi>, error out=w1257:errorcluster)  [unwired: 2 in]
                    n697 = call-by-ref "Start Asynchronous Call"(reference=w1256, error in=w1257) -> (reference out=w1259:refnum<vi>, error out=w1258:errorcluster)  [unwired: 12 in]
                    n698 = Close Reference(reference=w1259, error in (no error)=w1258) -> (error out=w1253:errorcluster)
                  }
                  frame Default {
                    n699 = invoke class="VI" method="FP.Open"(reference=w1266, error in=w1263, "Activate"=TRUE ("Activate?"), "State"=T58."Standard") -> (error out=w1262:errorcluster)  [unwired: 1 in, 4 out]
                  }
                }
              }
              frame "IO_Configuration" {
                n700 = disable-structure shown="Disabled" {
                  frame Disabled {
                  }
                  frame Enabled {
                  }
                }
              }
              frame "Nutrition:Pause" {
                n701 = Bundle By Name(cluster=cluster{"cmd":T5, "data":variant} {"cmd"=enum."ENG.PROC.STOP", "data"=variant} ("typedefElement"), "data"=w1268) -> (w1270:cluster{"cmd":T5, "data":variant})
                n702 = Enqueue Element(queue=w1272, element=w1270) -> (error out=w1269:errorcluster)  [unwired: 2 in, 2 out]
                n703 = local write "NTR Status"("Paused" ("ntr.flow-status")) -> ()
              }
              frame "Nutrition:Start" {
                n704 = Bundle By Name(cluster=cluster{"cmd":T5, "data":variant} {"cmd"=enum."ENG.PROC.START", "data"=variant} ("typedefElement"), "data"=w1274) -> (w1276:cluster{"cmd":T5, "data":variant})
                n705 = Enqueue Element(queue=w1278, element=w1276) -> (error out=w1275:errorcluster)  [unwired: 2 in, 2 out]
                n706 = local write "NTR Status"("Starting..." ("ntr.flow-status")) -> ()
              }
              frame "Nutrition:Terminate" {
                n707 = Two Button Dialog(message="Terminate Nutrition Procedure?") -> (T button?=w1279:bool)  [unwired: 2 in]
                n708 = case shown="True" w1279 {
                  tunnel: w1283 -> [_ w1287]
                  tunnel: w1282 -> [_ w1288]
                  tunnel: [_ w1284] -> w1281
                  frame False {
                  }
                  frame True {
                    n709 = stacked-sequence {
                      tunnel: [w1295 _ _ _ _] -> w1292
                      tunnel: w1287 -> [w1294 _ w1301 w1305 w1314]
                      tunnel: [_ w1298 _ _ _] -> w1290
                      tunnel: [_ _ w1302 _ _] -> w1289
                      tunnel: w1288 -> [w1293 _ w1300 w1307 _]
                      tunnel: [_ _ _ w1306 _] -> w1286
                      tunnel: [_ _ _ _ w1313] -> w1285
                      frame #0 {
                        n710 = Bundle By Name(cluster=cluster{"cmd":T5, "data":variant} {"cmd"=enum."ENG.PROC.STOP", "data"=variant} ("typedefElement"), "data"=w1293) -> (w1296:cluster{"cmd":T5, "data":variant})
                        n711 = Enqueue Element(queue=w1294, element=w1296) -> (error out=w1295:errorcluster)  [unwired: 2 in, 2 out]
                      }
                      frame #1 {
                        n712 = global read "globals-engine.vi" "NutritionConfiguration"() -> (w1299:T65[])
                        n713 = call "ntr-init-io.vi"("NutritionConfiguration"=w1299) -> ("error out"=w1298:errorcluster)  [unwired: 10 in]
                      }
                      frame #2 {
                        n714 = Bundle By Name(cluster=cluster{"cmd":T5, "data":variant} {"cmd"=enum."ENG.PROC.RELOAD-BY-NAME", "data"=variant} ("typedefElement"), "data"=w1300) -> (w1304:cluster{"cmd":T5, "data":variant})
                        n715 = Enqueue Element(queue=w1301, element=w1304) -> (error out=w1302:errorcluster)  [unwired: 2 in, 2 out]
                      }
                      frame #3 {
                        n716 = Bundle By Name(cluster=cluster{"cmd":T5, "data":variant} {"cmd"=enum."ENG.PROC.STOP", "data"=variant} ("typedefElement"), "data"=w1307) -> (w1309:cluster{"cmd":T5, "data":variant})
                        n717 = Enqueue Element(queue=w1305, element=w1309) -> (error out=w1306:errorcluster)  [unwired: 2 in, 2 out]
                      }
                      frame #4 {
                        n718 = global read "globals-engine.vi" "Q-Log"() -> (w1311:refnum<queue>)
                        n719 = Bundle("Q-Log"=w1311, "procQ"=cluster{"data":variant, "Enum":T57} {"data"=variant, "Enum"=enum."LOG.INIT.NTR-FLOW"}) -> (w1310:T82)  [unwired: 1 in]
                        n720 = Bundle By Name(cluster=cluster{"cmd":T5, "data":variant} {"cmd"=enum."ENG.EXTERNAL-CALL", "data"=variant} ("typedefElement"), "data"=w1310) -> (w1316:cluster{"cmd":T5, "data":variant})
                        n721 = Enqueue Element(queue=w1314, element=w1316) -> (error out=w1313:errorcluster)  [unwired: 2 in, 2 out]
                      }
                    }
                    n722 = Merge Errors(w1292, w1290, w1289, w1286, w1285) -> (w1284:errorcluster)
                    n723 = local write "NTR Status"("Terminated" ("ntr.flow-status")) -> ()
                  }
                }
              }
              frame "PageAdmin", "PageIO", "PageMain" {
                n724 = case shown="\"PageAdmin\"" w1319 {
                  tunnel: ["MAIN" "I/O" "ADMIN"] -> w1318
                  frame "PageMain", Default {
                  }
                  frame "PageIO" {
                  }
                  frame "PageAdmin" {
                  }
                }
                n725 = property on="Tab Main" class="TabCtl (strict)"() -> ("Pages"=w1320:refnum<vi>[])  [unwired: 2 in, 2 out]
                n726 = for {
                  tunnel: w1320 -> [w1325] mode=indexing
                  tunnel: w1318 -> [w1323]
                  tunnel: [w1322] -> w1317
                  i -> [w1322]
                  stop <- w1321 stop-if-true
                  n727 = property class="Page"(reference=w1325) -> ("PageLabel"=w1324:string)  [unwired: 1 in, 2 out]
                  n728 = Equal?(x=w1324, y=w1323) -> (x = y?=w1321:bool)
                }
                n729 = local write "Tab Main"(w1317) -> ()
              }
              frame "Exit" {
                n730 = global read "globals-engine.vi" "NutritionConfiguration"() -> (w1329:T65[])
                n731 = property on="Stop" class="Bool (strict)"("Val(Sgnl)"=TRUE ("Value (Signaling)")) -> ()  [unwired: 2 in, 2 out]
                n732 = call "ntr-init-io.vi"("NutritionConfiguration"=w1329) -> ("error out"=w1330:errorcluster)  [unwired: 10 in]
                n733 = Enqueue Element(queue=w1334, element=cluster{"cmd":T5, "data":variant} {"cmd"=enum."ENG.EXIT", "data"=variant} ("typedefElement"), error in (no error)=w1330) -> (error out=w1333:errorcluster)  [unwired: 1 in, 2 out]
              }
              frame Default {
              }
            }
          }
          event Timeout; "Timer Reset?": Value Change {
            n734 = event-data() -> ()  [unwired: 1 in, 1 out]
            n735 = stacked-sequence {
              tunnel: [w1337 _ _ _] -> w1336
              tunnel: w1335 -> [_ _ w1394 w1420]
              frame #0 {
                n736 = expression code="x*1000"("TimerSec") -> (w1341:dbl)
                n737 = call "util-timer-inline.vi"("Reset?"="Timer Reset?", "Target[ms]"=w1341) -> ("done?"=w1346:bool, "downcount[sec]"=→"downcount[sec]":dbl)  [unwired: 6 in, 2 out]
                n738 = local read "Tab Main"() -> (w1345:enum32{"MAIN", "I/O", "ADMIN"})
                n739 = local write "Timer Reset?"(w1346) -> ()
                n740 = local read "Tab IO"() -> (w1344:enum32{"Map", "Editor", "Calibration"})
                n741 = call "util-ui-view.vi"("Page2"=w1344, "Page1"=w1345) -> ("Page1:Page2"=w1342:string)  [unwired: 7 in, 2 out]
                n742 = case shown="True" w1346 {
                  tunnel: [_ w1353] -> w1340
                  tunnel: w1342 -> [_ w1355]
                  tunnel: "IO Map Snapshot Enable" -> [_ w1354]
                  tunnel: [_ w1352] -> w1339
                  frame False {
                  }
                  frame True {
                    n743 = stacked-sequence {
                      tunnel: w1355 -> [w1358 _ _ _]
                      tunnel: w1354 -> [w1357 _ w1383 _]
                      tunnel: [w1356 _ _ _] -> w1353
                      tunnel: [_ w1373 _ _] -> w1352
                      frame #0 {
                        n744 = case shown="Default" w1358 {
                          tunnel: [_ w1360 w1363 w1372] -> w1356
                          tunnel: w1357 -> [_ w1359 _ _]
                          frame Default {
                          }
                          frame "I/O:Map" {
                            n745 = case shown="True" w1359 {
                              tunnel: [_ w1361] -> w1360
                              frame False {
                              }
                              frame True {
                                n746 = property on="IO Map Take Snapshot" class="Bool (strict)"("Val(Sgnl)"=TRUE ("Value (Signaling)")) -> (error out=w1361:errorcluster)  [unwired: 2 in, 1 out]
                              }
                            }
                          }
                          frame "I/O:Snapshot" {
                            n747 = disable-structure shown="Disabled" {
                              disable-tunnel: [w1369 _] -> w1363
                              frame Disabled {
                                w1367 = cluster{"cmd":T5, "data":variant} {"cmd"=enum."ENG.RIO.SNAPSHOT", "data"=variant}  # snapshot all
                                n748 = local read item#-1() -> (w1365)
                                n749 = Build Array(w1365) -> (w1364:void[])
                                n750 = global read "globals-engine.vi" "Q-Eng"() -> (w1368:refnum<queue>)
                                n751 = Bundle By Name(cluster=w1367, "data"=w1364) -> (w1366:cluster{"cmd":T5, "data":variant})
                                n752 = Enqueue Element(queue=w1368, element=w1366) -> (error out=w1369:errorcluster)  [unwired: 2 in, 2 out]
                              }
                              frame Enabled {
                              }
                            }
                          }
                          frame "I/O:Calibration" {
                            n753 = global read "globals-engine.vi" "Q-Eng"() -> (w1371:refnum<queue>)
                            n754 = Enqueue Element(queue=w1371, element=cluster{"cmd":T5, "data":variant} {"cmd"=enum."ENG.RIO.AIN-SNAPSHOT-CALIB", "data"=variant} ("typedefElement")) -> (error out=w1372:errorcluster)  [unwired: 2 in, 2 out]
                          }
                        }
                      }
                      frame #1 {
                        n755 = global read "globals-engine.vi" "Q-Com"() -> (w1376:refnum<queue>)
                        n756 = Get Queue Status(queue=w1376) -> (error out=w1374:errorcluster, # elements in queue=→"COM FIFO":i32)  [unwired: 2 in, 6 out]
                        n757 = global read "globals-engine.vi" "Q-Log"() -> (w1381:refnum<queue>)
                        n758 = global read "globals-engine.vi" "Q-Eng"() -> (w1379:refnum<queue>)
                        n759 = Get Queue Status(queue=w1381) -> (error out=w1378:errorcluster, # elements in queue=→"LOG FIFO 2":i32)  [unwired: 2 in, 6 out]
                        n760 = Get Queue Status(queue=w1379) -> (error out=w1377:errorcluster, # elements in queue=→"ENG FIFO 2":i32)  [unwired: 2 in, 6 out]
                        n761 = Merge Errors(w1374, w1378, w1377) -> (w1373:errorcluster)
                      }
                      frame #2 {
                        n762 = case shown="False" w1383 {
                          frame False {
                          }
                          frame True {
                            n763 = property on="IO Map Take Snapshot" class="Bool (strict)"("Val(Sgnl)"=TRUE ("Value (Signaling)")) -> ()  [unwired: 2 in, 2 out]
                          }
                        }
                      }
                      frame #3 {
                        n764 = global read "globals-engine.vi" "Q-Log"() -> (w1387:refnum<queue>)
                        n765 = Enqueue Element(queue=w1387, element=cluster{"data":variant, "Enum":T57} {"data"=variant, "Enum"=enum."LOG.UPDATE.IRR"} ("procQ")) -> (error out=w1386:errorcluster)  [unwired: 2 in, 2 out]
                        n766 = call <vilib>:"Clear Errors.vi"("error in (no error)"=w1386) -> ()  [unwired: 5 in, 2 out]
                      }
                    }
                  }
                }
                n767 = Merge Errors(w1340, w1339) -> (w1338:errorcluster)
                n768 = flat-sequence {
                  tunnel: [w1350] -> w1337
                  tunnel: w1338 -> [w1350]
                  frame #0 {
                    n769 = property on="Timer Reset?" class="Bool (strict)"("Value"=FALSE ("Timer Reset?")) -> ()  [unwired: 2 in, 2 out]
                  }
                }
              }
              frame #1 {
                n770 = case shown="False" FALSE {
                  frame False {
                  }
                  frame True {
                    n771 = Unbundle By Name("VISA REPORT") -> ("VISA Report En"=w1390:bool)
                    n772 = case shown="True" w1390 {
                      tunnel: "VISA REPORT" -> [_ w1391]
                      frame False {
                      }
                      frame True {
                        n773 = call "helper-log-visa.vi"("VISA REPORT"=w1391) -> ("array type (2D Dbl)"=w1392:string[][])  [unwired: 9 in, 1 out]
                        n774 = property on="visa report" class="Tbl (strict)"("Value"=w1392) -> ()  [unwired: 2 in, 2 out]
                      }
                    }
                  }
                }
              }
              frame #2 {
                w1395 = "%d/%m/%y" ("time format string (%c)")
                # "PBR"
                n775 = local read "last"() -> (w1397:T17)
                n776 = Format Date/Time String(time format string (%c)=w1395, seconds (now)=w1397) -> (date/time string=w1396:string)  [unwired: 1 in]
                n777 = Format Date/Time String(time format string (%c)=w1395, seconds (now)=w1394) -> (date/time string=w1398:string)  [unwired: 1 in]
                n778 = Not Equal?(x=w1396, y=w1398) -> (x != y?=w1393:bool)
                n779 = First Call?() -> (First Call?: T/F=w1399:bool)
                n780 = feedback #3(TRUE ("Found?")) -> (w1402:bool)
                n781 = Select(t=FALSE ("Found?"), s=w1393, f=w1402) -> (s? t:f=w1403:bool)
                n782 = Or(x=w1403, y=w1399) -> (x .or. y?=w1400:bool)
                n783 = case shown="False" w1400 {
                  selector: w1400 -> [_ w1418]
                  tunnel: [w1408 w1418] -> w1401
                  tunnel: w1394 -> [w1407 _]
                  frame False {
                    n784 = Add(x="start", y=60.0) -> (x+y=w1413:T17)
                    n785 = Bundle By Name(cluster=cluster{"start":T17, "stop":T17} {"start"=timestamp(0 s since 1904-01-01), "stop"=timestamp(0 s since 1904-01-01)} ("sched-pairs"), "start"="start", "stop"=w1413) -> (w1414:cluster{"start":T17, "stop":T17})
                    n786 = Build Array(w1414) -> (w1415:cluster{"start":T17, "stop":T17}[])
                    n787 = call "sched-check-compare.vi"("sched-mode"=enum16{"Hourly", "Daily", "Weekly", "Date"}."Daily", "sched-pairs"=w1415, "time stamp"=w1407) -> ("Time"=w1406:timestamp, "Found?"=w1408:bool)  [unwired: 5 in, 2 out]
                    n788 = case shown="False" w1408 {
                      selector: w1408 -> [_ w1416]
                      tunnel: w1406 -> [_ _]
                      frame False {
                      }
                      frame True {
                        n789 = disable-structure shown="Disabled" {
                          disable-tunnel: w1416 -> [_ _]
                          frame Disabled {
                            n790 = call-poly <vilib>:"Write Delimited Spreadsheet.vi"("append to file? (new file:F)"=TRUE) -> ()  [unwired: 13 in, 2 out]
                          }
                          frame Enabled {
                          }
                        }
                        n791 = property on="Harvest" class="Bool (strict)"("Val(Sgnl)"=w1416) -> ()  [unwired: 2 in, 2 out]
                      }
                    }
                  }
                  frame True {
                  }
                }
                n792 = feedback-in #3(w1401) -> ()
              }
              frame #3 {
                # "sun/moon indicator"
                n793 = call "irr-sunrise-calc.vi"("Time Stamp"=w1420) -> ("(T) Day (F) Night"=→"DayNight":bool)  [unwired: 7 in, 3 out]
              }
            }
          }
          event "UVAccHistoryDays", "UvAccRefresh": Value Change {
            n794 = event-data() -> ()  [unwired: 1 in, 1 out]
            n795 = call "helper-build-graph.vi"("Row(2)"=1, "Module (OCS)"="IRR\\db", "filename pattern"="_UV_ACC_*.rec" ("filename.*"), "lastDays"="UVAccHistoryDays") -> ("error out"=w1423:errorcluster, "Multiple Plots (X Array and Y Array)"=→"UV_ACC":cluster{"X":dbl[], "Y":dbl[]})  [unwired: 5 in, 1 out]
            n796 = call <vilib>:"Clear Errors.vi"("error in (no error)"=w1423) -> ("error out"=w1421:errorcluster)  [unwired: 5 in, 1 out]
          }
          event "RFS SetX1": Value Change {
            n797 = event-data() -> ()  [unwired: 1 in, 1 out]
            n798 = global read "globals-engine.vi" "Q-Eng"() -> (w1429:refnum<queue>)
            n799 = Enqueue Element(queue=w1429, element=cluster{"cmd":T5, "data":variant} {"cmd"=enum."ENG.RIO.RFS-DELAY-SET-X1", "data"=variant} ("typedefElement")) -> (error out=w1428:errorcluster)  [unwired: 2 in, 2 out]
          }
          event "RFS SetX8": Value Change {
            n800 = event-data() -> ()  [unwired: 1 in, 1 out]
            n801 = global read "globals-engine.vi" "Q-Eng"() -> (w1432:refnum<queue>)
            n802 = Enqueue Element(queue=w1432, element=cluster{"cmd":T5, "data":variant} {"cmd"=enum."ENG.RIO.RFS-DELAY-SET-X8", "data"=variant} ("typedefElement")) -> (error out=w1431:errorcluster)  [unwired: 2 in, 2 out]
          }
          event "RFS Cycles Set": Value Change {
            n803 = event-data() -> ()  [unwired: 1 in, 1 out]
            n804 = global read "globals-engine.vi" "Q-Eng"() -> (w1435:refnum<queue>)
            n805 = Enqueue Element(queue=w1435, element=cluster{"cmd":T5, "data":variant} {"cmd"=enum."ENG.RIO.RFS-CYCLES-SET", "data"=variant} ("typedefElement")) -> (error out=w1434:errorcluster)  [unwired: 2 in, 2 out]
          }
          event "RFS Cycles Get": Value Change {
            n806 = event-data() -> ()  [unwired: 1 in, 1 out]
            n807 = global read "globals-engine.vi" "Q-Eng"() -> (w1438:refnum<queue>)
            n808 = Enqueue Element(queue=w1438, element=cluster{"cmd":T5, "data":variant} {"cmd"=enum."ENG.RIO.RFS-CYCLES-GET", "data"=variant} ("typedefElement")) -> (error out=w1437:errorcluster)  [unwired: 2 in, 2 out]
          }
          event "RFS Enable Table": Value Change {
            n809 = event-data() -> ()  [unwired: 1 in, 1 out]
            n810 = global read "globals-engine.vi" "Q-Eng"() -> (w1441:refnum<queue>)
            n811 = Enqueue Element(queue=w1441, element=cluster{"cmd":T5, "data":variant} {"cmd"=enum."ENG.RIO.RFS-ENABLE", "data"=variant} ("typedefElement")) -> (error out=w1440:errorcluster)  [unwired: 2 in, 2 out]
          }
          event "EngLogClear": Value Change {
            n812 = event-data() -> ()  [unwired: 1 in, 1 out]
            n813 = call "reg-eng-calls.vi"("Operation(Read)"=enum.report-filter."ClearAll") -> ("error out"=w1443:errorcluster, "Collected Reports"=w1444:string)  [unwired: 9 in]
            n814 = local write "Collected Reports"(w1444) -> ()
          }
        }
        n815 = case shown="\"\"" w134 {
          selector: w134 -> [_ w140]
          frame "" {
            # "skip empty statuts"
          }
          frame Default {
            # "status register"
            n816 = call "reg-status.vi"("Operation(Read)"=enum.report-filter."Collect", "Reports to Collect"=w140) -> ("Collected Reports"=w142:string)  [unwired: 8 in, 1 out]
            n817 = local write "User messages"(w142) -> ()
          }
        }
        n818 = call <vilib>:"Simple Error Handler.vi"("type of dialog (OK msg:1)"=w135, "error in (no error)"=w138) -> ()  [unwired: 3 in, 5 out]
        "Event" <- w136
      }
    }
  }
  n819 = while "Time Scheduler" {
    tunnel: w4 -> [w1453]
    tunnel: w2 -> [w1454]
    shift-right: [w1447] -> _
    shift-left: errorcluster[] [] ("Array out") -> [w1451]
    shift-right: [w1449] -> _
    shift-left: _ -> [w1448]
    i -> [w1446]
    stop <- w1458 stop-if-true
    n820 = Get Date/Time In Seconds() -> (seconds since 1Jan1904=w1452:timestamp)
    n821 = Dequeue Element(queue=w1453, timeout in ms (-1)=300, error in (no error)=w1454) -> (queue out=w1457:refnum<queue>, element=w1459:cluster{"data":variant, "Enum":T54}, timed out?=w1456:bool, error out=w1460:errorcluster)
    n822 = case shown="No Error" w1460 {
      selector: w1460 -> [_ w1512]
      tunnel: w1459 -> [w1467 _]
      tunnel: [w1464 _] -> w1458
      tunnel: w1457 -> [w1468 _]
      tunnel: w1456 -> [w1466 _]
      tunnel: [w1465 w1512] -> w1450
      tunnel: w1452 -> [w1461 _]
      tunnel: [w1463 w1511] -> w1449
      tunnel: w1448 -> [w1462 w1511]
      frame No Error {
        n823 = case shown="True" w1466 {
          tunnel: w1468 -> [_ w1497]
          tunnel: w1467 -> [_ w1495]
          tunnel: [w1470 w1493] -> w1465
          tunnel: [_ w1496] -> w1464
          tunnel: [w1472 w1490] -> w1463
          tunnel: w1462 -> [w1471 w1489]
          tunnel: w1461 -> [w1474 _]
          frame True {
            # "Queue Timeout\n- COMPARE TIME ELEMENTS -"
            n824 = for "COMPARE TIME(S) - RETURN POSITIVE PROCS" {
              tunnel: w1471 -> [w1486] mode=indexing
              tunnel: w1474 -> [w1485]
              tunnel: [w1488] -> w1473 mode=indexing if=w1487
              tunnel: [w1486] -> w1469 mode=indexing
              n825 = Unbundle By Name(w1486) -> ("Proc Name"=w1488:string, "Time"=w1483:timestamp)
              n826 = call "util-daily-seconds.vi"("seconds since 1Jan1904"=w1485) -> ("Numeric"=w1484:i32)  [unwired: 10 in]
              n827 = call "util-daily-seconds.vi"("seconds since 1Jan1904"=w1483) -> ("Numeric"=w1482:i32)  [unwired: 10 in]
              n828 = Equal?(x=w1484, y=w1482) -> (x = y?=w1487:bool)
            }
            "Schedulers" <- w1469
            n829 = for "REMOVE POSITIVE ELEMENTS FROM MAP AND SIGNAL ENG" {
              shift-right: [w1480] -> w1472
              shift-left: w1471 -> [w1481]
              tunnel: w1473 -> [w1477] mode=indexing
              tunnel: [w1475] -> w1470
              stop <- w1475 stop-if-true
              n830 = global read "globals-engine.vi" "Q-Eng"() -> (w1479:refnum<queue>)
              n831 = Bundle By Name(cluster=cluster{"cmd":T5, "data":variant} {"cmd"=enum."ENG.PROC.START", "data"=variant} ("typedefElement"), "data"=w1477) -> (w1476:cluster{"cmd":T5, "data":variant})
              n832 = Remove From Map(10:w1477, 11:w1481) -> (3:w1480:map{string, timestamp})  [unwired: 2 out]
              n833 = Enqueue Element(queue=w1479, element=w1476) -> (error out=w1475:errorcluster)  [unwired: 2 in, 2 out]
            }
          }
          frame False {
            # "Message Handler"
            n834 = Unbundle(w1495) -> ("data"=w1494:variant, "Enum"=w1492:T54)
            n835 = case shown="\"SCHED.REGISTER\"" w1492 {
              tunnel: w1497 -> [w1500 _ _ _]
              tunnel: [w1499 _ _ _] -> w1493
              tunnel: [TRUE _ _ _] -> w1496
              tunnel: w1494 -> [_ _ w1509 _]
              tunnel: T83 {"Proc Name"="", "Time"=timestamp(0 s since 1904-01-01)} -> [_ _ w1508 _]
              tunnel: [w1498 map{string, timestamp} {} ("map") w1506 w1510] -> w1490
              tunnel: w1489 -> [w1498 _ w1505 w1510]
              frame "SCHED.EXIT" {
                n836 = Release Queue(queue=w1500) -> (error out=w1499:errorcluster)  [unwired: 2 in, 2 out]
              }
              frame "SCHED.INIT" {
                # "BUILD MAP AND SET SHIFT REGISTER"
              }
              frame "SCHED.REGISTER" {
                # "INSERT ELEMENT INTO MAP AND UPDATE SHIFT REGISTER"
                n837 = Variant To Data(type=w1508, Variant=w1509) -> (data=w1507:T83)  [unwired: 1 in, 1 out]
                n838 = Unbundle By Name(w1507) -> ("Proc Name"=w1504:string, "Time"=w1503:timestamp)
                n839 = Insert Into Map(map in=w1505, key=w1504, value=w1503) -> (map out=w1506:map{string, timestamp})  [unwired: 2 out]
              }
              frame Default {
              }
            }
          }
        }
      }
      frame Error {
        # "handle error by displaying a continue/stop message dialog."
      }
    }
    n840 = call "util-collect-error.vi"("error in (no error)"=w1450, "Array in"=w1451) -> ("Array out"=w1447:errorcluster[])  [unwired: 9 in]
    "Scheduler Engine Errors" <- w1447
    "SCHED" <- w1446
  }
  n841 = while "GUI MONITOR" {
    tunnel: w29 -> [w1519]
    tunnel: w32 -> [w1521]
    tunnel: w33 -> [w1520]
    shift-right: [w1514] -> _
    shift-left: errorcluster[] [] ("Array out") -> [w1515]
    i -> [w1516]
    stop <- w1525 stop-if-true
    # "TODO make a general \nerror message \nvi eng vs log"
    n842 = Get Date/Time In Seconds() -> (seconds since 1Jan1904=w1517:timestamp)
    n843 = Dequeue Element(queue=w1519, timeout in ms (-1)=-1, error in (no error)=w1521) -> (queue out=w1524:refnum<queue>, element=w1526:cluster{"data":variant, "Enum":T57}, timed out?=w1523:bool, error out=w1527:errorcluster)
    n844 = case shown="No Error" w1527 {
      selector: w1527 -> [_ w1831]
      tunnel: w1526 -> [w1536 _]
      tunnel: [w1533 _] -> w1525
      tunnel: w1524 -> [w1537 _]
      tunnel: w1523 -> [w1535 _]
      tunnel: [w1534 w1831] -> w1513
      tunnel: w1520 -> [w1532 _]
      tunnel: [w1531 _] -> w1518
      tunnel: w1517 -> [_ _]
      frame No Error {
        n845 = case shown="False" w1535 {
          tunnel: w1537 -> [_ w1546]
          tunnel: w1536 -> [_ w1544]
          tunnel: [_ w1540] -> w1534
          tunnel: [_ w1545] -> w1533
          tunnel: w1532 -> [_ w1542]
          tunnel: [_ w1541] -> w1531
          frame True {
            # "Queue Timeout"
          }
          frame False {
            # "Command Handler"
            n846 = Unbundle(w1544) -> ("data"=w1543:variant, "Enum"=w1538:T57)
            n847 = case shown="\"LOG.UPDATE.SELECTORS\"" w1538 {
              tunnel: w1546 -> [_ w1623 _ _ _ _ _ _ _ _]
              tunnel: [w1556 w1621 _ w1628 _ _ w1708 w1725 w1753 _] -> w1540
              tunnel: [_ TRUE _ _ _ _ _ _ _ _] -> w1545
              tunnel: w1543 -> [w1559 _ _ _ _ w1638 w1709 w1726 _ _]
              tunnel: w1542 -> [_ _ _ _ _ _ _ _ _ _]
              tunnel: [_ _ _ _ _ _ _ _ "Update Irrigation parameters" _] -> w1541
              frame "LOG.CATCH" {
                n848 = Variant To Data(type=T84 {"Procedure(post)"=[], "Procedure(pre)"=[], "Next State "={"CMD"=enum."NEXT", "data"=variant}, "IsRunning"=FALSE, "error in"={"status"=FALSE, "code"=0, "source"=""}} ("cluster"), Variant=w1559) -> (data=w1557:T84)  [unwired: 1 in, 1 out]
                n849 = Unbundle By Name(w1557) -> ("Procedure(post)"=w1555:variant[], "Procedure(pre)"=w1554:variant[], "Next State"=w1553:cluster{"CMD":T85, "data":variant}, "IsRunning"=w1552:bool, "error in"=w1547:errorcluster)
                n850 = call "engine.logger.vi"("isRunning"=w1552, "Proc Error"=w1547, "Next State in"=w1553, "Procedure(pre)"=w1554, "Procedure(post) in"=w1555) -> ("error IO"=w1551:errorcluster, "output cluster"=w1550:T86)  [unwired: 4 in, 1 out]
                n851 = stacked-sequence {
                  tunnel: w1550 -> [w1564 w1577]
                  tunnel: [w1562 _] -> w1549
                  tunnel: [_ w1576] -> w1548
                  frame #0 {
                    # "Catch ANY log"
                    n852 = local read "Admin Panel"() -> (w1560:bool)
                    n853 = call "reg-log-general.vi"("Operation(Read)"=enum.report-filter."Collect", "filter by proc name"="Proc Name", "Reports to Collect"=w1564) -> ("error out"=w1563:errorcluster)  [unwired: 6 in, 2 out]
                    n854 = case shown="True" w1560 {
                      tunnel: w1563 -> [_ w1571]
                      tunnel: [_ w1570] -> w1562
                      tunnel: "Proc Name" -> [_ w1568]
                      frame False {
                      }
                      frame True {
                        n855 = call "reg-log-general.vi"("Operation(Read)"=enum.report-filter."Read ALL", "error in"=w1571, "filter by proc name"=w1568) -> ("error out"=w1570:errorcluster, "compact report"=w1567:T78[])  [unwired: 6 in, 1 out]
                        n856 = case shown="True" "Enable Report" {
                          tunnel: w1567 -> [_ w1572]
                          frame False {
                          }
                          frame True {
                            "Report General" <- w1572
                          }
                        }
                      }
                    }
                  }
                  frame #1 {
                    # "Catch APP log (AUXI, IRR, NTR ... )"
                    n857 = Unbundle By Name(w1577) -> ("Proc Module"=w1575:string, "Step Function"=w1573:T6)
                    n858 = case "Catch by module name (OCS,AUXI,IRR,NTR,...)" shown="\"IRR\"" w1575 {
                      selector: w1575 -> [_ _ w1588 _ _]
                      tunnel: w1577 -> [_ w1582 w1590 w1601 w1609]
                      tunnel: [_ _ w1589 _ _] -> w1576
                      tunnel: "LOG.PARSE." -> [_ _ w1587 _ _]
                      tunnel: w1573 -> [_ _ w1586 _ _]
                      frame Default {
                      }
                      frame "AUXI" {
                        n859 = local read "Tab Main"() -> (w1581:enum32{"MAIN", "I/O", "ADMIN"})
                        n860 = local read "Tab Auxi"() -> (w1580:T30)
                        n861 = Format Into String(format string="%s_%s", w1581, w1580) -> (resulting string=w1579:string)  [unwired: 2 in, 1 out]
                        n862 = case shown="\"MAIN_Auxiliary\"" w1579 {
                          tunnel: w1582 -> [_ w1583]
                          frame Default {
                          }
                          frame "MAIN_Auxiliary" {
                            n863 = local read "AuxiliaryList"() -> (w1584:T33)
                            n864 = call "helper-log-parse-auxi.vi"("log cluster"=w1583, "AuxiliaryList in"=w1584) -> ("AuxiliaryList out"=w1585:T33)  [unwired: 9 in]
                            n865 = local write "AuxiliaryList"(w1585) -> ()
                          }
                        }
                      }
                      frame "OCS" {
                        n866 = case shown="\"_OCS_CHECK\", \"_OCS_RECORD\"" w1586 {
                          tunnel: w1590 -> [_ w1598]
                          tunnel: [_ w1597] -> w1589
                          tunnel: w1588 -> [_ w1596]
                          tunnel: w1587 -> [_ w1594]
                          frame Default {
                          }
                          frame "_OCS_CHECK", "_OCS_RECORD" {
                            n867 = Concatenate Strings(w1594, w1596) -> (w1593:string)
                            n868 = Scan From String(input string=w1593, default 1=state-logger."LOG.NO_OP" ("Enum")) -> (output 1=w1592:T57)  [unwired: 3 in, 3 out]
                            n869 = global read "globals-engine.vi" "Q-Log"() -> (w1599:refnum<queue>)
                            n870 = Bundle By Name(cluster=cluster{"data":variant, "Enum":T57} {"data"=variant, "Enum"=enum."LOG.NO_OP"} ("procQ"), "Enum"=w1592, "data"=w1598) -> (w1600:cluster{"data":variant, "Enum":T57})
                            n871 = Enqueue Element(queue=w1599, element=w1600) -> (error out=w1597:errorcluster)  [unwired: 2 in, 2 out]
                          }
                        }
                      }
                      frame "IRR" {
                        n872 = call "helper-log-parse-irr.vi"("output cluster"=w1601) -> ("Cluster"=w1603:cluster{"sample":dbl, "UV Limit":dbl}, "update chart?"=w1602:bool)  [unwired: 9 in]
                        n873 = case shown="True" w1602 {
                          tunnel: w1603 -> [_ w1608]
                          frame False {
                          }
                          frame True {
                            n874 = global read "globals-engine.vi" "IRR Params"() -> (w1604:T31)
                            n875 = Unbundle By Name(w1608) -> ("sample"=→"UV Acc.":dbl)
                            n876 = Unbundle By Name(w1604) -> ("Last Iteration"=w1605:timestamp, "UV Reduction Status"=w1606:bool)
                            n877 = property on="UV Reduction Status" class="Bool (strict)"("Value"=w1606) -> ()  [unwired: 2 in, 2 out]
                            n878 = property on="Last Iteration" class="AbsTime (strict)"("Value"=w1605) -> ()  [unwired: 2 in, 2 out]
                            "Waveform Chart 2" <- w1608
                          }
                        }
                      }
                      frame "NTR" {
                        n879 = stacked-sequence {
                          tunnel: w1609 -> [w1611 w1617]
                          frame #0 {
                            n880 = property on="NTR Flowchart" class="Clust (strict)"() -> ("Controls[]"=w1610:refnum<vi>[])  [unwired: 2 in, 2 out]
                            n881 = call "ntr.flow-panel.update.vi"("log cluster"=w1611, "Controls[]"=w1610) -> ()  [unwired: 10 in]
                            n882 = call "helper-log-parse-ntr.vi"("output cluster"=w1611) -> ("NTR Status"=w1613:string, "update?"=w1612:bool)  [unwired: 9 in]
                            n883 = case shown="True" w1612 {
                              tunnel: w1613 -> [_ w1614]
                              frame False {
                              }
                              frame True {
                                "NTR Status" <- w1614
                              }
                            }
                          }
                          frame #1 {
                            n884 = Unbundle By Name(w1617) -> ("Step Function"=w1616:T6)
                            n885 = control-ref of="ntr.status-table"() -> (w1615:refnum<vi>)
                            n886 = case shown="\"UNIT_SAMPLE\"" w1616 {
                              tunnel: w1615 -> [_ w1620]
                              tunnel: w1617 -> [_ w1619]
                              frame Default {
                              }
                              frame "UNIT_SAMPLE" {
                                n887 = call "ntr.log-parse.unit-sample.vi"("log"=w1619, "status-table-REF"=w1620) -> ("ntr.status-table"=→"ntr.status-table":string[][])  [unwired: 9 in]
                              }
                            }
                          }
                        }
                      }
                    }
                  }
                }
                n888 = Merge Errors(w1551, w1549, w1548) -> (w1556:errorcluster)
              }
              frame "LOG.EXIT" {
                # "\"ENG.EXIT\""
                n889 = Release Queue(queue=w1623) -> (error out=w1622:errorcluster)  [unwired: 2 in, 2 out]
                n890 = Merge Errors(w1622) -> (w1621:errorcluster)
              }
              frame "LOG.INIT" {
                # "\"LOG.INIT\"\nSET GUI INDICATORS TO INITIAL STATE"
                n891 = invoke on="MenuRuntime" class="Clust (strict)" method="Reinit To Default"() -> ()  [unwired: 3 in, 3 out]
                n892 = property on="Waveform Chart" class="WFChart (strict)"("History Data"=u32[] []) -> ()  [unwired: 2 in, 2 out]
                n893 = property on="NTR Flowchart" class="Clust (strict)"() -> ("Controls[]"=w1627:refnum<vi>[])  [unwired: 2 in, 2 out]
                n894 = call "ntr.flow-panel.init.vi"("Controls in"=w1627) -> ()  [unwired: 8 in, 3 out]
                n895 = local write "NTR Status"("Initial" ("NTR Status")) -> ()
              }
              frame "LOG.INIT.NTR-FLOW" {
                n896 = property on="NTR Flowchart" class="Clust (strict)"() -> ("Controls[]"=w1630:refnum<vi>[])  [unwired: 2 in, 2 out]
                n897 = local write "NTR Status"("Initial" ("NTR Status")) -> ()
                n898 = call "ntr.flow-panel.init.vi"("Controls in"=w1630) -> ("error in (no error)"=w1628:errorcluster)  [unwired: 8 in, 2 out]
              }
              frame "LOG.NO_OP", Default {
              }
              frame "LOG.PARSE.OCS" {
                # "\"LOG.PARSE.OCS\" \nPARSE Outdoor Climate Sampling module LOG"
                n899 = Variant To Data(type=T86 {"Proc Name"="", "ProcPath"="", "Step Name"="", "Step Function"=enum."__NO-OP", "Step Index"=0, "Report"="", "clk"=0.0, "error in"={"status"=FALSE, "code"=0, "source"=""}, "Log Message"="", "Proc Module"=""} ("output cluster"), Variant=w1638) -> (data=w1636:T86)  [unwired: 1 in, 1 out]
                n900 = Unbundle By Name(w1636) -> ("Proc Name"=w1632:string, "Step Function"=w1635:T6, "Report"=w1634:string)
                n901 = Search and Replace String(input string=w1632, search string="OCS\\") -> (result string=w1631:string)  [unwired: 6 in, 3 out]
                n902 = case "Switch(Proc Name)" shown="\"OCS\"" w1631 {
                  tunnel: w1635 -> [_ w1640 w1646 w1653 w1661 w1703]
                  tunnel: w1634 -> [_ w1639 w1645 w1652 w1660 w1702]
                  frame Default {
                  }
                  frame "GET-UV" {
                    n903 = case shown="\"_IO_READ\"" w1640 {
                      tunnel: w1639 -> [w1643 _]
                      frame "_IO_READ" {
                        n904 = Match Pattern(string=w1643, regular expression="=") -> (after substring=w1641:string)  [unwired: 1 in, 3 out]
                        n905 = Fract/Exp String To Number(string=w1641) -> ()  [unwired: 3 in, 2 out]
                      }
                      frame Default {
                      }
                    }
                  }
                  frame "GET-WD" {
                    n906 = call "util.DelimitedStringToArray.vi"("delimitaed string"=w1645) -> ("array out"=w1644:string[])  [unwired: 10 in]
                    n907 = case shown="\"_GET_WD\"" w1646 {
                      tunnel: w1645 -> [w1649 _]
                      tunnel: w1644 -> [_ _]
                      frame "_GET_WD" {
                        n908 = call "util.DelimitedStringToArray.vi"("delimitaed string"=w1649) -> ("array out"=w1648:string[])  [unwired: 10 in]
                        n909 = Index Array(array=w1648) -> (element=w1647:string)  [unwired: 1 in]
                        n910 = Match Pattern(string=w1647, regular expression="=") -> ()  [unwired: 1 in, 4 out]
                      }
                      frame Default {
                      }
                    }
                  }
                  frame "GET-WS" {
                    n911 = call "util.DelimitedStringToArray.vi"("delimitaed string"=w1652) -> ("array out"=w1651:string[])  [unwired: 10 in]
                    n912 = case shown="\"_GET_WS\"" w1653 {
                      tunnel: w1652 -> [w1657 _]
                      tunnel: w1651 -> [_ _]
                      frame "_GET_WS" {
                        n913 = call "util.DelimitedStringToArray.vi"("delimitaed string"=w1657) -> ("array out"=w1656:string[])  [unwired: 10 in]
                        n914 = Index Array(array=w1656) -> (element=w1655:string)  [unwired: 1 in]
                        n915 = Match Pattern(string=w1655, regular expression="=") -> (after substring=w1654:string)  [unwired: 1 in, 3 out]
                        n916 = Fract/Exp String To Number(string=w1654) -> ()  [unwired: 3 in, 2 out]
                      }
                      frame Default {
                      }
                    }
                  }
                  frame "OCS" {
                    n917 = call "util.DelimitedStringToArray.vi"("delimitaed string"=w1660) -> ("array out"=w1659:string[])  [unwired: 10 in]
                    n918 = case "Switch (Step Name)" shown="\"_OCS_CHECK\"" w1661 {
                      tunnel: w1660 -> [_ _]
                      tunnel: w1659 -> [w1662 _]
                      frame "_OCS_CHECK" {
                        n919 = stacked-sequence {
                          tunnel: w1662 -> [w1663 w1687]
                          frame #0 {
                            # "parse outdoor sensors (TDRY, TWET ...)"
                            n920 = for {
                              tunnel: w1663 -> [w1675] mode=indexing
                              n921 = Match Pattern(string=w1675, regular expression="=") -> (before substring=w1670:string, after substring=w1672:string)  [unwired: 1 in, 2 out]
                              n922 = Concatenate Strings(w1670, "_BUF" ("string")) -> (w1665:string)
                              n923 = Decimal String To Number(string=w1672) -> (number=w1673:i32)  [unwired: 2 in, 1 out]
                              n924 = call "variantCtrlIo.vi"("menu (Get Param)"=enumVarCtrlIO."IO Get By Key", "Key (use IOnode Label if empty )"=w1665) -> ("error out"=w1666:errorcluster, "IOnode out"=w1667:T42)  [unwired: 5 in, 3 out]
                              n925 = Number To Decimal String(number=w1673) -> (decimal integer string=w1671:string)  [unwired: 1 in]
                              n926 = call <vilib>:"Clear Errors.vi"("error in (no error)"=w1666) -> ()  [unwired: 5 in, 2 out]
                              n927 = Unbundle By Name(w1667) -> ("Value"=w1664:string)
                              n928 = case shown="\"H0_WSPD\"" w1670 {
                                tunnel: w1675 -> [_ _ _ _ _ _ _]
                                tunnel: w1671 -> [_ w1676 w1677 w1678 w1679 w1680 w1681]
                                tunnel: w1664 -> [_ _ _ _ _ _ _]
                                frame Default {
                                }
                                frame "H0_TDRY" {
                                n929 = property on="Tdry" class="Str"("Value"=w1676) -> ()  [unwired: 2 in, 2 out]
                                }
                                frame "H0_TWET" {
                                n930 = property on="Twet" class="Str"("Value"=w1677) -> ()  [unwired: 2 in, 2 out]
                                }
                                frame "_H0_RH" {
                                n931 = property on="Humidity" class="Str"("Value"=w1678) -> ()  [unwired: 2 in, 2 out]
                                }
                                frame "H0_UV" {
                                n932 = property on="UV" class="Str"("Value"=w1679) -> ()  [unwired: 2 in, 2 out]
                                }
                                frame "H0_WSPD" {
                                n933 = property on="Wind Speed" class="Str"("Value"=w1680) -> ()  [unwired: 2 in, 2 out]
                                n934 = property on="Wind Speed" class="Str"("Value"=w1680) -> ()  [unwired: 2 in, 2 out]
                                }
                                frame "H0_WDIR" {
                                n935 = Decimal String To Number(string=w1681) -> (number=w1685:i32)  [unwired: 2 in, 1 out]
                                n936 = call "wind-dir-calc.vi"("Analog Direction"=w1685) -> ("Ndir"=w1682:T88, "Wind Dir View"=→"Wind Dir Panel":T29)  [unwired: 9 in]
                                n937 = call "helper-wind-status.vi"("Ndir"=w1682) -> ("Value"=w1683:string)  [unwired: 10 in]
                                n938 = property on="Wind Direction" class="Str"("Value"=w1681) -> ()  [unwired: 2 in, 2 out]
                                n939 = property on="Wind Direction" class="Str"("Value"=w1683) -> ()  [unwired: 2 in, 2 out]
                                }
                              }
                            }
                          }
                          frame #1 {
                            # "parse indoor sensors (H1_TDRY, H1_TWET ...)"
                            n940 = local read "Section"() -> (w1686:string)
                            n941 = for {
                              tunnel: w1687 -> [w1694] mode=indexing
                              tunnel: w1686 -> [w1697]
                              n942 = Format Into String(format string="%s_" ("_H1_"), w1697) -> (resulting string=w1692:string)  [unwired: 2 in, 1 out]
                              n943 = Match Pattern(string=w1694, regular expression="=") -> (before substring=w1693:string, after substring=w1689:string)  [unwired: 1 in, 2 out]
                              n944 = Match Pattern(string=w1693, regular expression=w1692) -> (after substring=w1691:string)  [unwired: 1 in, 3 out]
                              n945 = Decimal String To Number(string=w1689) -> (number=w1690:i32)  [unwired: 2 in, 1 out]
                              n946 = Number To Decimal String(number=w1690) -> (decimal integer string=w1688:string)  [unwired: 1 in]
                              n947 = case shown="\"TDRY\"" w1691 {
                                tunnel: w1688 -> [_ w1698 w1699 w1700]
                                frame Default {
                                }
                                frame "TDRY" {
                                n948 = property on="Tdry" class="Str"("Value"=w1698) -> ()  [unwired: 2 in, 2 out]
                                }
                                frame "TWET" {
                                n949 = property on="Twet" class="Str"("Value"=w1699) -> ()  [unwired: 2 in, 2 out]
                                }
                                frame "RH" {
                                n950 = property on="Humidity" class="Str"("Value"=w1700) -> ()  [unwired: 2 in, 2 out]
                                }
                              }
                            }
                          }
                        }
                      }
                      frame Default {
                      }
                    }
                  }
                  frame "OCS_RECORD" {
                    n951 = call "util.DelimitedStringToArray.vi"("delimitaed string"=w1702) -> ("array out"=w1701:string[])  [unwired: 10 in]
                    n952 = case "Switch (Step Name)" shown="\"_OCS_RECORD\"" w1703 {
                      tunnel: w1702 -> [_ _]
                      tunnel: w1701 -> [_ _]
                      frame Default {
                      }
                      frame "_OCS_RECORD" {
                        n953 = property on="refresh" class="Bool (strict)"("Val(Sgnl)"=TRUE ("Value (Signaling)")) -> ()  [unwired: 2 in, 2 out]
                      }
                    }
                  }
                }
              }
              frame "LOG.SNAPSHOT" {
                # "\"LOG.UPDATE.SNAPSHOT\" (Snapshot)"
                n954 = local read "Tab Main"() -> (w1707:enum32{"MAIN", "I/O", "ADMIN"})
                n955 = local read "Tab IO"() -> (w1706:enum32{"Map", "Editor", "Calibration"})
                n956 = call "util-ui-view.vi"("Page2"=w1706, "Page1"=w1707) -> ("Page1:Page2"=w1705:string)  [unwired: 7 in, 2 out]
                n957 = case shown="\"I/O:Map\"" w1705 {
                  tunnel: w1709 -> [_ w1722]
                  tunnel: [_ w1721] -> w1708
                  frame "False", Default {
                  }
                  frame "I/O:Map" {
                    n958 = Variant To Data(type=T13[] [{"Address"=0, "DI"=[], "status"={"status"=TRUE, "code"=-1073807339, "source"="Failed to read IO: "}, "AI"=[0.0], "Dports"=0, "AI RAW"=[]}, {"Address"=1, "DI"=[], "status"={"status"=TRUE, "code"=-1073807339, "source"="Failed to read IO: "}, "AI"=[0.0], "Dports"=0, "AI RAW"=[]}, {"Address"=2, "DI"=[FALSE, FALSE, FALSE, FALSE, FALSE, FALSE, FALSE, TRUE, FALSE, FALSE, FALSE, FALSE, FALSE, FALSE, FALSE, FALSE, FALSE, FALSE, TRUE, FALSE, FALSE, FALSE, FALSE, FALSE, FALSE, TRUE, FALSE, FALSE, FALSE, FALSE, FALSE, FALSE, TRUE, TRUE, TRUE, TRUE, TRUE, TRUE, FALSE, TRUE], "status"={"status"=FALSE, "code"=0, "source"=""}, "AI"=[-39.53601953601954, 0.0, 0.0, 0.0, 0.0, -8.815628815628816], "Dports"=0, "AI RAW"=[]}, {"Address"=3, "DI"=[], "status"={"status"=TRUE, "code"=-1073807339, "source"="Failed to read IO: "}, "AI"=[0.0], "Dports"=0, "AI RAW"=[]}, {"Address"=4, "DI"=[], "status"={"status"=TRUE, "code"=-1073807339, "source"="Failed to read IO: "}, "AI"=[0.0], "Dports"=0, "AI RAW"=[]}, {"Address"=5, "DI"=[], "status"={"status"=TRUE, "code"=-1073807339, "source"="Failed to read IO: "}, "AI"=[0.0], "Dports"=0, "AI RAW"=[]}] ("Dout List"), Variant=w1722) -> (data=w1719:T13[], error out=w1721:errorcluster)  [unwired: 1 in]
                    n959 = local read "IO Map DO"() -> (w1718:T37[])
                    n960 = local read "IO Map AI"() -> (w1717:T39[])
                    n961 = local read "IO Map DI"() -> (w1715:T40[])
                    n962 = call "helper-snapshot-update.vi"("Snapshot"=w1719, "IO Map DI in"=w1715, "IO Map AI in"=w1717, "IO Map DO in"=w1718) -> ("IO Map DI out"=w1716:T40[], "IO Map AI out"=w1724:T39[], "IO Map DO out"=w1723:T37[], "AI RAW"=w1712:dbl[][], "AI"=w1713:dbl[][])  [unwired: 3 in]
                    n963 = property on="State" class="Bool (strict)"("DisabledEnum"=T72."Enabled" ("Disabled")) -> ()  [unwired: 2 in, 2 out]
                    n964 = local write "IO Map DO"(w1723) -> ()
                    n965 = local write "IO Map DI"(w1716) -> ()
                    n966 = local write "IO Map AI"(w1724) -> ()
                    n967 = Select(t=w1713, s="Calib?", f=w1712) -> (s? t:f=→"AI":dbl[][])
                  }
                }
              }
              frame "LOG.SNAPSHOT.PROC" {
                # "\"LOG.UPDATE.STATUS\" (PROCS) - \nget ENG STATS of procs and IO conf"
                n968 = disable-structure shown="Enabled" {
                  disable-tunnel: w1726 -> [w1733 w1746]
                  disable-tunnel: [_ w1745] -> w1725
                  frame Disabled {
                    w1732 = cluster{"Procedure":variant[]}[] []  # Clustered Proces
                    # "\"LOG.UPDATE.STATUS\" (PROCS)\nUPDATE RUNTIME LIST AND CLEAR LOG BUFFERS (MUST BE CALLED FROM ENG)"
                    n969 = Variant To Data(type=w1732, Variant=w1733) -> (data=w1730:cluster{"Procedure":variant[]}[])  [unwired: 1 in, 1 out]
                    n970 = for {
                      tunnel: w1730 -> [w1739] mode=indexing
                      tunnel: [w1734] -> _ mode=indexing
                      n971 = Unbundle(w1739) -> ("Procedure"=w1736:variant[])
                      n972 = Index Array(array=w1736) -> (element=w1735:variant)  [unwired: 1 in]
                      n973 = call "proc.util.enumToStrProcVar.vi"("Proc var"=typeProcVarientName."procNameID" ("proc var")) -> ("String"=w1738:string)  [unwired: 10 in]
                      n974 = call-poly "variantCtrl.polymorphic.vi"("name in"=w1738, "Step in"=w1735) -> ("String Value"=w1734:string)  [unwired: 6 in, 3 out]
                    }
                    n975 = call "reg-log-ntr.vi"("Operation(Read)"=enum.report-filter."ClearAll" ("Operation(Collect)")) -> ("compact report"=w1727:T78[])  [unwired: 8 in, 2 out]
                    n976 = call "reg-log-irr.vi"("Operation(Read)"=enum.report-filter."ClearAll") -> ("compact report"=w1728:T78[])  [unwired: 8 in, 2 out]
                    n977 = local write item#-1(w1727) -> ()
                    n978 = local write item#-1(w1728) -> ()
                    n979 = local write item#-1(w1728) -> ()
                  }
                  frame Enabled {
                    w1747 = cluster{"Procedure":variant[]}[] []  # Clustered Proces
                    n980 = Variant To Data(type=w1747, Variant=w1746) -> (data=w1744:cluster{"Procedure":variant[]}[], error out=w1745:errorcluster)  [unwired: 1 in]
                    n981 = local read "Proc Select 2"() -> (w1740:string)
                    n982 = call "util.procs.find-by-name.vi"("ProcName in"=w1740, "Procs in"=w1744) -> ("Found Proc"=w1743:cluster{"Procedure":variant[]})  [unwired: 4 in, 5 out]
                    n983 = Unbundle By Name(w1743) -> ("Procedure"=w1742:variant[])
                    n984 = call "build.proc.parse.vi"("Array in"=w1742) -> ("Flow Steps"=→"UiBuildSteps 2":T49[])  [unwired: 8 in, 2 out]
                  }
                }
              }
              frame "LOG.UPDATE.IRR" {
                n985 = control-ref of="Solar Elevation Graph"() -> (w1762:refnum<vi>)
                n986 = global read "globals-engine.vi" "IRR Params"() -> (w1752:T31)
                n987 = call "nrs.sunrise-time-table.vi"() -> ("Irrigation Timing"=w1756:T89, "Sunrise Timing"=w1761:cluster{"Sunset":timestamp, "Sunrise":timestamp}, "Solar Elevation Graph"=→"Solar Elevation Graph":waveform(dbl))  [unwired: 9 in]
                n988 = Unbundle By Name(w1752) -> ("timeLimits.Irrigation"=w1751:dbl, "timeLimits.Nut./Water"=w1750:dbl)
                n989 = property on="Day Time" class="Clust (strict)"("Value"=w1761) -> ()  [unwired: 2 in, 2 out]
                n990 = property on="Calculated Timing" class="Clust (strict)"("Value"=w1756) -> ()  [unwired: 2 in, 2 out]
                n991 = Unbundle By Name(w1756) -> ("Irrigation Timeout"=w1754:timestamp, "Fertiliztion Timeout"=w1755:timestamp)
                n992 = Unbundle By Name(w1761) -> ("Sunset"=w1760:timestamp, "Sunrise"=w1758:timestamp)
                n993 = Absolute Value(x=w1751) -> (abs(x)=w1749:dbl)
                n994 = Absolute Value(x=w1750) -> (abs(x)=w1748:dbl)
                n995 = To Double Precision Float(number=w1760) -> (double precision float=w1759:dbl)
                n996 = To Double Precision Float(number=w1758) -> (double precision float=w1757:dbl)
                n997 = To Double Precision Float(number=w1755) -> ()  [unwired: 1 out]
                n998 = To Double Precision Float(number=w1754) -> ()  [unwired: 1 out]
                n999 = call "Add Cursors To Graph.vi"("Sunset Time"=w1759, "Sunrise Time"=w1757, "Solar Elevation Graph Ref"=w1762, "Postpone Time"=w1749, "Fresh Water Time"=w1748) -> ("error out"=w1753:errorcluster)  [unwired: 10 in]
              }
              frame "LOG.UPDATE.SELECTORS" {
                # "\"LOG.UPDATE.STATUS\" (PROCS) - \nget ENG STATS of procs and IO conf"
                n1000 = disable-structure shown="Enabled" {
                  frame Disabled {
                    w1770 = cluster{"Procedure":variant[]}[] []  # Clustered Proces
                    # "\"LOG.UPDATE.STATUS\" (PROCS)\nUPDATE RUNTIME LIST AND CLEAR LOG BUFFERS (MUST BE CALLED FROM ENG)"
                    n1001 = Variant To Data(type=w1770) -> (Variant=w1771:cluster{"Procedure":variant[]}[], data=w1768:cluster{"Procedure":variant[]}[])  [unwired: 1 in, 1 out]
                    n1002 = for {
                      tunnel: w1768 -> [w1777] mode=indexing
                      tunnel: [w1772] -> _ mode=indexing
                      n1003 = Unbundle(w1777) -> ("Procedure"=w1774:variant[])
                      n1004 = Index Array(array=w1774) -> (element=w1773:variant)  [unwired: 1 in]
                      n1005 = call "proc.util.enumToStrProcVar.vi"("Proc var"=typeProcVarientName."procNameID" ("proc var")) -> ("String"=w1776:string)  [unwired: 10 in]
                      n1006 = call-poly "variantCtrl.polymorphic.vi"("name in"=w1776, "Step in"=w1773) -> ("String Value"=w1772:string)  [unwired: 6 in, 3 out]
                    }
                    n1007 = call "reg-log-ntr.vi"("Operation(Read)"=enum.report-filter."ClearAll" ("Operation(Collect)")) -> ("compact report"=w1765:T78[])  [unwired: 8 in, 2 out]
                    n1008 = call "reg-log-irr.vi"("Operation(Read)"=enum.report-filter."ClearAll") -> ("compact report"=w1766:T78[])  [unwired: 8 in, 2 out]
                    n1009 = local write item#-1(w1765) -> ()
                    n1010 = local write item#-1(w1766) -> ()
                    n1011 = local write item#-1(w1766) -> ()
                  }
                  frame Enabled {
                    n1012 = call "variantCtrlIo.vi"("menu (Get Param)"=enumVarCtrlIO."IO List Configs") -> ("IO Configs List"=w1778:T42[])  [unwired: 6 in, 4 out]
                    n1013 = stacked-sequence {
                      tunnel: w1778 -> [w1780 w1792 w1808 _]
                      frame #0 {
                        # "list all I/O"
                        n1014 = disable-structure shown="Disabled" {
                          disable-tunnel: w1780 -> [w1783 _]
                          frame Disabled {
                            w1781 = T3[] [enum."AI", enum."DI", enum."DO"] items=["Type", "DI", "DO", "AI", "AO", "VL", "BUF"] ("Array")
                            n1015 = for {
                              tunnel: w1781 -> [w1785] mode=indexing
                              tunnel: w1783 -> [w1789]
                              tunnel: [w1788] -> _ mode=concatenating
                              tunnel: [w1786] -> _ mode=indexing
                              tunnel: enum.io.mode."Mode" ("Mode(Any)") -> [w1784]
                              n1016 = call "io-find-by-type.vi"("Mode(Any)"=w1784, "Type"=w1785, "IOConfigs in"=w1789) -> ("Search Results"=w1788:T42[])  [unwired: 8 in]
                              n1017 = Array Size(array=w1788) -> (size(s)=w1787:i32)
                              n1018 = Bundle("type"=w1785, w1787) -> (w1786:cluster{"type":T3, i32})  [unwired: 1 in]
                            }
                          }
                          frame Enabled {
                          }
                        }
                      }
                      frame #1 {
                        # "update AIN selectors"
                        n1019 = call "io-find-by-type.vi"("Mode(Any)"=enum.io.mode."Mode", "Type"=enum.io.type."AI", "IOConfigs in"=w1792) -> ("Search Results"=w1801:T42[])  [unwired: 8 in]
                        n1020 = call "io-find-by-type.vi"("Mode(Any)"=enum.io.mode."Mode", "Type"=enum.io.type."DI", "IOConfigs in"=w1792) -> ("Search Results"=w1790:T42[])  [unwired: 8 in]
                        n1021 = Build Array (concatenate)(w1801, w1790) -> (w1791:T42[])
                        n1022 = for {
                          tunnel: w1791 -> [w1807] mode=indexing
                          tunnel: [w1804] -> w1800 mode=indexing
                          tunnel: [w1804] -> w1799 mode=indexing if=w1803
                          n1023 = Unbundle By Name(w1807) -> ("Label"=w1804:string, "Mode"=w1806:T38)
                          n1024 = Equal?(x=w1806, y=enum.io.mode."SIM") -> (x = y?=w1803:bool)
                        }
                        "Simulated" <- w1799
                        n1025 = Sort 1D Array(array=w1800) -> (sorted array=w1796:string[])
                        n1026 = Index Array(array=w1796) -> (element=w1797:string)  [unwired: 1 in]
                        n1027 = property on="IO calib select" class="CmbBox"("Strings[]"=w1796, "Value"=w1797) -> ()  [unwired: 2 in, 2 out]
                        n1028 = property on="IO Simulat select" class="CmbBox"("Strings[]"=w1796, "Value"="") -> ()  [unwired: 2 in, 2 out]
                      }
                      frame #2 {
                        w1810 = map{string, u8} {}  # Size: 0
                        # "create map:\n{\n  key: deviceAddressStr\n  Value: deviceAddressNum\n}"
                        # "list hardware addresses from I/O confs"
                        n1029 = for {
                          tunnel: w1808 -> [w1823] mode=indexing
                          tunnel: [w1822] -> w1811 mode=indexing
                          workers-P: _ -> [_]
                          n1030 = Unbundle By Name(w1823) -> ("ADDR"=w1822:T8)  [unwired: 2 out]
                        }
                        n1031 = for {
                          shift-right: [w1820] -> w1812
                          shift-left: w1810 -> [w1821]
                          tunnel: w1811 -> [w1818] mode=indexing
                          n1032 = call "util-address-parser.vi"("ADDR 2"=w1818) -> ("Address"=w1817:u8)  [unwired: 9 in, 1 out]
                          n1033 = Number To Decimal String(number=w1817) -> (decimal integer string=w1819:string)  [unwired: 1 in]
                          n1034 = Insert Into Map(map in=w1821, key=w1819, value=w1817) -> (map out=w1820:map{string, u8})  [unwired: 2 out]
                        }
                        n1035 = for {
                          tunnel: w1812 -> [w1816] mode=indexing
                          tunnel: [w1813] -> w1809 mode=indexing
                          workers-P: _ -> [_]
                          # "list map values"
                          n1036 = Unbundle By Name(w1816) -> ("Address"=w1814:u8)
                          n1037 = Bundle("Address"=w1814, "status"=TRUE) -> (w1813:cluster{"Address":u8, "status":bool})  [unwired: 1 in]
                        }
                        "RIO List" <- w1809
                      }
                      frame #3 {
                        # "list ICC folder for proc filenames and update section selector"
                        n1038 = call "util-path.vi"("append path (ie. folder\\filename.*)"="ICC" ("dir name")) -> ("error out"=w1826:errorcluster, "SelectedPath"=w1827:path)  [unwired: 6 in, 3 out]
                        n1039 = List Folder(path=w1827, error in=w1826) -> (folder names=w1829:string[], error out=w1825:errorcluster)  [unwired: 2 in, 2 out]
                        n1040 = Index Array(array=w1829) -> (element=w1828:string)  [unwired: 1 in]
                        n1041 = property on="Section" class="CmbBox"(error in=w1825, "Strings[]"=w1829, "Value"=w1828) -> (error out=w1824:errorcluster)  [unwired: 1 in, 1 out]
                        n1042 = case shown="No Error" w1824 {
                          frame No Error {
                          }
                          frame Error {
                          }
                        }
                      }
                    }
                  }
                }
              }
            }
            n1043 = call "helper-log-log.vi"("error in"=w1540, "Enum"=w1538) -> ("Collected Reports"=→"Collected Reports 2":string)  [unwired: 8 in, 1 out]
          }
        }
      }
      frame Error {
        # "handle error by displaying a continue/stop message dialog."
      }
    }
    n1044 = case shown="Default" w1518 {
      selector: w1518 -> [_ w1529]
      frame "" {
        # "skip empty statuts"
      }
      frame Default {
        # "status register"
        n1045 = call "reg-status.vi"("Operation(Read)"=enum.report-filter."Collect", "Reports to Collect"=w1529) -> ("Collected Reports"=w1528:string)  [unwired: 8 in, 1 out]
        n1046 = local write "User messages"(w1528) -> ()
      }
    }
    n1047 = call "util-collect-error.vi"("error in (no error)"=w1513, "Array in"=w1515) -> ("Array out"=w1514:errorcluster[])  [unwired: 9 in]
    "GUI Engine Errors" <- w1514
    "GuiLog" <- w1516
  }
  n1048 = while "LOCAL MEASUREMENT RECORD" {
    tunnel: w18 -> [w1839]
    tunnel: w17 -> [w1840]
    shift-right: [w1836] -> _
    shift-left: _ -> [w1835]
    shift-right: [w1834] -> _
    shift-left: errorcluster[] [] ("Array out") -> [w1833]
    i -> [w1837]
    stop <- w1844 stop-if-true
    n1049 = Get Date/Time In Seconds() -> (seconds since 1Jan1904=w1838:timestamp)
    n1050 = Dequeue Element(queue=w1839, timeout in ms (-1)=250, error in (no error)=w1840) -> (queue out=w1843:refnum<queue>, element=w1845:cluster{"data":variant, "Enum":T55}, timed out?=w1842:bool, error out=w1846:errorcluster)
    n1051 = case shown="No Error" w1846 {
      selector: w1846 -> [_ w1950]
      tunnel: w1845 -> [w1852 _]
      tunnel: [w1849 _] -> w1844
      tunnel: w1843 -> [w1853 _]
      tunnel: w1842 -> [w1851 _]
      tunnel: [w1850 w1950] -> w1832
      tunnel: w1838 -> [_ _]
      tunnel: [w1848 w1949] -> w1836
      tunnel: w1835 -> [w1847 w1949]
      frame No Error {
        n1052 = case shown="False" w1851 {
          tunnel: w1853 -> [_ w1878]
          tunnel: w1852 -> [_ w1876]
          tunnel: [w1855 w1874] -> w1850
          tunnel: [_ w1877] -> w1849
          tunnel: [w1859 w1871] -> w1848
          tunnel: w1847 -> [w1859 w1870]
          frame True {
            # "Queue Timeout"
            n1053 = call "step.util.flag-matching.vi"("include step flags"=FALSE, "$string in"="serial\\serial-$date.*" ("append path (ie. folder\\filename.*)")) -> ("formated string out"=w1864:string)  [unwired: 9 in]
            n1054 = Refnum to Path(1:w1859) -> (0:w1858:path)
            n1055 = call "util-path.vi"("Create Folders?(F)"=TRUE, "Selected Folder (PROCS)"=typePathSelector."DIR_LOG" ("Selected Folder (PROCEDURE_DIR)"), "append path (ie. folder\\filename.*)"=w1864) -> ("error out"=w1854:errorcluster, "SelectedPath"=w1857:path)  [unwired: 4 in, 3 out]
            n1056 = Not Equal?(x=w1858, y=w1857) -> (x != y?=w1856:bool)
            n1057 = case shown="False" w1856 {
              tunnel: [w1865 w1867] -> w1855
              tunnel: w1854 -> [w1865 w1866]
              frame False {
              }
              frame True {
                n1058 = global read "globals-engine.vi" "Q-Com"() -> (w1868:refnum<queue>)
                n1059 = Enqueue Element At Opposite End(queue=w1868, element=cluster{"data":variant, "Enum":T55} {"data"=variant, "Enum"=enum."REC.REOPEN-FILE"} ("procQ"), error in (no error)=w1866) -> (error out=w1867:errorcluster)  [unwired: 1 in, 2 out]
              }
            }
          }
          frame False {
            # "Command Handler"
            n1060 = Unbundle(w1876) -> ("data"=w1875:variant, "Enum"=w1873:T55)
            n1061 = case shown="\"REC.OPEN-FILE\"" w1873 {
              tunnel: w1878 -> [w1883 _ _ w1890 w1908 _ _ w1948]
              tunnel: [w1881 _ _ w1889 w1907 w1923 w1933 w1946] -> w1874
              tunnel: [TRUE _ _ _ _ _ _ _] -> w1877
              tunnel: w1875 -> [_ _ _ w1893 w1911 _ _ _]
              tunnel: T53 {"Caller"="", "IOnode"={"ADDR"=0, "Label"="Name", "Type"=enum."DI", "Mode"=enum."RIO", "Value"="Value", "Tags"="Tags", "calibration"=[]}, "error"={"status"=FALSE, "code"=0, "source"=""}, "dports"=[], "AIN (calib)"=0.0, "AIN (raw)"=0, "Times Stamp"=timestamp(0 s since 1904-01-01), "Record File Path"=path "", "Visa Data"=""} ("input cluster") -> [_ _ _ w1888 w1906 _ w1935 _]
              tunnel: [w1879 w1885 w1886 w1887 w1905 w1931 w1934 w1945] -> w1871
              tunnel: w1870 -> [w1879 w1885 w1886 w1887 w1905 w1931 _ w1945]
              frame "REC.EXIT" {
                n1062 = Close File(refnum=w1879) -> (error out=w1880:errorcluster)  [unwired: 1 in, 1 out]
                n1063 = Release Queue(queue=w1883) -> (error out=w1882:errorcluster)  [unwired: 2 in, 2 out]
                n1064 = Merge Errors(w1882, w1880) -> (w1881:errorcluster)
              }
              frame "REC.INIT" {
              }
              frame "REC.NO_OP", Default {
              }
              frame "REC.SERIAL" {
                # "\"REC.SERIAL\" \nLOGS SERIAL PORT COMMUNICATION"
                n1065 = Variant To Data(type=w1888, Variant=w1893) -> (data=w1891:T53, error out=w1892:errorcluster)  [unwired: 1 in]
                n1066 = stacked-sequence {
                  tunnel: w1892 -> [w1900]
                  tunnel: w1891 -> [w1896]
                  tunnel: w1890 -> [_]
                  tunnel: [w1895] -> w1889
                  tunnel: w1887 -> [w1901]
                  frame #0 {
                    n1067 = disable-structure shown="Enabled" {
                      disable-tunnel: w1896 -> [w1902 _]
                      frame Disabled {
                        n1068 = call "helper-serial-log-to-string.vi"("input cluster"=w1902) -> ("String"=w1904:string)  [unwired: 8 in, 2 out]
                        n1069 = call "reg-visa.vi"("Operation(Read)"=enum.report-filter."Collect", "Reports to Collect"=w1904) -> ()  [unwired: 8 in, 2 out]
                      }
                      frame Enabled {
                      }
                    }
                    n1070 = Write Datalog(4:w1900, 6:w1896, 7:w1901) -> (0:w1898:errorcluster, 3:w1899:refnum<k1>)
                    n1071 = Get Number of Records(4:w1898, 7:w1899) -> (0:w1894:errorcluster, 2:→"COM Size":i64)  [unwired: 1 out]
                    n1072 = Merge Errors(w1894) -> (w1895:errorcluster)
                  }
                }
              }
              frame "REC.IO" {
                # "\"REC.IO\" \nRECORD I/O MEASURMENT FILES."
                n1073 = Variant To Data(type=w1906, Variant=w1911) -> (data=w1909:T53, error out=w1910:errorcluster)  [unwired: 1 in]
                n1074 = stacked-sequence {
                  tunnel: w1910 -> [_]
                  tunnel: w1909 -> [w1914]
                  tunnel: w1908 -> [_]
                  tunnel: [w1912] -> w1907
                  tunnel: w1905 -> [_]
                  frame #0 {
                    n1075 = call "helper-eng-rec.vi"("input cluster"=w1914) -> ("error"=w1913:errorcluster)  [unwired: 10 in]
                    n1076 = Merge Errors(w1913) -> (w1912:errorcluster)
                  }
                }
              }
              frame "REC.FETCH" {
                n1077 = local read "COM Size"() -> (w1920:i64)
                n1078 = In Range and Coerce(upper limit=w1920, x="Snapshot Size", lower limit=i64 0) -> (coerced(x)=w1918:i64)  [unwired: 1 out]
                n1079 = Negate(x=w1918) -> (-x=w1922:i64)
                n1080 = Set Datalog Position(5:enum16{"start", "end", "current"}."end" ("from (0:start)"), 6:w1922, 7:w1931) -> (0:w1930:errorcluster, 3:w1928:refnum<k1>)  [unwired: 1 in]
                n1081 = Read Datalog(4:w1930, 6:w1918, 7:w1928) -> (0:w1924:errorcluster, 2:w1915:T53[], 3:w1926:refnum<k1>)
                "Serial Record(s)" <- w1915
                n1082 = call "helper-serial-log-to-string-2.vi"("Array in"=w1915) -> ("Array out"=w1916:T51[])  [unwired: 10 in]
                n1083 = call <vilib>:"Clear Errors.vi"("error in (no error)"=w1924) -> ("error out"=w1921:errorcluster)  [unwired: 5 in, 1 out]
                n1084 = local write "COM Snapshot"(w1916) -> ()
                n1085 = Set Datalog Position(4:w1921, 5:enum16{"start", "end", "current"}."end" ("from (0:start)"), 6:i64 0 ("offset (in records) (0)"), 7:w1926) -> (0:w1923:errorcluster)  [unwired: 1 out]
              }
              frame "REC.OPEN-FILE" {
                n1086 = call "step.util.flag-matching.vi"("include step flags"=FALSE, "$string in"="serial\\serial-$date.*" ("append path (ie. folder\\filename.*)")) -> ("formated string out"=w1943:string)  [unwired: 9 in]
                n1087 = call "util-path.vi"("Create Folders?(F)"=TRUE, "Selected Folder (PROCS)"=typePathSelector."DIR_LOG" ("Selected Folder (PROCEDURE_DIR)"), "append path (ie. folder\\filename.*)"=w1943) -> ("error out"=w1932:errorcluster, "SelectedPath"=w1937:path)  [unwired: 4 in, 3 out]
                n1088 = Open/Create/Replace Datalog(5:w1935, 8:w1932, 10:T90."open or create" ("operation (0:open)"), 11:w1937) -> (0:w1933:errorcluster, 3:w1934:refnum<k1>)  [unwired: 2 in, 1 out]
                n1089 = Refnum to Path(1:w1934) -> (0:→"SelectedPath":path)
              }
              frame "REC.REOPEN-FILE" {
                n1090 = Close File(refnum=w1945) -> (error out=w1944:errorcluster)  [unwired: 1 in, 1 out]
                n1091 = Enqueue Element At Opposite End(queue=w1948, element=cluster{"data":variant, "Enum":T55} {"data"=variant, "Enum"=enum."REC.OPEN-FILE"} ("procQ"), error in (no error)=w1944) -> (error out=w1946:errorcluster)  [unwired: 1 in, 2 out]
              }
            }
          }
        }
      }
      frame Error {
        # "handle error by displaying a continue/stop message dialog."
      }
    }
    n1092 = call "util-collect-error.vi"("error in (no error)"=w1832, "Array in"=w1833) -> ("Array out"=w1834:errorcluster[])  [unwired: 9 in]
    "Record Engine Errors" <- w1834
    "ComLog" <- w1837
  }
  n1093 = while "EXECUTION CONTROL" {
    tunnel: w28 -> [w1952]
    shift-right: [w1961] -> _
    shift-left: cluster{"Procedure":variant[]}[] [] ("Array 5") -> [w1964]
    shift-right: [w1953] -> w36
    shift-left: errorcluster[] [] ("Array out") -> [w1955]
    i -> [w1962]
    stop <- w1966 stop-if-true
    n1094 = disable-structure shown="Enabled" {
      disable-tunnel: w1952 -> [w1971 _]
      frame Disabled {
        n1095 = Get Queue Status(queue=w1971, return elements? (F)=TRUE) -> (elements=→"elements":cluster{"case":T5, "data":variant}[])  [unwired: 1 in, 7 out]
      }
      frame Enabled {
      }
    }
    n1096 = Dequeue Element(queue=w1952, timeout in ms (-1)="ENG ms") -> (queue out=w1965:refnum<queue>, element=w1967:cluster{"case":T5, "data":variant}, timed out?=w1963:bool, error out=w1968:errorcluster)  [unwired: 1 in]
    n1097 = case shown="No Error" w1968 {
      selector: w1968 -> [_ w2835]
      tunnel: w1967 -> [w1989 _]
      tunnel: [w1984 _] -> w1966
      tunnel: w1965 -> [w1990 _]
      tunnel: w1964 -> [w1988 w2837]
      tunnel: [w1987 w2837] -> w1961
      tunnel: w1963 -> [w1986 _]
      tunnel: [w1985 w2836] -> w1954
      tunnel: [w1977 _] -> w1956
      tunnel: [w1983 w2834] -> w1960
      tunnel: "Time Addition" -> [w1982 _]
      tunnel: "Clk Simulator" -> [w1981 _]
      frame No Error {
        n1098 = call "helper-eng-clock-src.vi"("Clk Simulator"=w1981, "Time Addition"=w1982) -> ("Clk Simulated"=→"Clock Simulation":bool, "CLK"=w1979:dbl)  [unwired: 7 in, 1 out]
        n1099 = Get Date/Time In Seconds() -> (seconds since 1Jan1904=w1978:timestamp)
        n1100 = To Double Precision Float(number=w1978) -> (double precision float=w1977:dbl)
        n1101 = case shown="False" w1986 {
          tunnel: w1990 -> [w1996 w2052]
          tunnel: w1989 -> [_ w2047]
          tunnel: w1988 -> [w1993 w2050]
          tunnel: [w1991 w2049] -> w1987
          tunnel: [w1995 w2043] -> w1985
          tunnel: [_ w2048] -> w1984
          tunnel: [w1992 w2046] -> w1983
          tunnel: w1979 -> [w1994 w2040]
          tunnel: w1977 -> [_ _]
          frame True {
            # "Queue Timeout  (procedure execution)"
            n1102 = disable-structure shown="Enabled" {
              disable-tunnel: w1996 -> [w1999 _ w2029]
              disable-tunnel: [w1998 w2014 w2017] -> w1995
              disable-tunnel: w1994 -> [_ w2007 w2018]
              disable-tunnel: w1993 -> [_ w2016 w2030]
              disable-tunnel: [_ "Engine execution" "Engine execution"] -> w1992
              disable-tunnel: [_ w2005 _] -> w1991
              frame Disabled {
                n1103 = property on="ProcedureRun" class="Bool (strict)"() -> ("Value"=w1997:bool)  [unwired: 2 in, 2 out]
                n1104 = case shown="True" w1997 {
                  tunnel: w1999 -> [w2001 w2004]
                  tunnel: [w2000 w2003] -> w1998
                  frame False {
                    n1105 = call "eng-call-execute.vi"("Queue in"=w2001) -> ("error out"=w2000:errorcluster)  [unwired: 10 in]
                  }
                  frame True {
                    n1106 = property on="ProcedureSelect" class="CmbBox"() -> ("Value"=w2002:string)  [unwired: 2 in, 2 out]
                    n1107 = call "eng-call-execute.vi"("Proc Name to Execute (empty: Execute All)"=w2002, "Queue in"=w2004) -> ("error out"=w2003:errorcluster)  [unwired: 9 in]
                  }
                }
              }
              frame Enabled {
                w2015 = -1  # execute all
                n1108 = To Time Stamp(1:w2007) -> (0:w2012:timestamp)
                n1109 = Get Date/Time String(seconds (now)=w2012, want seconds? (F)=TRUE) -> (date string=w2010:string, time string=w2011:string)  [unwired: 1 in]
                n1110 = Format Into String(format string="%s %s", w2010, w2011) -> (resulting string=→"clock":string)  [unwired: 2 in, 1 out]
                n1111 = call "engine.executor.vi"("Index(-1: All)"=w2015, "clk (NaN)"=w2007, "Procs in"=w2016) -> ("Error"=w2014:errorcluster, "Procs out"=w2005:cluster{"proc out":variant[]}[])  [unwired: 5 in, 2 out]
              }
              frame Disabled {
                w2028 = -1  # execute all
                n1112 = To Time Stamp(1:w2018) -> (0:w2024:timestamp)
                n1113 = Get Date/Time String(seconds (now)=w2024, want seconds? (F)=TRUE) -> (date string=w2022:string, time string=w2023:string)  [unwired: 1 in]
                n1114 = Format Into String(format string="%s %s", w2022, w2023) -> (resulting string=→"clock 3":string)  [unwired: 2 in, 1 out]
                n1115 = call "engine.executor.vi"("Index(-1: All)"=w2028, "clk (NaN)"=w2018, "Procs in"=w2030) -> ("Error"=w2027:errorcluster, "ErrorProcs out"=w2026:T98)  [unwired: 5 in, 2 out]
                n1116 = stacked-sequence {
                  tunnel: w2029 -> [_ w2036]
                  tunnel: w2027 -> [_ w2031]
                  tunnel: w2026 -> [_ _]
                  tunnel: [_ w2032] -> w2017
                  frame #0 {
                  }
                  frame #1 {
                    n1117 = property on="ProcedureStep" class="Bool (strict)"() -> ("Value"=w2033:bool)  [unwired: 2 in, 2 out]
                    n1118 = property on="Step" class="Bool (strict)"() -> ("Value"=w2035:bool)  [unwired: 2 in, 2 out]
                    n1119 = Or(x=w2035, y=w2033) -> (x .or. y?=w2034:bool)
                    n1120 = case shown="True" w2034 {
                      tunnel: w2036 -> [_ _]
                      tunnel: [_ w2039] -> w2032
                      tunnel: w2031 -> [_ w2037]
                      frame False {
                      }
                      frame True {
                        w2038 = FALSE ("flagEngRunStep")
                        n1121 = property on="Step" class="Bool (strict)"("Value"=w2038) -> ()  [unwired: 2 in, 2 out]
                        n1122 = property on="ProcedureStep" class="Bool (strict)"("Value"=w2038) -> ()  [unwired: 2 in, 2 out]
                        n1123 = call "eng-call-start.vi"("error in (no error)"=w2037, "Start(T)/Stop(F)"=w2038) -> ("error out"=w2039:errorcluster)  [unwired: 9 in]
                      }
                    }
                  }
                }
              }
            }
          }
          frame False {
            # "Command Handler"
            n1124 = Unbundle(w2047) -> ("case"=w2044:T5, "data"=w2051:variant)
            "case" <- w2044
            n1125 = case shown="\"ENG.EXIT\"" w2044 {
              tunnel: w2052 -> [_ _ _ _ _ _ w2169 w2174 _ _ _ _ _ _ _ w2440 _ _ _ _ w2510 _ _ _ _ _ _ _ _ _ _ _ _ _]
              tunnel: w2051 -> [w2064 _ _ _ w2149 _ _ _ _ _ w2355 _ _ w2415 _ w2437 _ w2450 w2460 w2487 w2511 w2553 w2569 w2579 w2586 _ w2632 w2658 _ _ _ _ _ _]
              tunnel: w2050 -> [w2063 w2103 w2110 w2117 w2151 w2155 w2170 w2175 w2193 w2320 w2360 w2387 _ w2411 _ w2441 _ w2451 w2456 w2461 w2509 w2547 w2567 w2577 w2588 w2607 w2633 w2659 w2670 w2731 w2764 w2803 w2831 w2833]
              tunnel: [w2065 w2103 w2110 w2117 w2151 w2155 w2170 w2175 w2193 w2320 w2360 w2387 w2401 w2410 w2426 w2434 cluster{"Procedure":variant[]}[] [] ("t") w2451 w2459 w2478 w2509 w2548 w2568 w2578 w2588 w2607 w2633 w2659 w2670 w2731 w2764 w2803 w2831 w2833] -> w2049
              tunnel: [w2066 w2100 w2108 w2118 w2144 w2156 w2163 w2173 w2192 w2321 w2351 w2384 w2394 w2418 _ w2438 _ w2449 w2457 w2475 w2508 w2539 w2566 w2576 w2587 _ w2613 w2651 w2669 w2730 w2735 w2782 w2830 errorcluster {"status"=TRUE, "code"=-1, "source"="NO-OP is not a funtion"} ("error out")] -> w2042
              tunnel: [_ _ _ _ _ _ w2168 _ _ _ _ _ _ _ _ _ _ _ _ _ _ _ _ _ _ _ _ _ _ _ _ _ _ _] -> w2048
              tunnel: ["Engine execution" w2099 w2107 _ _ _ _ _ _ _ _ _ _ _ _ _ _ _ _ _ _ _ w2561 w2571 "RIO Snapshot" _ w2610 w2642 _ _ _ _ _ _] -> w2046
              tunnel: [_ _ _ _ _ _ _ _ _ _ _ _ _ _ _ _ _ _ w2452 _ _ w2541 w2560 w2570 _ _ _ _ _ _ _ _ _ _] -> w2041
              tunnel: w2040 -> [w2060 _ _ _ _ _ _ _ _ _ _ _ _ _ _ _ _ _ _ _ _ _ _ _ _ _ _ _ _ _ _ _ _ _]
              frame "ENG.EXECUTE" {
                w2057 = ""  # Proc
                # "\"ENG.EXECUTE\" \nCall engine execution"
                n1126 = Variant To Data(type=w2057, Variant=w2064) -> (data=w2056:string, error out=w2055:errorcluster)  [unwired: 1 in]
                n1127 = case shown="Default" w2056 {
                  selector: w2056 -> [_ w2079]
                  tunnel: [w2077 w2083] -> w2059
                  tunnel: [w2076 w2082] -> w2058
                  tunnel: w2063 -> [_ w2081]
                  tunnel: w2055 -> [w2076 w2078]
                  frame "" {
                    w2077 = -1  # execute all
                    # "run all if called w/o name"
                  }
                  frame Default {
                    # "run single proc using name"
                    n1128 = call "util.procs.find-by-name.vi"("isRequired(T)"=TRUE ("isRequired"), "error in"=w2078, "ProcName in"=w2079, "Procs in"=w2081) -> ("error out"=w2082:errorcluster, "procIndex"=w2083:i32)  [unwired: 2 in, 4 out]
                  }
                }
                n1129 = disable-structure shown="Enabled" {
                  disable-tunnel: [w2073 w2075] -> w2065
                  disable-tunnel: w2059 -> [w2072 _]
                  disable-tunnel: w2058 -> [w2071 w2074]
                  disable-tunnel: w2063 -> [w2070 w2075]
                  disable-tunnel: w2060 -> [w2069 _]
                  disable-tunnel: [w2068 w2074] -> w2054
                  disable-tunnel: [w2067 _] -> w2053
                  frame Enabled {
                    n1130 = call "engine.executor.vi"("error"=w2071, "Index(-1: All)"=w2072, "clk (NaN)"=w2069, "Procs in"=w2070) -> ("Error"=w2068:errorcluster, "Procs out"=w2073:cluster{"proc out":variant[]}[], "ErrorProcs out"=w2067:T98)  [unwired: 4 in, 1 out]
                  }
                  frame Disabled {
                  }
                }
                n1131 = stacked-sequence {
                  tunnel: w2054 -> [_ w2091]
                  tunnel: w2053 -> [_ _]
                  tunnel: [_ w2092] -> w2061
                  tunnel: w2060 -> [w2086 _]
                  frame #0 {
                    n1132 = To Time Stamp(1:w2086) -> (0:w2085:timestamp)
                    n1133 = Get Date/Time String(seconds (now)=w2085, want seconds? (F)=TRUE) -> (date string=w2090:string, time string=w2089:string)  [unwired: 1 in]
                    n1134 = Format Into String(format string="%s %s", w2090, w2089) -> (resulting string=w2084:string)  [unwired: 2 in, 1 out]
                    n1135 = local write "clock"(w2084) -> ()
                  }
                  frame #1 {
                    n1136 = property on="ProcedureStep" class="Bool (strict)"() -> ("Value"=w2093:bool)  [unwired: 2 in, 2 out]
                    n1137 = property on="Step" class="Bool (strict)"() -> ("Value"=w2095:bool)  [unwired: 2 in, 2 out]
                    n1138 = Or(x=w2095, y=w2093) -> (x .or. y?=w2094:bool)
                    n1139 = case shown="True" w2094 {
                      tunnel: [_ w2098] -> w2092
                      tunnel: w2091 -> [_ w2096]
                      frame False {
                      }
                      frame True {
                        w2097 = FALSE ("flagEngRunStep")
                        n1140 = property on="Step" class="Bool (strict)"("Value"=w2097) -> ()  [unwired: 2 in, 2 out]
                        n1141 = property on="ProcedureStep" class="Bool (strict)"("Value"=w2097) -> ()  [unwired: 2 in, 2 out]
                        n1142 = call "eng-call-start.vi"("error in (no error)"=w2096, "Start(T)/Stop(F)"=w2097) -> ("error out"=w2098:errorcluster)  [unwired: 9 in]
                      }
                    }
                  }
                }
                n1143 = Merge Errors(w2061) -> (w2066:errorcluster)
              }
              frame "ENG.START" {
                w2099 = "Engine Started" ("t")
                # "\"ENG.RUN\" \nStart/stop runtime engine by changing Timeout"
                n1144 = local read "ENG ms ctrl"() -> (w2102:i32)
                n1145 = local write "ENG ms"(w2102) -> ()
                n1146 = local write "clock"(w2099) -> ()
                n1147 = disable-structure shown="Disabled" {
                  frame Enabled {
                    n1148 = property on="clock" class="Str"("Blinking"=FALSE) -> ()  [unwired: 2 in, 2 out]
                  }
                  frame Disabled {
                    n1149 = property on="User messages" class="Str"("Text.TextColor"=u32 0 ("Color Box")) -> ()  [unwired: 2 in, 2 out]
                  }
                }
                n1150 = property on="Run" class="Bool (strict)"("Value"=TRUE) -> (error out=w2100:errorcluster)  [unwired: 2 in, 1 out]
              }
              frame "ENG.STOP" {
                w2106 = -1 items=["ENG_STOP(-1)"=-1] ("UiInterval")
                w2107 = "Engine Paused" ("t")
                # "\"ENG.RUN\" \nStart/stop runtime engine by changing Timeout"
                n1151 = property on="Run" class="Bool (strict)"("Value"=FALSE) -> (error out=w2108:errorcluster)  [unwired: 2 in, 1 out]
                n1152 = disable-structure shown="Enabled" {
                  frame Enabled {
                    n1153 = property on="clock" class="Str"("Blinking"=TRUE) -> ()  [unwired: 2 in, 2 out]
                  }
                  frame Disabled {
                    n1154 = property on="User messages" class="Str"("Text.TextColor"=u32 16711680 ("Color Box")) -> ()  [unwired: 2 in, 2 out]
                  }
                }
                n1155 = local write "clock"(w2107) -> ()
                n1156 = local write "ENG ms"(w2106) -> ()
              }
              frame "ENG.STATUS" {
                # "\"ENG.STATUS\" \n1) create list of proc names (and paths) and update proc selectors\n2) call LOG.STATUS"
                n1157 = for "create list of proc names and set proc selectors" {
                  tunnel: w2117 -> [w2131] mode=indexing
                  tunnel: [w2130] -> w2114 mode=indexing
                  tunnel: [w2129] -> w2115 mode=indexing
                  n1158 = stacked-sequence {
                    tunnel: w2131 -> [w2137 w2143]
                    tunnel: [w2132 _] -> w2130
                    tunnel: [_ w2138] -> w2129
                    frame #0 {
                      n1159 = Unbundle(w2137) -> ("Procedure"=w2134:variant[])
                      n1160 = Index Array(array=w2134) -> (element=w2133:variant)  [unwired: 1 in]
                      n1161 = call "proc.util.enumToStrProcVar.vi"("Proc var"=typeProcVarientName."procNameID" ("proc var")) -> ("String"=w2136:string)  [unwired: 10 in]
                      n1162 = call-poly "variantCtrl.polymorphic.vi"("name in"=w2136, "Step in"=w2133) -> ("String Value"=w2132:string)  [unwired: 6 in, 3 out]
                    }
                    frame #1 {
                      n1163 = Unbundle(w2143) -> ("Procedure"=w2140:variant[])
                      n1164 = Index Array(array=w2140) -> (element=w2139:variant)  [unwired: 1 in]
                      n1165 = call "proc.util.enumToStrProcVar.vi"("Proc var"=typeProcVarientName."procPath" ("proc var")) -> ("String"=w2142:string)  [unwired: 10 in]
                      n1166 = call-poly "variantCtrl.polymorphic.vi"("name in"=w2142, "Step in"=w2139) -> ("String Value"=w2138:string)  [unwired: 6 in, 3 out]
                    }
                  }
                }
                n1167 = local write "Loaded Proc Path"(w2115) -> ()
                n1168 = Index Array(array=w2114) -> (element=w2113:string)  [unwired: 1 in]
                n1169 = property on="Proc Name" class="CmbBox"("Strings[]"=w2114, "Value"="" ("Proc Name")) -> ()  [unwired: 2 in, 2 out]
                n1170 = property on="ProcedureSelect" class="CmbBox"("Strings[]"=w2114, "Value"=w2113) -> ()  [unwired: 2 in, 2 out]
                n1171 = disable-structure shown="Enabled" {
                  disable-tunnel: [w2122 w2127 _] -> w2118
                  disable-tunnel: w2117 -> [w2119 _ _]
                  frame Disabled {
                    n1172 = global read "globals-engine.vi" "Q-Log"() -> (w2123:refnum<queue>)
                    n1173 = Bundle By Name(cluster=cluster{"data":variant, "Enum":T57} {"data"=variant, "Enum"=enum."LOG.UPDATE.SELECTORS"} ("procQ"), "data"=w2119) -> (w2120:cluster{"data":variant, "Enum":T57})
                    n1174 = Enqueue Element(queue=w2123, element=w2120) -> (error out=w2122:errorcluster)  [unwired: 2 in, 2 out]
                  }
                  frame Enabled {
                    n1175 = global read "globals-engine.vi" "Q-Log"() -> (w2128:refnum<queue>)
                    n1176 = Bundle By Name(cluster=cluster{"data":variant, "Enum":T57} {"data"=variant, "Enum"=enum."LOG.UPDATE.SELECTORS"} ("procQ"), "data"=variant) -> (w2125:cluster{"data":variant, "Enum":T57})
                    n1177 = Enqueue Element(queue=w2128, element=w2125) -> (error out=w2127:errorcluster)  [unwired: 2 in, 2 out]
                  }
                  frame Disabled {
                  }
                }
                n1178 = property on="Proc Select 2" class="CmbBox"("Strings[]"=w2114, "Value"=w2113) -> ()  [unwired: 2 in, 2 out]
              }
              frame "ENG.EXTERNAL-CALL" {
                n1179 = Variant To Data(type=T82 {"Q-Log"=refnum, "procQ"={"data"=variant, "Enum"=enum."LOG.NO_OP"}} ("output cluster"), Variant=w2149) -> (data=w2148:T82, error out=w2145:errorcluster)  [unwired: 1 in]
                n1180 = Unbundle By Name(w2148) -> ("Q-Log"=w2147:refnum<queue>, "procQ"=w2146:cluster{"data":variant, "Enum":T57})
                n1181 = Enqueue Element(queue=w2147, element=w2146, error in (no error)=w2145) -> (error out=w2144:errorcluster)  [unwired: 1 in, 2 out]
              }
              frame "ENG.PROC.STATUS" {
                n1182 = global read "globals-engine.vi" "Q-Log"() -> (w2154:refnum<queue>)
                n1183 = Bundle By Name(cluster=cluster{"data":variant, "Enum":T57} {"data"=variant, "Enum"=enum."LOG.SNAPSHOT.PROC"} ("procQ"), "data"=w2155) -> (w2152:cluster{"data":variant, "Enum":T57})
                n1184 = Enqueue Element(queue=w2154, element=w2152) -> (error out=w2156:errorcluster)  [unwired: 2 in, 2 out]
              }
              frame "ENG.EXIT" {
                w2168 = TRUE
                # "\"ENG.EXIT\""
                n1185 = Release Queue(queue=w2169) -> (error out=w2164:errorcluster)  [unwired: 2 in, 2 out]
                n1186 = global write "globals-engine.vi" "STOP"(w2168) -> ()
                n1187 = global read "globals-engine.vi" "Q-Log"() -> (w2166:refnum<queue>)
                n1188 = Enqueue Element(queue=w2166, element=cluster{"data":variant, "Enum":T57} {"data"=variant, "Enum"=enum."LOG.EXIT"} ("procQ")) -> (error out=w2167:errorcluster)  [unwired: 2 in, 2 out]
                n1189 = global read "globals-engine.vi" "Q-Com"() -> (w2162:refnum<queue>)
                n1190 = Enqueue Element(queue=w2162, element=cluster{"data":variant, "Enum":T55} {"data"=variant, "Enum"=enum."REC.EXIT"}) -> (error out=w2160:errorcluster)  [unwired: 2 in, 2 out]
                n1191 = global read "globals-engine.vi" "Q-Sched"() -> (w2159:refnum<queue>)
                n1192 = Enqueue Element(queue=w2159, element=cluster{"data":variant, "Enum":T54} {"data"=variant, "Enum"=enum."SCHED.EXIT"}) -> (error out=w2157:errorcluster)  [unwired: 2 in, 2 out]
                n1193 = Merge Errors(w2157, w2160, w2167, w2164) -> (w2163:errorcluster)
              }
              frame "ENG.INIT" {
                # "initialize engine before loading runtime procedures"
                n1194 = for {
                  tunnel: w2174 -> [w2178]
                  tunnel: [w2177] -> w2172
                  tunnel: cluster{"cmd":T5, "data":variant}[] [{"cmd"=enum."ENG.INIT.SERIAL", "data"=variant}, {"cmd"=enum."ENG.INIT.VARS", "data"=variant}] ("typedefElement") -> [w2176] mode=indexing
                  n1195 = Enqueue Element At Opposite End(queue=w2178, element=w2176) -> (error out=w2177:errorcluster)  [unwired: 2 in, 2 out]
                }
                n1196 = Merge Errors(w2172) -> (w2173:errorcluster)
              }
              frame "ENG.INIT.VARS" {
                # "initialize Globals (nutritionConf)"
                n1197 = stacked-sequence {
                  seq-local: [_ _ _ w2217 _ _ _] -> [_ _ _ _ w2306 _ _]
                  tunnel: [_ w2197 _ _ _ _ _] -> w2191
                  tunnel: [_ _ w2211 _ _ _ _] -> w2190
                  tunnel: [w2195 _ _ _ _ _ _] -> w2189
                  tunnel: [_ _ _ w2217 _ _ _] -> w2182
                  tunnel: [_ _ _ w2222 _ _ _] -> w2188
                  tunnel: [w2194 _ _ _ _ _ _] -> w2187
                  tunnel: [_ w2196 _ _ _ _ _] -> w2186
                  tunnel: [_ _ _ w2220 _ _ _] -> w2185
                  tunnel: [_ _ _ w2219 _ _ _] -> w2184
                  tunnel: [_ _ _ w2218 _ _ _] -> w2183
                  tunnel: [_ _ w2208 _ _ _ _] -> w2181
                  tunnel: [_ _ _ _ _ w2312 _] -> w2180
                  tunnel: [_ _ _ _ _ _ w2313] -> w2179
                  frame #0 {
                    # "load aux list"
                    n1198 = call "aux-conf-loader.vi"() -> ("error out"=w2195:errorcluster, "Array"=w2194:T99[])  [unwired: 10 in]
                  }
                  frame #1 {
                    # "Nutrition GLOBAL"
                    n1199 = call "util.file.vars.vi"("Directory (DIR_PROC)"=typePathSelector."DIR_CONFIG" ("location (PROCEDURE_DIR)"), "Proc Name(open dialog if empty)"="unit-nutrition" ("Filename.*  (opens dialog if empty and allow)")) -> ("error out"=w2199:errorcluster, "Vars[] out"=w2200:variant[])  [unwired: 5 in, 3 out]
                    n1200 = for {
                      tunnel: w2200 -> [w2207] mode=indexing
                      tunnel: [w2206] -> w2196 mode=indexing
                      tunnel: w2199 -> [w2204]
                      tunnel: [w2203] -> w2198
                      n1201 = Variant To Data(error in=w2204, type=T65 {"Main"={"Enable"=FALSE, "WashTimes"={"In"=0.0, "Out"=0.0}, "DailyActivityHours"=[]}, "Water Dosing"={"Water Dose"=0.0, "Water Limit"=0.0}, "EC Ranges"={"H Alarm"=0.0, "L Alarm"=0.0, "Low"=0.0}, "EC Dosing"={"ALFA1 Dose"=0.0, "ALFA1 Limit"=0.0, "BETA1 Dose"=0.0, "BETA1 Limit"=0.0, "ALFA2 Dose"=0.0, "ALFA2 Limit"=0.0, "BETA2 Dose"=0.0, "BETA2 Limit"=0.0}, "PH Ranges"={"H Alarm"=0.0, "L Alarm"=0.0, "High"=0.0, "Low"=0.0}, "PH Dosing"={"ACID Dose"=0.0, "ACID Limit"=0.0, "BASE Dose"=0.0, "BASE Limit"=0.0}, "ORP Ranges"={"H Alarm"=0.0, "L Alarm"=0.0, "Low"=0.0}, "ORP Dosing"={"MIX Dose"=0.0, "MIX Limit"=0.0}} ("Cluster"), Variant=w2207) -> (data=w2206:T65, error out=w2203:errorcluster)
                    }
                    n1202 = Merge Errors(w2198) -> (w2197:errorcluster)
                  }
                  frame #2 {
                    # "irrigation GLOBAL"
                    n1203 = call "util.file.vars.vi"("Directory (DIR_PROC)"=typePathSelector."DIR_CONFIG" ("location (PROCEDURE_DIR)"), "Proc Name(open dialog if empty)"="IRR_CONF" ("Filename.*  (opens dialog if empty and allow)")) -> ("error out"=w2213:errorcluster, "Vars[] out"=w2214:variant[])  [unwired: 5 in, 3 out]
                    n1204 = Index Array(array=w2214) -> (element=w2210:variant)  [unwired: 1 in]
                    n1205 = Variant To Data(error in=w2213, type=T31 {"Day Time"={"Sunset"=timestamp(0 s since 1904-01-01), "Sunrise"=timestamp(0 s since 1904-01-01)}, "timeLimits"={"Irrigation"=0.0, "Nut./Water"=0.0}, "Calculated Timing"={"Irrigation Timeout"=timestamp(0 s since 1904-01-01), "Nutrients Timeout"=timestamp(0 s since 1904-01-01)}, "Irr Dosing Time"={"Nutrients"=250, "Water"=250, "Wash"=250}, "UV Limit "=250.0, "Dose Table"=[{"Enable"=TRUE, "output"="IRR_SEC1"}, {"Enable"=FALSE, "output"="IRR_SEC2"}, {"Enable"=FALSE, "output"="IRR_SEC3"}, {"Enable"=FALSE, "output"="IRR_SEC4"}, {"Enable"=FALSE, "output"="IRR_SEC5"}, {"Enable"=FALSE, "output"="IRR_SEC6"}], "Last Iteration"=timestamp(0 s since 1904-01-01), "UV Reduction Status"=FALSE, "UV Reduction"=99} ("irr panel"), Variant=w2210) -> (data=w2208:T31, error out=w2212:errorcluster)
                    n1206 = Merge Errors(w2212) -> (w2211:errorcluster)
                  }
                  frame #3 {
                    w2221 = 500  # ms default
                    # "INI to GLOBALs"
                    n1207 = call "util-path.vi"("Create Folders?(F)"=FALSE, "Selected Folder (PROCS)"=typePathSelector."DIR_INI" ("Selected Folder (PROCEDURE_DIR)")) -> ("error out"=w2229:errorcluster, "SelectedPath"=w2230:path)  [unwired: 5 in, 3 out]
                    n1208 = call <vilib>:"Open Config Data.vi"("error in (no error)"=w2229, "configuration file path"=w2230) -> ("error out"=w2223:errorcluster, "refnum"=w2226:T64)  [unwired: 7 in, 1 out]
                    n1209 = case shown="No Error" w2223 {
                      selector: w2223 -> [_ w2300]
                      tunnel: [w2250 _] -> w2233
                      tunnel: [w2249 _] -> w2232
                      tunnel: [w2248 _] -> w2231
                      tunnel: w2226 -> [w2247 w2299]
                      tunnel: [w2246 w2299] -> w2225
                      tunnel: [w2244 w2300] -> w2224
                      tunnel: [w2240 _] -> w2220
                      tunnel: [w2238 w2298] -> w2219
                      tunnel: w2221 -> [w2237 w2298]
                      tunnel: [w2235 _] -> w2218
                      frame No Error {
                        n1210 = stacked-sequence {
                          tunnel: [w2254 _ _ _ _ _] -> w2248
                          tunnel: [_ w2261 _ _ _ _] -> w2249
                          tunnel: [_ _ w2267 _ _ _] -> w2250
                          tunnel: [_ w2259 _ _ _ _] -> w2243
                          tunnel: w2247 -> [w2253 w2258 w2265 w2272 w2281 w2294]
                          tunnel: [w2252 _ _ _ _ _] -> w2245
                          tunnel: [w2251 _ _ _ _ _] -> w2246
                          tunnel: [_ _ w2264 _ _ _] -> w2242
                          tunnel: [_ _ _ w2271 _ _] -> w2241
                          tunnel: [_ _ _ w2270 _ _] -> w2240
                          tunnel: [_ _ _ _ w2280 _] -> w2239
                          tunnel: [_ _ _ _ w2279 _] -> w2238
                          tunnel: w2237 -> [_ _ _ _ w2276 _]
                          tunnel: [_ _ _ _ _ w2291] -> w2236
                          tunnel: [_ _ _ _ _ w2285] -> w2235
                          frame #0 {
                            n1211 = call "util-ini-key.vi"("key"=ini-key."INI.LOCAL.LONGITUDE" ("input 1")) -> ("key"=w2257:string, "section"=w2255:string)  [unwired: 9 in]
                            n1212 = call-poly <vilib>:"Read Key.vi"("section"=w2255, "key"=w2257, "refnum"=w2253) -> ("error out"=w2252:errorcluster, "value"=w2254:dbl, "refnum out"=w2251:T64)  [unwired: 5 in, 1 out]
                          }
                          frame #1 {
                            n1213 = call "util-ini-key.vi"("key"=ini-key."INI.LOCAL.LATITUDE" ("input 1")) -> ("key"=w2263:string, "section"=w2260:string)  [unwired: 9 in]
                            n1214 = call-poly <vilib>:"Read Key.vi"("section"=w2260, "key"=w2263, "refnum"=w2258) -> ("error out"=w2259:errorcluster, "value"=w2261:dbl)  [unwired: 5 in, 2 out]
                          }
                          frame #2 {
                            n1215 = call "util-ini-key.vi"("key"=ini-key."INI.LOCAL.TIMEZONE" ("input 1")) -> ("key"=w2269:string, "section"=w2266:string)  [unwired: 9 in]
                            n1216 = call-poly <vilib>:"Read Key.vi"("section"=w2266, "key"=w2269, "refnum"=w2265) -> ("error out"=w2264:errorcluster, "value"=w2267:dbl)  [unwired: 5 in, 2 out]
                          }
                          frame #3 {
                            n1217 = call "util-ini-key.vi"("key"=ini-key."INI.PROJECT_NAME" ("input 1")) -> ("key"=w2275:string, "section"=w2273:string)  [unwired: 9 in]
                            n1218 = call-poly <vilib>:"Read Key.vi"("section"=w2273, "key"=w2275, "refnum"=w2272) -> ("error out"=w2271:errorcluster, "value"=w2270:string)  [unwired: 5 in, 2 out]
                          }
                          frame #4 {
                            n1219 = call "util-ini-key.vi"("key"=ini-key."INI.ENG.INTERVAL_MS" ("input 1")) -> ("key"=w2284:string, "section"=w2282:string)  [unwired: 9 in]
                            n1220 = call-poly <vilib>:"Read Key.vi"("section"=w2282, "key"=w2284, "refnum"=w2281) -> ("error out"=w2280:errorcluster, "value"=w2278:i32, "found?"=w2277:bool)  [unwired: 5 in, 1 out]
                            n1221 = Select(t=w2278, s=w2277, f=w2276) -> (s? t:f=w2279:i32)
                          }
                          frame #5 {
                            w2287 = typeEnv."ENV.PRODUCTION" ("ENV in")
                            n1222 = call "util-ini-key.vi"("key"=ini-key."INI.ENV" ("input 1")) -> ("key"=w2297:string, "section"=w2295:string)  [unwired: 9 in]
                            n1223 = call-poly <vilib>:"Read Key.vi"("section"=w2295, "key"=w2297, "refnum"=w2294) -> ("error out"=w2292:errorcluster, "value"=w2290:string, "found?"=w2289:bool)  [unwired: 5 in, 1 out]
                            n1224 = Scan From String(input string=w2290, default 1=w2287) -> (output 1=w2288:T1)  [unwired: 3 in, 3 out]
                            n1225 = Select(t=w2288, s=w2289, f=w2287) -> (s? t:f=w2286:T1)
                            n1226 = call "util.environment.vi"("error in"=w2292, "Operation (Get)"=enum16{"get", "set"}."set", "ENV in"=w2286) -> ("error out"=w2291:errorcluster, "ENV out"=w2285:T1)  [unwired: 7 in]
                          }
                        }
                        n1227 = Merge Errors(w2245, w2243, w2242, w2241, w2239, w2236) -> (w2244:errorcluster)
                      }
                      frame Error {
                      }
                    }
                    n1228 = global read "globals-engine.vi" "ProjectSettings"() -> (w2234:T12)
                    n1229 = Bundle By Name(cluster=w2234, "Longitude"=w2231, "Latitude"=w2232, "TimeZone"=w2233) -> (w2217:T12)
                    n1230 = call <vilib>:"Close Config Data.vi"("error in (no error)"=w2224, "refnum"=w2225) -> ("error out"=w2222:errorcluster)  [unwired: 8 in, 1 out]
                  }
                  frame #4 {
                    n1231 = Unbundle By Name(w2306) -> ("Latitude"=w2304:dbl, "Longitude"=w2303:dbl, "TimeZone"=w2302:i32)
                    n1232 = local read "UiProjectSettings"() -> (w2305:T19)
                    n1233 = Bundle By Name(cluster=w2305, "Latitude"=w2304, "Longitude"=w2303, "TimeZone"=w2302) -> (w2301:T19)
                    n1234 = local write "UiProjectSettings"(w2301) -> ()
                  }
                  frame #5 {
                    # "INIT PBR PROC SELECTOR"
                    n1235 = call "pbr-get-procs-names.vi"() -> ("error out"=w2312:errorcluster, "Array"=w2311:string[])  [unwired: 10 in]
                    n1236 = local write "PBR Builder"(T23 [] ("PBR Builder")) -> ()
                    n1237 = local write "PBR_PLAY"(cluster{"PLAY":bool, "PAUSE":bool, "STOP":bool} {"PLAY"=FALSE, "PAUSE"=FALSE, "STOP"=FALSE} ("PBR_PLAY")) -> ()
                    n1238 = local write "source"("" ("source")) -> ()
                    n1239 = property on="PBR PROC" class="CmbBox"("Strings[]"=w2311, "Value"="" ("source")) -> ()  [unwired: 2 in, 2 out]
                  }
                  frame #6 {
                    n1240 = global read "globals-engine.vi" "Q-Log"() -> (w2314:refnum<queue>)
                    n1241 = for {
                      tunnel: cluster{"data":variant, "Enum":T57}[] [{"data"=variant, "Enum"=enum."LOG.INIT"}, {"data"=variant, "Enum"=enum."LOG.UPDATE.IRR"}] ("procQ") -> [w2319] mode=indexing
                      shift-right: [w2317] -> w2313
                      shift-left: _ -> [w2316]
                      tunnel: w2314 -> [w2318]
                      n1242 = Enqueue Element(queue=w2318, element=w2319, error in (no error)=w2316) -> (error out=w2317:errorcluster)  [unwired: 1 in, 2 out]
                    }
                  }
                }
                n1243 = local write "ENG ms ctrl"(w2184) -> ()
                n1244 = local write "ENV"(w2183) -> ()
                n1245 = local write "ProjectSettings"(w2182) -> ()
                n1246 = global write "globals-engine.vi" "ProjectSettings"(w2182) -> ()
                n1247 = local write "AuxiliaryList"(w2187) -> ()
                n1248 = global write "globals-engine.vi" "NutritionConfiguration"(w2186) -> ()
                n1249 = local write "IRR Params"(w2181) -> ()
                n1250 = global write "globals-engine.vi" "IRR Params"(w2181) -> ()
                n1251 = local write "projectName"(w2185) -> ()
                n1252 = Merge Errors(w2188, w2191, w2190, w2189, w2180, w2179) -> (w2192:errorcluster)
              }
              frame "ENG.INIT.SERIAL" {
                # "initialize:\nGlobals (nutritionConf)\nSerial port\ncall ENG.IO.LOAD"
                n1253 = disable-structure shown="Enabled" {
                  disable-tunnel: [w2328 _] -> w2321
                  frame Disabled {
                    w2324 = T59[] [enum."INI.ENG.SERIAL"] items=["INI.PROJECT_NAME", "INI.ENV", "INI.ENG.SERIAL", "INI.ENG.INTERVAL_MS", "INI.LOCAL.LONGITUDE", "INI.LOCAL.LATITUDE", "INI.LOCAL.TIMEZONE"] ("keys")
                    n1254 = feedback #4() -> ()  [unwired: 2 in]
                    n1255 = feedback-in #4() -> ()  [unwired: 1 out]
                    n1256 = call "util.file.ini.vi"("Section"="LOCAL" ("element"), "keys"=w2324) -> ("values"=w2325:string[])  [unwired: 7 in, 2 out]
                    n1257 = disable-structure shown="Disabled" {
                      frame Disabled {
                        n1258 = case shown="Error .." {
                          selector: _ -> [w2329 _]
                          tunnel: [w2329 w2330] -> _
                          frame No Error {
                          }
                          frame Error {
                            w2332 = T100 2 items=["Canonical Names Only"=0, "Aliases Only"=2, "Include Matching Aliases"=3, "Include All Aliases"=4] ("Search Mode")
                            # "TODO auto scan serial port"
                            n1259 = VISA Find Resource(10:w2332) -> (3:w2333:string[])  [unwired: 2 in, 2 out]
                            n1260 = Reverse 1D Array(array=w2333) -> (reversed array=w2331:string[])
                            n1261 = for {
                              tunnel: w2331 -> [w2334] mode=indexing
                              tunnel: [w2335] -> w2330
                              shift-right: [w2334] -> _
                              shift-left: _ -> [_]
                              stop <- w2335 continue-if-true
                              n1262 = call "util-serial-init.vi"("NewVal"=w2334) -> ("error out"=w2335:errorcluster)  [unwired: 10 in]
                            }
                          }
                        }
                      }
                      frame Enabled {
                      }
                    }
                    n1263 = Index Array(array=w2325) -> (element=w2327:string)  [unwired: 1 in]
                    n1264 = call "util-serial-init.vi"("NewVal"=w2327, "Port"=w2327) -> ("error out"=w2322:errorcluster)  [unwired: 9 in]
                    n1265 = property on="SerialPort" class="VISAName"(error in=w2322, "Value"=w2327) -> (error out=w2326:errorcluster)  [unwired: 1 in, 1 out]
                    n1266 = Merge Errors(w2326) -> (w2328:errorcluster)
                  }
                  frame Enabled {
                    n1267 = call "util-path.vi"("Create Folders?(F)"=FALSE, "Selected Folder (PROCS)"=typePathSelector."DIR_INI" ("Selected Folder (PROCEDURE_DIR)")) -> ("error out"=w2348:errorcluster, "SelectedPath"=w2346:path)  [unwired: 5 in, 3 out]
                    n1268 = call <vilib>:"Open Config Data.vi"("error in (no error)"=w2348, "configuration file path"=w2346) -> ("error out"=w2347:errorcluster, "refnum"=w2345:T64)  [unwired: 7 in, 1 out]
                    n1269 = call "util-ini-key.vi"("key"=ini-key."INI.ENG.SERIAL" ("input 1")) -> ("key"=w2342:string, "section"=w2341:string)  [unwired: 9 in]
                    n1270 = call-poly <vilib>:"Read Key.vi"("section"=w2341, "error in (no error)"=w2347, "key"=w2342, "refnum"=w2345) -> ("error out"=w2344:errorcluster, "value"=w2337:string, "found?"=w2336:bool, "refnum out"=w2343:T64)  [unwired: 4 in]
                    n1271 = case shown="True" w2336 {
                      tunnel: w2337 -> [_ w2349]
                      frame False {
                      }
                      frame True {
                        n1272 = property on="SerialPort" class="VISAName"("Val(Sgnl)"=w2349) -> ()  [unwired: 2 in, 2 out]
                      }
                    }
                    n1273 = call <vilib>:"Close Config Data.vi"("error in (no error)"=w2344, "refnum"=w2343) -> ()  [unwired: 8 in, 2 out]
                  }
                }
              }
              frame "ENG.IO.LOAD" {
                # "let the LOG.status update IOconf local variable so search can work\nwithout the need to trigger io-reg for the io list"
                # "\"ENG.LOAD\" \n load i/o from filesystem to global variable"
                n1274 = Variant To Data(type=T42[] [] ("IO Conf"), Variant=w2355) -> (data=w2354:T42[], error out=w2353:errorcluster)  [unwired: 1 in]
                n1275 = case shown="Error .." w2353 {
                  tunnel: [w2367 w2372] -> w2359
                  tunnel: [_ w2371] -> w2358
                  tunnel: w2354 -> [w2367 _]
                  frame No Error {
                    # "read from Queue"
                  }
                  frame Error {
                    # "read from fs"
                    n1276 = call "util-path.vi"("Selected Folder (PROCS)"=typePathSelector."DIR_IO_FILE") -> ("error out"=w2368:errorcluster, "SelectedPath"=w2369:path)  [unwired: 6 in, 3 out]
                    n1277 = call "util-io-csv-load.vi"("error in"=w2368, "file path (dialog if empty)"=w2369) -> ("error out"=w2371:errorcluster, "Array"=w2372:T42[])  [unwired: 8 in]
                  }
                }
                n1278 = call "variantCtrlIo.vi"("menu (Get Param)"=enumVarCtrlIO."IO Remove All" ("menu (get)"), "error in"=w2358) -> ("error out"=w2356:errorcluster)  [unwired: 5 in, 4 out]
                n1279 = for {
                  tunnel: w2359 -> [w2373] mode=indexing
                  tunnel: [w2376] -> w2350
                  tunnel: w2356 -> [w2374]
                  stop <- w2376 stop-if-true
                  n1280 = call "variantCtrlIo.vi"("menu (Get Param)"=enumVarCtrlIO."IO Add By Key" ("menu (get)"), "error in"=w2374, "IOnode in"=w2373) -> ("error out"=w2376:errorcluster)  [unwired: 4 in, 4 out]
                }
                n1281 = disable-structure shown="Disabled" {
                  frame Disabled {
                    n1282 = global read "globals-engine.vi" "Q-Log"() -> (w2362:refnum<queue>)
                    n1283 = Enqueue Element(queue=w2362, element=cluster{"data":variant, "Enum":T57} {"data"=variant, "Enum"=enum."LOG.UPDATE.SELECTORS"} ("procQ")) -> ()  [unwired: 2 in, 3 out]
                  }
                  frame Enabled {
                  }
                }
                n1284 = disable-structure shown="Enabled" {
                  disable-tunnel: [w2364 w2366] -> w2351
                  disable-tunnel: w2350 -> [w2363 w2366]
                  frame Disabled {
                    n1285 = call "variantCtrlIo.vi"("menu (Get Param)"=enumVarCtrlIO."IO List Configs", "error in"=w2363) -> ("error out"=w2364:errorcluster)  [unwired: 5 in, 4 out]
                  }
                  frame Enabled {
                  }
                }
              }
              frame "ENG.IO.SAVE" {
                # "TODO add file name or dialog"
                # "\"ENG.LOAD\" \n load i/o from filesystem to global variable"
                n1286 = call "variantCtrlIo.vi"("menu (Get Param)"=enumVarCtrlIO."IO List Configs" ("menu (get)")) -> ("IO Configs List"=w2378:T42[])  [unwired: 6 in, 4 out]
                n1287 = call "util-io-sort.vi"("IO Configs List"=w2378) -> ("Result"=w2382:T42[])  [unwired: 10 in]
                n1288 = Array Size(array=w2382) -> (size(s)=w2381:i32)
                n1289 = call "util-path.vi"("Selected Folder (PROCS)"=typePathSelector."DIR_IO_FILE" ("Selected Folder (PROCEDURE_DIR)")) -> ("error out"=w2385:errorcluster, "SelectedPath"=w2377:path)  [unwired: 6 in, 3 out]
                n1290 = Format Into String(format string="Save %d IO nodes as %s?", w2381, w2377) -> (resulting string=w2380:string)  [unwired: 2 in, 1 out]
                n1291 = Two Button Dialog(message=w2380) -> (T button?=w2379:bool)  [unwired: 2 in]
                n1292 = case shown="True" w2379 {
                  tunnel: w2377 -> [_ w2393]
                  tunnel: w2385 -> [w2389 w2392]
                  tunnel: [w2389 w2391] -> w2384
                  tunnel: w2382 -> [_ w2390]
                  frame False {
                  }
                  frame True {
                    n1293 = call "util-io-csv-save.vi"("error out"=w2392, "file path (dialog if empty)"=w2393, "IO Nodes"=w2390) -> ("error out"=w2391:errorcluster)  [unwired: 8 in]
                  }
                }
              }
              frame "ENG.LOAD" {
                # "\"ENG.LOAD\" \nLoads all procs from filesystem as it should be loaded in production (read all procs from procedure folder)"
                n1294 = call "util-path.vi"() -> ("error out"=w2397:errorcluster, "SelectedPath"=w2398:path)  [unwired: 7 in, 3 out]
                n1295 = call <vilib>:"Recursive File List.vi"("error in (no error)"=w2397, "Folder Path"=w2398) -> ("error out"=w2396:errorcluster, "All Files in Dir"=w2395:path[])  [unwired: 5 in, 3 out]
                n1296 = for {
                  tunnel: [w2408] -> w2399 mode=indexing
                  tunnel: [w2404] -> w2394
                  tunnel: w2395 -> [w2402] mode=indexing
                  tunnel: w2396 -> [w2406]
                  stop <- w2404 stop-if-true
                  n1297 = call "util.file.vars.file-operations.vi"("error in (no error)"=w2406, "selected path"=w2402) -> ("error out"=w2405:errorcluster, "Procedure"=w2403:variant[])  [unwired: 7 in, 1 out]
                  n1298 = call "util.proc.init.vi"("error in"=w2405, "Proc Path"=w2402, "Procedure in"=w2403) -> ("error out"=w2404:errorcluster, "Procedure out"=w2407:variant[])  [unwired: 7 in]
                  n1299 = Bundle("Procedure out"=w2407) -> (w2408:cluster{"Procedure out":variant[]})  [unwired: 1 in]
                }
                n1300 = Select(t=cluster{"Procedure":variant[]}[] [], s=w2394, f=w2399) -> (s? t:f=w2401:cluster{"Procedure out":variant[]}[])
                "Loaded" <- w2401
              }
              frame "ENG.LOAD.MODULE" {
                # "\"ENG.LOAD\" \nLoads all procs from filesystem as it should be loaded in production (read all procs from procedure folder)"
                n1301 = Variant To Data(type=path "" ("procPath"), Variant=w2415) -> (data=w2413:path, error out=w2412:errorcluster)  [unwired: 1 in]
                n1302 = call <vilib>:"Recursive File List.vi"("error in (no error)"=w2412, "Folder Path"=w2413) -> ("error out"=w2417:errorcluster, "All Files in Dir"=w2416:path[])  [unwired: 5 in, 3 out]
                n1303 = for {
                  tunnel: [w2425] -> w2409 mode=indexing
                  tunnel: [w2421] -> w2418
                  tunnel: w2416 -> [w2419] mode=indexing
                  tunnel: w2417 -> [w2423]
                  stop <- w2421 stop-if-true
                  n1304 = call "util.file.vars.file-operations.vi"("error in (no error)"=w2423, "selected path"=w2419) -> ("error out"=w2422:errorcluster, "Procedure"=w2420:variant[])  [unwired: 7 in, 1 out]
                  n1305 = call "util.proc.init.vi"("error in"=w2422, "Proc Path"=w2419, "Procedure in"=w2420) -> ("error out"=w2421:errorcluster, "Procedure out"=w2424:variant[])  [unwired: 7 in]
                  n1306 = Bundle("Procedure out"=w2424) -> (w2425:cluster{"Procedure out":variant[]})  [unwired: 1 in]
                }
                n1307 = Build Array (concatenate)(w2411, w2409) -> (w2410:cluster{"Procedure out":variant[]}[])
              }
              frame "ENG.LOAD.RELOAD" {
                # "\"ENG.LOAD.RELOAD\" \nRELOAD THE LAST RUNTIME REGISTER"
                n1308 = local read "Loaded"() -> (w2426:cluster{"Procedure":variant[]}[])
              }
              frame "ENG.LOAD.SINGLE" {
                # "\"ENG.LOAD.SINGLE\"  (PROCEDURE_PATH)\nADD PROCEDURE TO RUNTIME REGISTER"
                n1309 = Variant To Data(type=path "" ("procPath"), Variant=w2437) -> (data=w2427:path, error out=w2428:errorcluster)  [unwired: 1 in]
                n1310 = call "util.file.vars.file-operations.vi"("error in (no error)"=w2428, "selected path"=w2427) -> ("error out"=w2429:errorcluster, "Procedure"=w2430:variant[])  [unwired: 7 in, 1 out]
                n1311 = call "util.proc.init.vi"("error in"=w2429, "Proc Path"=w2427, "Procedure in"=w2430) -> ("error out"=w2432:errorcluster, "Procedure out"=w2433:variant[])  [unwired: 7 in]
                n1312 = Bundle("Procedure out"=w2433) -> (w2436:cluster{"Procedure out":variant[]})  [unwired: 1 in]
                n1313 = case shown="No Error" w2432 {
                  selector: w2432 -> [_ w2446]
                  tunnel: [w2444 w2445] -> w2434
                  tunnel: w2441 -> [w2443 w2445]
                  tunnel: w2436 -> [w2442 _]
                  tunnel: [_ w2446] -> w2435
                  frame No Error {
                    n1314 = Build Array (concatenate)(w2443, w2442) -> (w2444:cluster{"Procedure out":variant[]}[])
                    n1315 = local write "Loaded"(w2444) -> ()
                  }
                  frame Error {
                  }
                }
                n1316 = Enqueue Element(queue=w2440, element=cluster{"cmd":T5, "data":variant} {"cmd"=enum."ENG.STATUS", "data"=variant} ("typedefElement"), error in (no error)=w2435) -> (error out=w2438:errorcluster)  [unwired: 1 in, 2 out]
              }
              frame "ENG.LOAD.UNLOAD" {
                # "\"ENG.LOAD.UNLOAD\" \n REMOVE ALL PROCEDURES FROM RUNTIME REGISTER"
              }
              frame "ENG.PRINT-USER-MSG" {
                # "No code required. used to release th FIFO if waiting indefinitly (-1)"
                n1317 = Variant To Data(type="" ("Value (Signaling)"), Variant=w2450) -> (error out=w2449:errorcluster)  [unwired: 1 in, 1 out]
              }
              frame "ENG.PROC.INSERT-STEPS" {
                # "\"ENG.PROC.INIT\" \nload selected proc from filesystem"
                n1318 = Variant To Data(type=T91 {"ProcName"="", "instructions"=[]}, Variant=w2460) -> (data=w2455:T91, error out=w2458:errorcluster)  [unwired: 1 in]
                n1319 = Unbundle By Name(w2455) -> ("ProcName"=w2452:string, "instructions"=w2453:variant[])
                n1320 = call "main.eng.proc-insert-instructions.vi"("error in (no error)"=w2458, "instructions in"=w2453, "procedureName"=w2452, "procs in"=w2456) -> ("error out"=w2457:errorcluster, "procs out"=w2459:cluster{"Procedure":variant[]}[])  [unwired: 6 in]
              }
              frame "ENG.PROC.ISRUNNING" {
                w2474 = "%s=%s"  # procLabel=ON/OFF
                # "\"ENG-PROC.ISRUNNING\" check if proc is running"
                n1321 = Variant To Data(type=T92 {"callerProc"="", "procPointer"=""}, Variant=w2487) -> (data=w2486:T92)  [unwired: 1 in, 1 out]
                n1322 = Unbundle By Name(w2486) -> ("callerProc"=w2463:string, "procPointer"=w2462:string)
                n1323 = call "util.procs.find-by-name.vi"("ProcName in"=w2462, "Procs in"=w2461) -> ("error out"=w2468:errorcluster, "Found?"=w2481:bool, "procIndex"=w2482:i32)  [unwired: 4 in, 3 out]
                n1324 = call "proc.util.enumToStrProcVar.vi"("Proc var"=typeProcVarientName."procIsRunning" ("Combo Box")) -> ("String"=w2483:string)  [unwired: 10 in]
                n1325 = case shown="True" w2481 {
                  selector: w2481 -> [w2499 _]
                  tunnel: [w2500 w2507] -> w2464
                  tunnel: w2461 -> [w2500 w2506]
                  tunnel: w2483 -> [_ w2502]
                  tunnel: w2482 -> [_ w2504]
                  tunnel: [w2498 w2505] -> w2467
                  tunnel: [w2499 w2501] -> w2473
                  tunnel: w2468 -> [w2498 w2503]
                  frame False {
                  }
                  frame True {
                    n1326 = call "procs.setByProcIndexBoolean.vi"("procIndex"=w2504, "error in"=w2503, "procAttribute"=w2502, "procs in"=w2506) -> ("error out"=w2505:errorcluster, "Bool out"=w2501:bool, "procs out"=w2507:cluster{"Procedure":variant[]}[])  [unwired: 5 in]
                  }
                }
                n1327 = Select(t="ON" ("format string"), s=w2473, f="OFF" ("format string")) -> (s? t:f=w2470:string)
                n1328 = call "util.procs.find-by-name.vi"("error in"=w2467, "ProcName in"=w2463, "Procs in"=w2464) -> ("error out"=w2466:errorcluster, "Found?"=w2476:bool, "procIndex"=w2477:i32)  [unwired: 3 in, 3 out]
                n1329 = Format Into String(format string=w2474, w2462, w2470) -> (resulting string=w2469:string)  [unwired: 2 in, 1 out]
                n1330 = call "proc.util.enumToStrProcVar.vi"("Proc var"=typeProcVarientName."procRegisterString" ("Combo Box")) -> ("String"=w2480:string)  [unwired: 10 in]
                n1331 = Merge Errors(w2466) -> (w2465:errorcluster)
                n1332 = case shown="True" w2476 {
                  tunnel: [w2489 w2497] -> w2478
                  tunnel: w2464 -> [w2489 w2496]
                  tunnel: w2480 -> [_ w2491]
                  tunnel: w2477 -> [_ w2492]
                  tunnel: [w2488 w2495] -> w2475
                  tunnel: w2465 -> [w2488 w2494]
                  tunnel: w2469 -> [_ w2490]
                  frame False {
                  }
                  frame True {
                    n1333 = call "procs.setByProcIndexString.vi"("menu in (get)"=enum16{"get", "set"}."set", "procIndex"=w2492, "error in"=w2494, "String in"=w2490, "procAttribute"=w2491, "procs in"=w2496) -> ("error out"=w2495:errorcluster, "procs out"=w2497:cluster{"Procedure":variant[]}[])  [unwired: 3 in, 1 out]
                  }
                }
              }
              frame "ENG.PROC.PRESET" {
                # "\"ENG.PROC.PRESET\" copy template as procedure (used to change device modes)"
                n1334 = disable-structure shown="Enabled" {
                  disable-tunnel: w2511 -> [w2527 _]
                  disable-tunnel: w2510 -> [w2525 _]
                  disable-tunnel: [w2520 _] -> w2508
                  frame Disabled {
                    # "procedure can be configured to reset itself every completion or be reset immidiatly"
                    n1335 = local read item#-1() -> (w2523)
                    n1336 = Variant To Data(type=w2523, Variant=w2527) -> (data=w2526, error out=w2518:errorcluster)  [unwired: 1 in]
                    n1337 = Unbundle By Name(w2526) -> ("Immidiate"=w2524, "ProcName"=w2514, "Preset File"=w2517)
                    n1338 = call "util.file.vars.vi"("error in"=w2518, "Directory (DIR_PROC)"=typePathSelector."DIR_TEMPLATE" ("Enum"), "Proc Name(open dialog if empty)"=w2517) -> ("error out"=w2513:errorcluster, "Vars[] out"=w2516:variant[])  [unwired: 4 in, 3 out]
                    n1339 = call "util.proc.set-name.vi"("error in"=w2513, "new Proc Name"=w2514, "Procedure in"=w2516) -> ("error out"=w2512:errorcluster, "Procedure out"=w2515:variant[])  [unwired: 7 in]
                    n1340 = call "util.file.vars.vi"("Operation(Read)"=enum16{"Read File", "Write File"}."Write File", "error in"=w2512, "Proc Name(open dialog if empty)"=w2514, "Vars[] in"=w2515) -> ("error out"=w2519:errorcluster)  [unwired: 3 in, 4 out]
                    n1341 = case shown="True" w2524 {
                      tunnel: w2525 -> [_ w2535]
                      tunnel: w2514 -> [_ w2532]
                      tunnel: [w2528 w2530] -> w2520
                      tunnel: w2519 -> [w2528 w2529]
                      frame False {
                      }
                      frame True {
                        n1342 = To Variant(anything=w2532) -> (Variant=w2531:variant)
                        n1343 = Bundle By Name(cluster=cluster{"cmd":T5, "data":variant} {"cmd"=enum."ENG.PROC.RELOAD-BY-NAME", "data"=variant} ("typedefElement"), "data"=w2531) -> (w2534:cluster{"cmd":T5, "data":variant})
                        n1344 = Enqueue Element At Opposite End(queue=w2535, element=w2534, error in (no error)=w2529) -> (error out=w2530:errorcluster)  [unwired: 1 in, 2 out]
                      }
                    }
                  }
                  frame Enabled {
                  }
                }
              }
              frame "ENG.PROC.RELOAD-BY-NAME" {
                w2552 = ""  # procedureName
                # "(3)"
                # "(2)"
                # "(1)"
                # "\"ENG.PROC.RELOAD-BY-NAME\"  (PROCEDURE_NAME)\n(1) SEARCH PROC BY NAME (IN RUNTIME), GET ITS INDEX AND PATH\n(2) LOAD PROCEDURE FROM STORAGE AND INITIALIZE IT\n(3) REPLACE ORIGINAL PROC"
                n1345 = Variant To Data(type=w2552, Variant=w2553) -> (data=w2541:string, error out=w2537:errorcluster)  [unwired: 1 in]
                n1346 = call "util.procs.find-by-name.vi"("isRequired(T)"=FALSE, "error in"=w2537, "ProcName in"=w2541, "Procs in"=w2547) -> ("error out"=w2536:errorcluster, "Found?"=w2545:bool, "procIndex"=w2546:i32, "Proc Path"=w2542:string)  [unwired: 2 in, 2 out]
                n1347 = String To Path(string=w2542) -> (path=w2543:path)
                n1348 = call "util.file.vars.file-operations.vi"("error in (no error)"=w2536, "selected path"=w2543) -> ("error out"=w2549:errorcluster, "Procedure"=w2550:variant[])  [unwired: 7 in, 1 out]
                n1349 = call "util.proc.init.vi"("error in"=w2549, "Proc Path"=w2543, "Procedure in"=w2550) -> ("error out"=w2540:errorcluster, "Procedure out"=w2551:variant[])  [unwired: 7 in]
                n1350 = Bundle("Procedure out"=w2551) -> (w2544:cluster{"Procedure out":variant[]})  [unwired: 1 in]
                n1351 = case shown="No Error" w2540 {
                  selector: w2540 -> [_ w2559]
                  tunnel: [w2557 w2558] -> w2548
                  tunnel: w2547 -> [w2556 w2558]
                  tunnel: w2546 -> [w2555 _]
                  tunnel: w2544 -> [w2554 _]
                  tunnel: w2545 -> [_ _]
                  tunnel: [_ w2559] -> w2539
                  frame No Error {
                    n1352 = Replace Array Subset(array=w2556, new element=w2554, index=w2555) -> (w2557:cluster{"Procedure":variant[]}[])
                  }
                  frame Error {
                  }
                }
              }
              frame "ENG.PROC.START" {
                # "\"ENG-PROC.START\"  find proc and set its procIsRuning attribute"
                n1353 = Variant To Data(type="" ("procName"), Variant=w2569) -> (data=w2560:string)  [unwired: 1 in, 1 out]
                n1354 = Bundle By Name(cluster=T93 {"operation"=enum."START", "procName"=""}, "procName"=w2560) -> (w2563:T93)
                n1355 = call "main.eng.proc-start.vi"("params in"=w2563, "Procs in"=w2567) -> ("error out"=w2566:errorcluster, "Procs out"=w2568:cluster{"Procedure":variant[]}[])  [unwired: 7 in, 1 out]
                n1356 = Format Into String(format string="Start Procedure %s", w2560) -> (resulting string=w2561:string)  [unwired: 2 in, 1 out]
              }
              frame "ENG.PROC.STOP" {
                # "\"ENG-PROC.START\"  find proc and set its procIsRuning attribute"
                n1357 = Variant To Data(type="" ("procName"), Variant=w2579) -> (data=w2570:string)  [unwired: 1 in, 1 out]
                n1358 = Bundle By Name(cluster=T93 {"operation"=enum."STOP", "procName"=""}, "procName"=w2570) -> (w2573:T93)
                n1359 = call "main.eng.proc-start.vi"("params in"=w2573, "Procs in"=w2577) -> ("error out"=w2576:errorcluster, "Procs out"=w2578:cluster{"Procedure":variant[]}[])  [unwired: 7 in, 1 out]
                n1360 = Format Into String(format string="Stop Procedure %s", w2570) -> (resulting string=w2571:string)  [unwired: 2 in, 1 out]
              }
              frame "ENG.RIO.SNAPSHOT" {
                # "\"ENG.RIO.SNAPSHOT\""
                n1361 = Variant To Data(type=u8[] [], Variant=w2586) -> (error out=w2583:errorcluster)  [unwired: 1 in, 1 out]
                n1362 = call <vilib>:"Clear Errors.vi"("error in (no error)"=w2583) -> ()  [unwired: 5 in, 2 out]
                n1363 = local read "RIO List"() -> (w2581:cluster{"Address":u8, "Connected":bool}[])
                n1364 = call "helper-snapshot.vi"("RIO List"=w2581) -> ("Snapshot"=w2582:T13[])  [unwired: 10 in]
                "RIO Snapshots" <- w2582
                n1365 = for {
                  tunnel: w2582 -> [w2593] mode=indexing
                  tunnel: w2581 -> [w2592] mode=indexing
                  tunnel: [w2591] -> w2580 mode=indexing
                  workers-P: _ -> [_]
                  n1366 = Unbundle By Name(w2593) -> ("status.status"=w2590:bool)
                  n1367 = Not(x=w2590) -> (.not. x?=w2589:bool)
                  n1368 = in-place {
                    in-place-border: w2589 -> [w2594]
                    n1369 = in-place-cluster #5(w2592) -> ()  [unwired: 1 out]
                    n1370 = in-place-cluster #5("Connected"=w2594) -> (w2591:cluster{"Address":u8, "Connected":bool})
                  }
                }
                n1371 = disable-structure shown="Enabled" {
                  disable-tunnel: w2582 -> [w2596 _]
                  disable-tunnel: [w2595 _] -> w2587
                  frame Enabled {
                    n1372 = global read "globals-engine.vi" "Q-Log"() -> (w2597:refnum<queue>)
                    n1373 = Bundle By Name(cluster=cluster{"data":variant, "Enum":T57} {"data"=variant, "Enum"=enum."LOG.SNAPSHOT"} ("procQ"), "data"=w2596) -> (w2599:cluster{"data":variant, "Enum":T57})
                    n1374 = Enqueue Element(queue=w2597, element=w2599) -> (error out=w2598:errorcluster)  [unwired: 2 in, 2 out]
                    n1375 = call <vilib>:"Clear Errors.vi"("error in (no error)"=w2598) -> ("error out"=w2595:errorcluster)  [unwired: 5 in, 1 out]
                  }
                  frame Disabled {
                  }
                }
                n1376 = local write "RIO List"(w2580) -> ()
              }
              frame "ENG.RIO.AIN-SNAPSHOT-CALIB" {
                # "\"ENG.RIO.READ-AIN\"  (RIO_ADDRESS)\nREAD ALL ANALOG INPUTS OF A RIO"
                n1377 = local read "IO calib select"() -> (w2606:string)
                n1378 = call "io.interface.vi"("Caller"="ENG.RIO.AIN-SNAPSHOT-CALIB", "IO Name in"=w2606) -> ("error out"=→"error":errorcluster, "unCalibrated"=w2603:u16, "Value out"=w2602:dbl)  [unwired: 4 in, 3 out]
                "Raw (X)" <- w2603
                "Value (Y)" <- w2602
                n1379 = Bundle("unCalibrated"=w2603, "Value out"=w2602) -> (→"Chart":cluster{"unCalibrated":u16, "Value out":dbl})  [unwired: 1 in]
              }
              frame "ENG.RIO.DOUT-BY-ADDR" {
                # "\"ENG.RIO.READ-AIN\"  (RIO_ADDRESS)\nREAD ALL ANALOG INPUTS OF A RIO"
                n1380 = Variant To Data(type=cluster{"State":bool, "ADDR":T8, "Timeout":u8} {"State"=FALSE, "ADDR"=8, "Timeout"=8} ("digitalPort"), Variant=w2632) -> (data=w2624:cluster{"State":bool, "ADDR":T8, "Timeout":u8})  [unwired: 1 in, 1 out]
                n1381 = Unbundle By Name(w2624) -> ("ADDR"=w2611:T8, "State"=w2612:bool, "Timeout"=w2628:u8)
                n1382 = Bundle By Name(cluster=cluster{"state":bool, "timeoutSeconds":u16} {"state"=FALSE, "timeoutSeconds"=0} ("output cluster"), "state"=w2612, "timeoutSeconds"=w2628) -> (w2629:cluster{"state":bool, "timeoutSeconds":u16})
                n1383 = Bundle By Name(cluster=T42 {"ADDR"=2, "Label"="", "Type"=enum."DO", "Mode"=enum."RIO", "Value"="1:1", "Tags"="", "calibration"=[]} ("IoConf in 2"), "Type"=enum.io.type."DO" ("type"), "ADDR"=w2611) -> (w2627:T42)
                n1384 = To Variant(anything=w2629) -> (Variant=w2625:variant)
                n1385 = call "io.interface.serial.vi"("IoConf in"=w2627, "Caller"="ENG.RIO.DOUT-BY-ADDR", "Output State"=w2625) -> ("error out"=w2622:errorcluster)  [unwired: 7 in, 5 out]
                n1386 = disable-structure shown="Enabled" {
                  disable-tunnel: w2622 -> [w2635 w2638]
                  disable-tunnel: [w2634 w2638] -> w2613
                  frame Disabled {
                    n1387 = global read "globals-engine.vi" "Q-Eng"() -> (w2637:refnum<queue>)
                    n1388 = Enqueue Element(queue=w2637, element=cluster{"case":T5, "data":variant} {"case"=enum."ENG.RIO.SNAPSHOT", "data"=variant}, error in (no error)=w2635) -> (error out=w2634:errorcluster)  [unwired: 1 in, 2 out]
                  }
                  frame Enabled {
                  }
                }
                n1389 = Select(t="Set DO " ("format string"), s=w2612, f="Clear DO " ("format string")) -> (s? t:f=w2614:string)
                n1390 = property on="Timer Reset?" class="Bool (strict)"("Val(Sgnl)"=TRUE ("Value (Signaling)")) -> ()  [unwired: 2 in, 2 out]
                n1391 = Format Into String(format string=" %04d", w2611) -> (resulting string=w2615:string)  [unwired: 2 in, 1 out]
                n1392 = Select(t="Error " ("format string"), s=w2613, f="" ("format string")) -> (s? t:f=w2618:string)
                n1393 = Concatenate Strings(w2618, w2614, w2615) -> (w2610:string)
              }
              frame "ENG.RIO.DOUT-BY-NAME" {
                # "\"ENG.RIO.READ-AIN\"  (RIO_ADDRESS)\nREAD ALL ANALOG INPUTS OF A RIO"
                n1394 = Variant To Data(type=T94 {"State"=FALSE, "Timeout"=0, "Name"=""} ("Cluster"), Variant=w2658) -> (data=w2655:T94)  [unwired: 1 in, 1 out]
                n1395 = Unbundle By Name(w2655) -> ("Name"=w2641:string, "State"=w2644:bool, "Timeout"=w2654:u16)
                n1396 = Select(t="Set DO " ("format string"), s=w2644, f="Clear DO " ("format string")) -> (s? t:f=w2643:string)
                n1397 = Bundle By Name(cluster=cluster{"state":bool, "timeoutSeconds":u16} {"state"=FALSE, "timeoutSeconds"=0} ("output cluster"), "state"=w2644, "timeoutSeconds"=w2654) -> (w2653:cluster{"state":bool, "timeoutSeconds":u16})
                n1398 = To Variant(anything=w2653) -> (Variant=w2657:variant)
                n1399 = call "io.interface.vi"("Caller"="ENG.RIO.DOUT-BY-NAME", "IO Value"=w2657, "IO Name in"=w2641) -> ("error out"=w2648:errorcluster)  [unwired: 3 in, 5 out]
                n1400 = Select(t="Error " ("format string"), s=w2648, f="" ("format string")) -> (s? t:f=w2647:string)
                n1401 = disable-structure shown="Enabled" {
                  disable-tunnel: w2648 -> [w2661 w2665]
                  disable-tunnel: [w2660 w2664] -> w2651
                  frame Disabled {
                    n1402 = global read "globals-engine.vi" "Q-Eng"() -> (w2663:refnum<queue>)
                    n1403 = Enqueue Element(queue=w2663, element=cluster{"case":T5, "data":variant} {"case"=enum."ENG.RIO.SNAPSHOT", "data"=variant}, error in (no error)=w2661) -> (error out=w2660:errorcluster)  [unwired: 1 in, 2 out]
                  }
                  frame Enabled {
                    n1404 = call <vilib>:"Clear Errors.vi"("error in (no error)"=w2665) -> ("error out"=w2664:errorcluster)  [unwired: 5 in, 1 out]
                  }
                }
                n1405 = Concatenate Strings(w2647, w2643, w2641) -> (w2642:string)
                n1406 = property on="Timer Reset?" class="Bool (strict)"("Val(Sgnl)"=TRUE ("Value (Signaling)")) -> ()  [unwired: 2 in, 2 out]
              }
              frame "ENG.RIO.RFS-DELAY-SET-X8" {
                n1407 = local read "RFS Delays"() -> (w2667:T35)
                n1408 = for {
                  N: 8 -> [_]
                  tunnel: [w2673] -> w2669
                  tunnel: w2667 -> [w2672]
                  tunnel: "RFS Address" -> [w2671]
                  i -> [w2674]
                  stop <- w2673 stop-if-true
                  w2681 = u8 5  # Datasize
                  w2682 = u8 96  # Command
                  w2692 = "%s RIO[%d] %s %s"  # TIME RIO[i] OPERATION STATUS
                  w2695 = T42 {"ADDR"=0, "Label"="", "Type"=enum."Type", "Mode"=enum."RIO", "Value"="", "Tags"="", "calibration"=[]}  # IoConf in 2
                  n1409 = Unbundle By Name(w2672) -> ("Delay Y"=w2683:u8, "Delay X1"=w2684:u8, "Delay X2"=w2685:u8, "Delay CT"=w2686:u8)
                  n1410 = Bundle(cluster=T95 {"DataSize"=0, "Address"=0, "CMD"=0, "Table Index"=0, "Delay Y"=0, "Delay X1"=0, "Delay X2"=0, "Delay CT"=0}, "DataSize"=w2681, "Address"=w2671, "CMD"=w2682, "Table Index"=w2674, "Delay Y"=w2683, "Delay X1"=w2684, "Delay X2"=w2685, "Delay CT"=w2686) -> (w2680:T95)
                  n1411 = Flatten To String(anything=w2680) -> (data string=w2679:string, error out=w2678:errorcluster)  [unwired: 3 in, 1 out]
                  n1412 = Format Into String(format string="Set Delays for Table[%d]", w2674) -> (resulting string=w2675:string)  [unwired: 2 in, 1 out]
                  n1413 = call "io.frame.vi"("error in"=w2678, "Frameless Command"=w2679) -> ("error out"=w2699:errorcluster, "Framed Command"=w2700:string)  [unwired: 8 in]
                  n1414 = call "io.visa.vi"("operation in (wr-rd)"=enum.io-interface."IO_VISA_WR-RD" ("operation"), "preReadMsDelay"=u32 150, "error in (no error)"=w2699, "write buffer"=w2700) -> ("error out"=w2698:errorcluster, "read buffer"=w2696:string)  [unwired: 4 in, 2 out]
                  n1415 = call "io.responseValidator.vi"("error in"=w2698, "ResponsToValidate in"=w2696, "IoConf in 2"=w2695) -> ("error out"=w2673:errorcluster)  [unwired: 7 in, 1 out]
                  n1416 = Select(t="Failed", s=w2673, f="Succeeded ") -> (s? t:f=w2677:string)
                  n1417 = Get Date/Time String(want seconds? (F)=TRUE) -> (time string=w2691:string)  [unwired: 2 in, 1 out]
                  n1418 = Format Into String(format string=w2692, w2691, w2671, w2675, w2677) -> (resulting string=w2688:string)  [unwired: 2 in, 1 out]
                  n1419 = local write "RFS Status"(w2688) -> ()
                }
              }
              frame "ENG.RIO.RFS-DELAY-SET-X1" {
                w2711 = u8 5  # Datasize
                w2712 = u8 96  # Command
                w2721 = "%s RIO[%d] %s %s"  # TIME RIO[i] OPERATION STATUS
                w2724 = T42 {"ADDR"=0, "Label"="", "Type"=enum."Type", "Mode"=enum."RIO", "Value"="", "Tags"="", "calibration"=[]}  # IoConf in 2
                n1420 = local read "RFS Address"() -> (w2707:u8)
                n1421 = local read "TableIndex"() -> (w2703:u8)
                n1422 = Unbundle By Name("RFS Delays") -> ("Delay Y"=w2713:u8, "Delay X1"=w2714:u8, "Delay X2"=w2715:u8, "Delay CT"=w2716:u8)
                n1423 = Bundle(cluster=T95 {"DataSize"=0, "Address"=0, "CMD"=0, "Table Index"=0, "Delay Y"=0, "Delay X1"=0, "Delay X2"=0, "Delay CT"=0}, "DataSize"=w2711, "Address"=w2707, "CMD"=w2712, "Table Index"=w2703, "Delay Y"=w2713, "Delay X1"=w2714, "Delay X2"=w2715, "Delay CT"=w2716) -> (w2710:T95)
                n1424 = Flatten To String(anything=w2710) -> (data string=w2709:string, error out=w2708:errorcluster)  [unwired: 3 in, 1 out]
                n1425 = Format Into String(format string="Set Delays for Table[%d]", w2703) -> (resulting string=w2704:string)  [unwired: 2 in, 1 out]
                n1426 = call "io.frame.vi"("error in"=w2708, "Frameless Command"=w2709) -> ("error out"=w2728:errorcluster, "Framed Command"=w2729:string)  [unwired: 8 in]
                n1427 = call "io.visa.vi"("operation in (wr-rd)"=enum.io-interface."IO_VISA_WR-RD" ("operation"), "preReadMsDelay"=u32 150, "error in (no error)"=w2728, "write buffer"=w2729) -> ("error out"=w2727:errorcluster, "read buffer"=w2725:string)  [unwired: 4 in, 2 out]
                n1428 = call "io.responseValidator.vi"("error in"=w2727, "ResponsToValidate in"=w2725, "IoConf in 2"=w2724) -> ("error out"=w2730:errorcluster)  [unwired: 7 in, 1 out]
                n1429 = Select(t="Failed", s=w2730, f="Succeeded ") -> (s? t:f=w2706:string)
                n1430 = Get Date/Time String(want seconds? (F)=TRUE) -> (time string=w2720:string)  [unwired: 2 in, 1 out]
                n1431 = Format Into String(format string=w2721, w2720, w2707, w2704, w2706) -> (resulting string=→"RFS Status":string)  [unwired: 2 in, 1 out]
              }
              frame "ENG.RIO.RFS-CYCLES-GET" {
                w2738 = u16 0  # u16
                w2748 = u8 0  # Datasize
                w2749 = u8 97  # Command
                w2755 = "%s RIO[%d] %s %s"  # TIME RIO[i] OPERATION STATUS
                n1432 = local read "RFS Address"() -> (w2744:u8)
                n1433 = Bundle(cluster=cluster{"DataSize":u8, "Address":u8, "CMD":u8} {"DataSize"=0, "Address"=0, "CMD"=0}, "DataSize"=w2748, "Address"=w2744, "CMD"=w2749) -> (w2747:cluster{"DataSize":u8, "Address":u8, "CMD":u8})
                n1434 = Flatten To String(anything=w2747) -> (data string=w2746:string, error out=w2745:errorcluster)  [unwired: 3 in, 1 out]
                n1435 = call "io.frame.vi"("error in"=w2745, "Frameless Command"=w2746) -> ("error out"=w2762:errorcluster, "Framed Command"=w2763:string)  [unwired: 8 in]
                n1436 = call "io.visa.vi"("operation in (wr-rd)"=enum.io-interface."IO_VISA_WR-RD" ("operation"), "preReadMsDelay"=u32 150, "error in (no error)"=w2762, "write buffer"=w2763) -> ("error out"=w2761:errorcluster, "read buffer"=w2759:string)  [unwired: 4 in, 2 out]
                n1437 = call "io.responseValidator.vi"("error in"=w2761, "ResponsToValidate in"=w2759, "IoConf in 2"=T42 {"ADDR"=0, "Label"="", "Type"=enum."Type", "Mode"=enum."RIO", "Value"="", "Tags"="", "calibration"=[]}) -> ("error out"=w2735:errorcluster, "Data out"=w2737:string)  [unwired: 7 in]
                n1438 = Unflatten From String(type=w2738, binary string=w2737, data includes array or string size? (T)=FALSE, error in (no error)=w2735) -> (rest of the binary string=w2739:string, value=→"RFS Cycles":u16, error out=w2740:errorcluster)  [unwired: 1 in]
                n1439 = Select(t="Failed", s=w2735, f="Succeeded ") -> (s? t:f=w2743:string)
                n1440 = for {
                  N: 8 -> [_]
                  shift-right: [w2769] -> _
                  shift-left: w2739 -> [w2771]
                  shift-right: [w2766] -> _
                  shift-left: w2740 -> [w2767]
                  tunnel: [w2765] -> w2734 mode=indexing
                  n1441 = Unflatten From String(type=u16 0, binary string=w2771, data includes array or string size? (T)=FALSE, error in (no error)=w2767) -> (rest of the binary string=w2769:string, value=w2765:u16, error out=w2766:errorcluster)  [unwired: 1 in]
                }
                n1442 = Get Date/Time String(want seconds? (F)=TRUE) -> (time string=w2754:string)  [unwired: 2 in, 1 out]
                n1443 = Format Into String(format string=w2755, w2754, w2744, "Get Cycles" ("format string"), w2743) -> (resulting string=w2751:string)  [unwired: 2 in, 1 out]
                n1444 = Array To Cluster(array=w2734) -> (cluster=→"RFS Cycles Table":T36)
                n1445 = local write "RFS Status"(w2751) -> ()
              }
              frame "ENG.RIO.RFS-ENABLE" {
                (unwired) FALSE ("data includes array or string size? (T)")
                w2787 = u8 1  # Datasize
                w2788 = u8 99  # Command
                w2794 = "%s RIO[%d] %s %s"  # TIME RIO[i] OPERATION STATUS
                (unwired) 8
                n1446 = local read "RFS Address"() -> (w2778:u8)
                n1447 = Cluster To Array(cluster="RFS Enable Table") -> (array=w2777:bool[])
                n1448 = Boolean Array To Number(Boolean array=w2777) -> (number=w2780:u32)
                n1449 = for {
                  tunnel: w2777 -> [w2804] mode=indexing
                  tunnel: [w2805] -> w2776 mode=indexing if=w2804
                  i -> [w2805]
                }
                n1450 = To Unsigned Byte Integer(number=w2780) -> (unsigned 8bit integer=w2779:u8)
                n1451 = Bundle(cluster=T96 {"DataSize"=0, "Address"=0, "CMD"=0, "Enable"=0}, "DataSize"=w2787, "Address"=w2778, "CMD"=w2788, "Enable"=w2779) -> (w2786:T96)
                n1452 = Number To Decimal String(number=w2776) -> (decimal integer string=w2775:string[])  [unwired: 1 in]
                n1453 = call "util.DelimitedStringFromArray.vi"("params array in"=w2775) -> ("delimited string out"=w2772:string)  [unwired: 10 in]
                n1454 = Flatten To String(anything=w2786) -> (data string=w2785:string, error out=w2784:errorcluster)  [unwired: 3 in, 1 out]
                n1455 = call "io.frame.vi"("error in"=w2784, "Frameless Command"=w2785) -> ("error out"=w2801:errorcluster, "Framed Command"=w2802:string)  [unwired: 8 in]
                n1456 = call "io.visa.vi"("operation in (wr-rd)"=enum.io-interface."IO_VISA_WR-RD" ("operation"), "preReadMsDelay"=u32 150, "error in (no error)"=w2801, "write buffer"=w2802) -> ("error out"=w2800:errorcluster, "read buffer"=w2798:string)  [unwired: 4 in, 2 out]
                n1457 = Format Into String(format string="Enable Tables[%s]", w2772) -> (resulting string=w2773:string)  [unwired: 2 in, 1 out]
                n1458 = call "io.responseValidator.vi"("error in"=w2800, "ResponsToValidate in"=w2798, "IoConf in 2"=T42 {"ADDR"=0, "Label"="", "Type"=enum."Type", "Mode"=enum."RIO", "Value"="", "Tags"="", "calibration"=[]}) -> ("error out"=w2782:errorcluster)  [unwired: 7 in, 1 out]
                n1459 = Select(t="Failed", s=w2782, f="Succeeded ") -> (s? t:f=w2783:string)
                n1460 = Get Date/Time String(want seconds? (F)=TRUE) -> (time string=w2793:string)  [unwired: 2 in, 1 out]
                n1461 = Format Into String(format string=w2794, w2793, w2778, w2773, w2783) -> (resulting string=w2790:string)  [unwired: 2 in, 1 out]
                n1462 = local write "RFS Status"(w2790) -> ()
              }
              frame "ENG.RIO.RFS-CYCLES-SET" {
                w2814 = u8 2  # Datasize
                w2815 = u8 98  # Command
                w2821 = "%s RIO[%d] %s %s"  # TIME RIO[i] OPERATION STATUS
                w2824 = T42 {"ADDR"=0, "Label"="", "Type"=enum."Type", "Mode"=enum."RIO", "Value"="", "Tags"="", "calibration"=[]}  # IoConf in 2
                (unwired) 8
                n1463 = local read "RFS Cycles"() -> (w2806:u16)
                n1464 = local read "RFS Address"() -> (w2810:u8)
                n1465 = Bundle(cluster=T97 {"DataSize"=0, "Address"=0, "CMD"=0, "Cycles"=0}, "DataSize"=w2814, "Address"=w2810, "CMD"=w2815, "Cycles"=w2806) -> (w2813:T97)
                n1466 = Flatten To String(anything=w2813) -> (data string=w2812:string, error out=w2811:errorcluster)  [unwired: 3 in, 1 out]
                n1467 = Format Into String(format string="Limit Cycles to %d", w2806) -> (resulting string=w2807:string)  [unwired: 2 in, 1 out]
                n1468 = call "io.frame.vi"("error in"=w2811, "Frameless Command"=w2812) -> ("error out"=w2828:errorcluster, "Framed Command"=w2829:string)  [unwired: 8 in]
                n1469 = call "io.visa.vi"("operation in (wr-rd)"=enum.io-interface."IO_VISA_WR-RD" ("operation"), "preReadMsDelay"=u32 150, "error in (no error)"=w2828, "write buffer"=w2829) -> ("error out"=w2827:errorcluster, "read buffer"=w2825:string)  [unwired: 4 in, 2 out]
                n1470 = call "io.responseValidator.vi"("error in"=w2827, "ResponsToValidate in"=w2825, "IoConf in 2"=w2824) -> ("error out"=w2830:errorcluster)  [unwired: 7 in, 1 out]
                n1471 = Select(t="Failed", s=w2830, f="Succeeded ") -> (s? t:f=w2809:string)
                n1472 = Get Date/Time String(want seconds? (F)=TRUE) -> (time string=w2820:string)  [unwired: 2 in, 1 out]
                n1473 = Format Into String(format string=w2821, w2820, w2810, w2807, w2809) -> (resulting string=w2817:string)  [unwired: 2 in, 1 out]
                n1474 = local write "RFS Status"(w2817) -> ()
              }
              frame "ENG.NO-OP", Default {
              }
            }
            n1475 = call "helper-log-eng.vi"("error in"=w2042, "ARGS"=w2041, "case"=w2044) -> ("error out"=w2043:errorcluster, "Collected Reports"=→"Collected Reports":string)  [unwired: 7 in]
          }
        }
      }
      frame Error {
        # "handle error by displaying a continue/stop message dialog."
        n1476 = call <vilib>:"Clear Errors.vi"("error in (no error)"=w2835) -> ("error out"=w2836:errorcluster)  [unwired: 5 in, 1 out]
        n1477 = Unbundle By Name(w2835) -> ("source"=w2834:string)
      }
    }
    n1478 = case shown="Default" w1960 {
      selector: w1960 -> [_ w1975]
      frame "" {
        # "skip empty statuts"
      }
      frame Default {
        # "status register"
        n1479 = call "reg-status.vi"("Operation(Read)"=enum.report-filter."Collect", "Reports to Collect"=w1975) -> ("Collected Reports"=→"User messages":string)  [unwired: 8 in, 1 out]
      }
    }
    n1480 = call "util-collect-error.vi"("error in (no error)"=w1954, "Array in"=w1955) -> ("Array out"=w1953:errorcluster[])  [unwired: 9 in]
    "VM Engine Errors" <- w1953
    n1481 = disable-structure shown="Enabled" {
      disable-tunnel: w1956 -> [w1973 _]
      disable-tunnel: [w1972 _] -> w1951
      frame Enabled {
        n1482 = call "eng-error-handler.vi"("Numeric"=w1973) -> ("delta t"=w1972:dbl)  [unwired: 9 in, 1 out]
      }
      frame Disabled {
      }
    }
    "Waveform Chart 3" <- w1951
    n1483 = property on="Waveform Chart" class="WFChart (strict)"("Value"=w1951) -> ()  [unwired: 2 in, 2 out]
    "Eng" <- w1962
  }
  n1484 = Merge Errors(w36) -> (w14:errorcluster)
  n1485 = call <vilib>:"Clear Errors.vi"("error in (no error)"=w14) -> ("error out"=w35:errorcluster)  [unwired: 5 in, 1 out]
  n1486 = call "io.visa.vi"("operation in (wr-rd)"=enum.io-interface."IO_VISA_CLOSE", "error in (no error)"=w35) -> ("error out"=w34:errorcluster)  [unwired: 6 in, 3 out]
  n1487 = disable-structure shown="Enabled" {
    frame Disabled {
      n1488 = feedback #6() -> (w2838)  [unwired: 1 in]
      n1489 = feedback-in #6() -> (w2842)
      n1490 = local write "IO Map AI"(w2842) -> ()
      n1491 = Not Equal?(x=w2842, y=w2838) -> (x != y?=w2843:bool)
      n1492 = Array Max & Min(array=w2843) -> (max index (indices)=w2840:i32, min index (indices)=w2839:i32)  [unwired: 2 out]
      n1493 = Not Equal?(x=w2840, y=w2839) -> (x != y?=w2841:bool)
      n1494 = case shown="True" w2841 {
        tunnel: w2842 -> [_ w2844]
        frame False {
        }
        frame True {
          n1495 = local write "IO Map AI"(w2844) -> ()
        }
      }
    }
    frame Enabled {
    }
  }
  n1496 = call <vilib>:"Clear Errors.vi"("error in (no error)"=w34) -> ("error out"=w24:errorcluster)  [unwired: 5 in, 1 out]
  n1497 = property on="Splitter" class="Splitter"(error in=w24, "Locked"=FALSE ("Splitter Position Locked")) -> ()  [unwired: 1 in, 2 out]
